vi "Lab Panel V3.4.vi"() -> ()   [LabVIEW 2013]
uses:
  <vilib>/Platform/TimedLoop/XDataNode/timing_clust.ctl
  <vilib>/Platform/TimedLoop/XDataNode/nitl_modes.ctl
  <vilib>/Platform/TimedLoop/XDataNode/wakeup.ctl
  Global 1.vi
  <vilib>/platform/TimedLoop/XDataNode/XDataNode.xnode
  <vilib>/Platform/TimedLoop/XDataNode/XDNodeRunTimeDep.lvlib
panel:
  out "TEMP update":bool
  out "AI update":bool
  in  "stop":bool
  in  "Tab Control 2":T1(tab)
  out "SIG LAB05-2":T2 {"PF" format="%.2f"; "AMPS" format="%.1f"}
  out "SIG LAB05-1":T2 {"PF" format="%.2f"; "AMPS" format="%.1f"}
  out "SIG LAB04-2":T2 {"PF" format="%.2f"; "AMPS" format="%.1f"}
  out "SIG LAB04-1":T2 {"PF" format="%.2f"; "AMPS" format="%.1f"}
  out "SIG LAB03-2":T2 {"PF" format="%.2f"; "AMPS" format="%.1f"}
  out "SIG LAB03-1":T2 {"PF" format="%.2f"; "AMPS" format="%.1f"}
  out "SIG LAB02-2":T2 {"PF" format="%.2f"; "AMPS" format="%.1f"}
  in  "RUN LAB01-1":bool
  in  "O/I  LAB05-1":bool
  in  "O/I  LAB05-2":bool
  in  "O/I  LAB04-1":bool
  in  "O/I  LAB04-2":bool
  in  "O/I  LAB02-1":bool
  in  "O/1  LAB02-2":bool
  in  "O/I  LAB01-2":bool
  in  "O/I  LAB01-1":bool
  in  "O/I  LAB03-1":bool
  in  "RUN LAB05-2":bool
  in  "RUN LAB05-1":bool
  in  "RUN LAB04-2":bool
  in  "RUN LAB04-1":bool
  in  "RUN LAB03-2":bool
  in  "RUN LAB03-1":bool
  in  "RUN LAB02-2":bool
  in  "RUN LAB02-1":bool
  in  "RUN LAB01-2":bool
  in  "SELECT LAB05-2":T3(radio)
  in  "SELECT LAB05-1":T3(radio)
  in  "SELECT LAB04-2":T3(radio)
  in  "SELECT LAB04-1":T3(radio)
  in  "SELECT LAB03-2":T3(radio)
  in  "SELECT LAB03-1":T3(radio)
  in  "SELECT LAB02-2":T3(radio)
  in  "SELECT LAB02-1":T3(radio)
  in  "SELECT LAB01-2":T3(radio)
  in  "SELECT LAB01-1":T3(radio)
  in  "O/I  LAB03-2":bool
  out "SIG LAB01-1":T2 {"PF" format="%.2f"; "AMPS" format="%.1f"}
  out "SIG LAB01-2":T2 {"PF" format="%.2f"; "AMPS" format="%.1f"}
  out "SIG LAB02-1":T2 {"PF" format="%.2f"; "AMPS" format="%.1f"}
  out "DISP LAB05-2":T4 {"MINS" format="%.2g"}
  out "DISP LAB05-1":T4 {"MINS" format="%.2g"}
  out "DISP LAB04-2":T4 {"MINS" format="%.2g"}
  out "DISP LAB04-1":T4 {"MINS" format="%.2g"}
  out "DISP LAB03-2":T4 {"MINS" format="%.2g"}
  out "DISP LAB03-1":T4 {"MINS" format="%.2g"}
  in  "SET LAB05-2":T5={"NAME"="", "DESCRIPTION"="", "CYCLES"=5.0, "T-RISE mins"=0.0, "T-RISE deg C"=0.0} {"CYCLES" min=5.0 step=1.0}
  in  "SET LAB05-1":T5={"NAME"="", "DESCRIPTION"="", "CYCLES"=5.0, "T-RISE mins"=0.0, "T-RISE deg C"=0.0} {"CYCLES" min=5.0 step=1.0}
  in  "SET LAB04-2":T5={"NAME"="", "DESCRIPTION"="", "CYCLES"=5.0, "T-RISE mins"=0.0, "T-RISE deg C"=0.0} {"CYCLES" min=5.0 step=1.0}
  in  "SET LAB04-1":T5={"NAME"="", "DESCRIPTION"="", "CYCLES"=5.0, "T-RISE mins"=0.0, "T-RISE deg C"=0.0} {"CYCLES" min=5.0 step=1.0}
  in  "SET LAB03-2":T5={"NAME"="", "DESCRIPTION"="", "CYCLES"=5.0, "T-RISE mins"=0.0, "T-RISE deg C"=0.0} {"CYCLES" min=5.0 step=1.0}
  in  "SET LAB03-1":T5={"NAME"="", "DESCRIPTION"="", "CYCLES"=5.0, "T-RISE mins"=0.0, "T-RISE deg C"=0.0} {"CYCLES" min=5.0 step=1.0}
  out "DISP LAB02-2":T4 {"MINS" format="%.2g"}
  out "DISP LAB02-1":T4 {"MINS" format="%.2g"}
  in  "SET LAB02-2":T5={"NAME"="", "DESCRIPTION"="", "CYCLES"=5.0, "T-RISE mins"=0.0, "T-RISE deg C"=0.0} {"CYCLES" min=5.0 step=1.0}
  in  "SET LAB02-1":T5={"NAME"="", "DESCRIPTION"="", "CYCLES"=5.0, "T-RISE mins"=0.0, "T-RISE deg C"=0.0} {"CYCLES" min=5.0 step=1.0}
  out "RESULT LAB05-2":bool
  out "RESULT LAB05-1":bool
  out "RESULT LAB04-2":bool
  out "RESULT LAB04-1":bool
  out "RESULT LAB03-2":bool
  out "RESULT LAB03-1":bool
  out "RESULT LAB02-2":bool
  out "RESULT LAB02-1":bool
  out "RESULT LAB01-2":bool
  out "RESULT LAB01-1":bool
  in  "SET LAB01-1":T5={"NAME"="", "DESCRIPTION"="", "CYCLES"=5.0, "T-RISE mins"=0.0, "T-RISE deg C"=0.0} {"CYCLES" min=5.0 step=1.0}
  in  "SET LAB01-2":T5={"NAME"="", "DESCRIPTION"="", "CYCLES"=5.0, "T-RISE mins"=0.0, "T-RISE deg C"=0.0} {"CYCLES" min=5.0 step=1.0}
  out "DISP LAB01-1":T4 {"MINS" format="%.2g"}
  out "DISP LAB01-2":T4 {"MINS" format="%.2f"}
  out "TEMP RISE LAB05-2":cluster{"TL":dbl, "TN":dbl}
  out "TEMP RISE LAB05-1":cluster{"TL":dbl, "TN":dbl}
  out "TEMP RISE LAB04-2":cluster{"TL":dbl, "TN":dbl}
  out "TEMP RISE LAB04-1":cluster{"TL":dbl, "TN":dbl}
  out "TEMP RISE LAB03-2":cluster{"TL":dbl, "TN":dbl}
  out "TEMP RISE LAB03-1":cluster{"TL":dbl, "TN":dbl}
  out "TEMP RISE LAB02-2":cluster{"TL":dbl, "TN":dbl}
  out "TEMP RISE LAB02-1":cluster{"TL":dbl, "TN":dbl}
  out "TEMP RISE LAB01-2":cluster{"TL":dbl, "TN":dbl}
  out "TEMP RISE LAB01-1":cluster{"TL":dbl, "TN":dbl}
  in  "JIG OFF TIME (S)":dbl=2.0 min=2.0 max=10.0 step=0.5 format="%.1g"
  in  "JIG ON TIME (S)":dbl=1.0 min=1.0 max=10.0 step=0.5 format="%.1g"
  out "JIG LAB05-2":bool
  out "JIG LAB05-1":bool
  out "JIG LAB04-2":bool
  out "JIG LAB04-1":bool
  out "JIG LAB03-2":bool
  out "JIG LAB03-1":bool
  out "JIG LAB02-2":bool
  out "JIG LAB02-1":bool
  out "JIG LAB01-2":bool
  out "JIG LAB01-1":bool
  out "TEMP START LAB01-1":cluster{"TL":dbl, "TN":dbl}
  out "TEMP START LAB02-1":cluster{"TL":dbl, "TN":dbl}
  out "TEMP START LAB03-1":cluster{"TL":dbl, "TN":dbl}
  out "TEMP START LAB04-1":cluster{"TL":dbl, "TN":dbl}
  out "TEMP START LAB01-2":cluster{"TL":dbl, "TN":dbl}
  out "TEMP START LAB02-2":cluster{"TL":dbl, "TN":dbl}
  out "TEMP START LAB03-2":cluster{"TL":dbl, "TN":dbl}
  out "TEMP START LAB04-2":cluster{"TL":dbl, "TN":dbl}
  out "TEMP START LAB05-2":cluster{"TL":dbl, "TN":dbl}
  out "TEMP START LAB05-1":cluster{"TL":dbl, "TN":dbl}
  in  "MAIL SETTINGS":T6
  out "MAIL REPORT":string
  in  "TO (string):":string
  in  "Send Mail Now":bool
  in  "Auto Mail Send":bool
  in  "Network Directory":path
  out "CAL LAB01":T7 {"2 (TN) cal" min=0.0 step=0.01 format="%.2f"; "2 (TL) cal" min=0.0 step=0.01 format="%.2f"; "2 (PF) cal" min=0.0 step=0.01 format="%.2f"; "2 (V) cal" min=0.0 step=0.01 format="%.2f"; "2 (A) cal" min=0.0 step=0.01 format="%.2f"; "1 (TN) cal" min=0.0 step=0.01 format="%.2f"; "1 (TL) cal" min=0.0 step=0.01 format="%.2f"; "1 (PF) cal" min=0.0 step=0.01 format="%.2f"; "1 (V) cal" min=0.0 step=0.01 format="%.2f"; "1  (A) cal" min=0.0 step=0.01 format="%.2f"}
  out "CAL LAB03":T7 {"2 (TN) cal" min=0.0 step=0.01 format="%.2f"; "2 (TL) cal" min=0.0 step=0.01 format="%.2f"; "2 (PF) cal" min=0.0 step=0.01 format="%.2f"; "2 (V) cal" min=0.0 step=0.01 format="%.2f"; "2 (A) cal" min=0.0 step=0.01 format="%.2f"; "1 (TN) cal" min=0.0 step=0.01 format="%.2f"; "1 (TL) cal" min=0.0 step=0.01 format="%.2f"; "1 (PF) cal" min=0.0 step=0.01 format="%.2f"; "1 (V) cal" min=0.0 step=0.01 format="%.2f"; "1  (A) cal" min=0.0 step=0.01 format="%.2f"}
  out "CAL LAB02":T8 {"2 (TN) cal" min=0.0 step=0.01 format="%.2f"; "2 (TL) cal" min=0.0 step=0.01 format="%.2f"; "2 (PF) cal" min=0.0 step=0.01 format="%.2f"; "2 (V) cal" min=0.0 step=0.01 format="%.2f"; "2 (A) cal" min=0.0 step=0.01 format="%.2f"; "1 (TN) cal" min=0.0 step=0.01 format="%.2f"; "1 (TL) cal" min=0.0 step=0.01 format="%.2f"; "1 (PF) cal" min=0.0 step=0.01 format="%.2f"; "1 (V) cal" min=0.0 step=0.01 format="%.2f"; "1 (A) cal" min=0.0 step=0.01 format="%.2f"}
  out "CAL LAB05":T7 {"2 (TN) cal" min=0.0 step=0.01 format="%.2f"; "2 (TL) cal" min=0.0 step=0.01 format="%.2f"; "2 (PF) cal" min=0.0 step=0.01 format="%.2f"; "2 (V) cal" min=0.0 step=0.01 format="%.2f"; "2 (A) cal" min=0.0 step=0.01 format="%.2f"; "1 (TN) cal" min=0.0 step=0.01 format="%.2f"; "1 (TL) cal" min=0.0 step=0.01 format="%.2f"; "1 (PF) cal" min=0.0 step=0.01 format="%.2f"; "1 (V) cal" min=0.0 step=0.01 format="%.2f"; "1  (A) cal" min=0.0 step=0.01 format="%.2f"}
  out "CAL LAB04":T7 {"2 (TN) cal" min=0.0 step=0.01 format="%.2f"; "2 (TL) cal" min=0.0 step=0.01 format="%.2f"; "2 (PF) cal" min=0.0 step=0.01 format="%.2f"; "2 (V) cal" min=0.0 step=0.01 format="%.2f"; "2 (A) cal" min=0.0 step=0.01 format="%.2f"; "1 (TN) cal" min=0.0 step=0.01 format="%.2f"; "1 (TL) cal" min=0.0 step=0.01 format="%.2f"; "1 (PF) cal" min=0.0 step=0.01 format="%.2f"; "1 (V) cal" min=0.0 step=0.01 format="%.2f"; "1  (A) cal" min=0.0 step=0.01 format="%.2f"}
  out "calibration file error out":errorcluster
  in  "CALIBRATE":bool
  in  "SHOW ADMIN PAGE":bool
  out "FAIL LAB05-2":cluster{"LO":dbl, "HI":dbl}
  out "FAIL LAB05-1":cluster{"LO":dbl, "HI":dbl}
  out "FAIL LAB04-2":cluster{"LO":dbl, "HI":dbl}
  out "FAIL LAB04-1":cluster{"LO":dbl, "HI":dbl}
  out "FAIL LAB03-2":cluster{"LO":dbl, "HI":dbl}
  out "FAIL LAB03-1":cluster{"LO":dbl, "HI":dbl}
  out "FAIL LAB02-2":cluster{"LO":dbl, "HI":dbl}
  out "FAIL LAB02-1":cluster{"LO":dbl, "HI":dbl}
  out "FAIL LAB01-2":cluster{"LO":dbl, "HI":dbl}
  out "FAIL LAB01-1":cluster{"LO":dbl, "HI":dbl}
  in  "C drive data root dir":path
  out "run lab05-2":bool
  out "run lab05-1":bool
  out "run lab04-2":bool
  out "run lab04-1":bool
  out "run lab03-2":bool
  out "run lab03-1":bool
  out "run lab02-2":bool
  out "run lab02-1":bool
  out "run lab01-2":bool
  out "run lab01-1":bool
  out "stop2":bool
  in  "Tab Control":T9(tab)
  out "LAB01-2 (GRAPH)":dynamicdata(graph)
  out "LAB01-1 (GRAPH)":dynamicdata(graph)
  out "LAB02-2 (GRAPH)":dynamicdata(graph)
  out "LAB02-1 (GRAPH)":dynamicdata(graph)
  out "LAB03-2 (GRAPH)":dynamicdata(graph)
  out "LAB03-1 (GRAPH)":dynamicdata(graph)
  out "LAB04-2 (GRAPH)":dynamicdata(graph)
  out "LAB04-1 (GRAPH)":dynamicdata(graph)
  out "LAB05-2 (GRAPH)":dynamicdata(graph)
  out "LAB05-1 (GRAPH)":dynamicdata(graph)
  out "LAB05 TEMP":T10
  out "LAB04 TEMP":T10
  out "LAB02 TEMP":T10
  out "LAB01 TEMP":T10
  out "LAB03 TEMP":T10
  out "Analog Error Array":errorcluster[](array[cluster])
  out "AI loop time":dbl format="%.6g"
  out "loops":dbl
  in  "loop  delay(mS)":dbl
  out "on loops":dbl
  out "off loops":dbl
  out "jig cycle":dbl
  out "TDMS LAB01-1":refnum<k34>
  out "data file error":errorcluster
  out "TDMS LAB02-1":refnum<k34>
  out "TDMS LAB01-2":refnum<k34>
  out "TDMS LAB02-2":refnum<k34>
  out "TDMS LAB03-1":refnum<k34>
  out "TDMS LAB03-2":refnum<k34>
  out "TDMS LAB04-1":refnum<k34>
  out "TDMS LAB04-2":refnum<k34>
  out "TDMS LAB05-1":refnum<k34>
  out "TDMS LAB05-2":refnum<k34>
  out "mail control":string
  # "LAB01"
  # "LAB02"
  # "LAB05"
  # "LAB03"
  # "LAB04"
  # "LAB01"
  # "LAB02"
  # "LAB03"
  # "LAB04"
  # "LAB05"
  # "JIG SET"
  # "(Enter recipients address seperated by comma)"
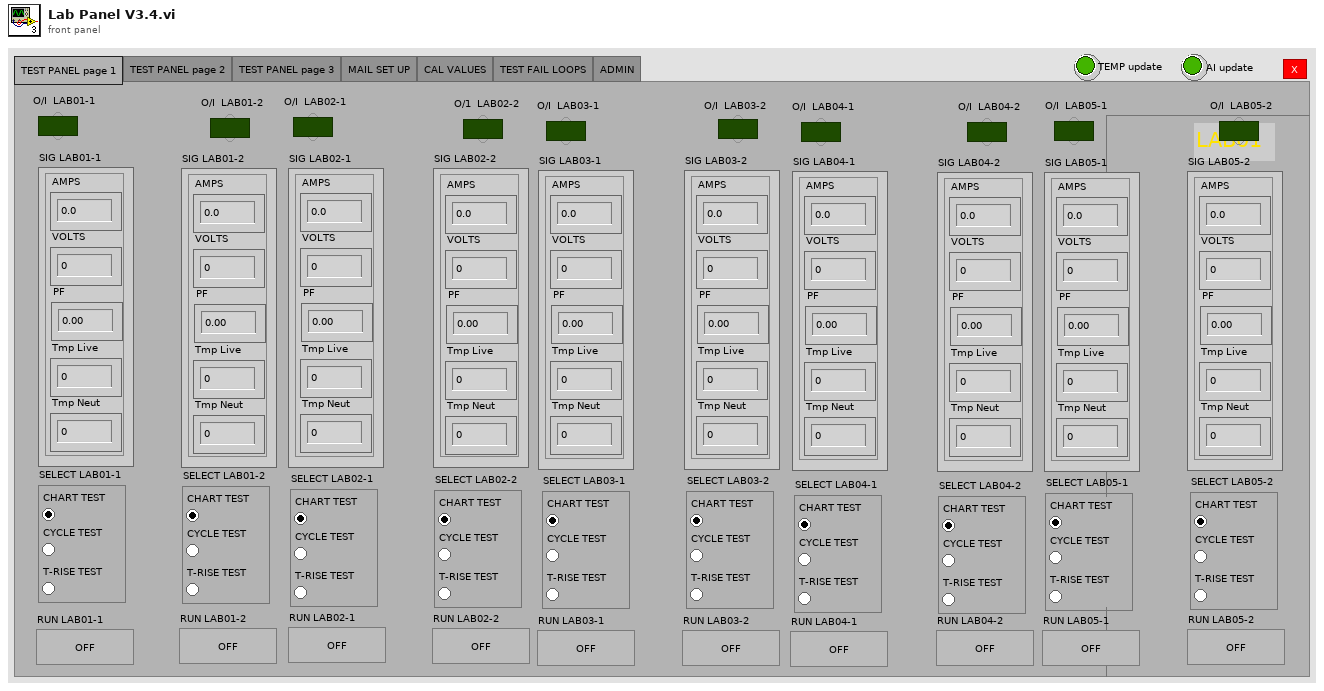
[diagram p1: front panel]
types:
  T1 = enum32{"TEST PANEL page 1", "TEST PANEL page 2", "TEST PANEL page 3", "MAIL SET UP", "CAL VALUES", "TEST FAIL LOOPS", "ADMIN"}
  T2 = cluster{"AMPS":dbl, "VOLTS":dbl, "PF":dbl, "Tmp Live":dbl, "Tmp Neut":dbl}
  T3 = enum32{"CHART TEST", "CYCLE TEST", "T-RISE TEST"}
  T4 = cluster{"CYCLE":dbl, "MINS":dbl, "STATUS":string}
  T5 = cluster{"NAME":string, "DESCRIPTION":string, "CYCLES":dbl, "T-RISE mins":dbl, "T-RISE deg C":dbl}
  T6 = cluster{"OUT SERVER ADDRESS":string, "FROM ACCOUNT":string, "USER NAME":string, "PASSWORD":string, "TEST MAIL":bool, "TEST MAIL STATUS":string, "mail error":errorcluster}
  T7 = cluster{"1  (A) cal":dbl, "1 (V) cal":dbl, "1 (PF) cal":dbl, "1 (TL) cal":dbl, "1 (TN) cal":dbl, "2 (A) cal":dbl, "2 (V) cal":dbl, "2 (PF) cal":dbl, "2 (TL) cal":dbl, "2 (TN) cal":dbl}
  T8 = cluster{"1 (A) cal":dbl, "1 (V) cal":dbl, "1 (PF) cal":dbl, "1 (TL) cal":dbl, "1 (TN) cal":dbl, "2 (A) cal":dbl, "2 (V) cal":dbl, "2 (PF) cal":dbl, "2 (TL) cal":dbl, "2 (TN) cal":dbl}
  T9 = enum32{"LAB01", "LAB02", "LAB03", "LAB04", "LAB05", "TEMPERATURE", "ERROR"}
  T10 = cluster{"T1 Live":dbl, "T1 Neut":dbl, "T2 Live":dbl, "T2 Neut":dbl, "ID":dbl, "ER":dbl}
  T11 = enum8{"Enabled", "Disabled", "Disabled and Grayed Out"}
  T12 = typedef "XDNodeRunTimeDep.lvlib/timing_clust.ctl" = cluster{"Expected End [f-1]":u64, "Actual End [f-1]":u64, "Finished Late? [f-1]":bool, "Expected End [i-1]":u64, "Actual End [i-1]":u64, "Finished Late? [i-1]":bool, "Expected Start [i]":u64, "Actual Start [i]":u64, "Expected Start [f]":u64, "Actual Start [f]":u64, "Source Name":string, "Structure Name":string, "Period":i64, "Deadline":i64, "Offset":i64, "Start":i64, "Priority":i32, "Timeout":i32, "Mode":T13, "Wakeup Reason":T14, "Error":errorcluster, "Source Type":string, "Secondary Source Type":string, "Global End Time":u64, "Global Start Time":u64, "Frame Duration":u64, "Iteration Duration":u64, "Assigned CPU":i32, "I/O Scan Engine Mode":u32}
  T13 = typedef "XDNodeRunTimeDep.lvlib/nitl_modes.ctl" = enum32{"No Change", "Process missed periods, maintain original phase", "Discard missed periods, maintain original phase", "Process missed periods, ignore original phase", "Discard missed periods, ignore original phase"}
  T14 = typedef "XDNodeRunTimeDep.lvlib/wakeup.ctl" = enum32{"Normal", "Aborted", "Asynchronous wakeup", "Timing source error", "Timed loop error", "Timeout"}
  T15 = enum16{"open", "open or create", "create or replace", "create", "open (read-only)"}
  T16 = enum16{"open", "replace", "create", "open or create", "replace or create", "replace or create with confirmation"}
  T17 = cluster{"SET LAB01-1":cluster{"NAME":string, "DESCRIPTION":string, "CYCLES":dbl, "T-RISE mins":dbl, "T-RISE deg C":dbl}, "SET LAB01-2":cluster{"NAME":string, "DESCRIPTION":string, "CYCLES":dbl, "T-RISE mins":dbl, "T-RISE deg C":dbl}, "SET LAB02-1":cluster{"NAME":string, "DESCRIPTION":string, "CYCLES":dbl, "T-RISE mins":dbl, "T-RISE deg C":dbl}, "SET LAB02-2":cluster{"NAME":string, "DESCRIPTION":string, "CYCLES":dbl, "T-RISE mins":dbl, "T-RISE deg C":dbl}, "SET LAB03-1":cluster{"NAME":string, "DESCRIPTION":string, "CYCLES":dbl, "T-RISE mins":dbl, "T-RISE deg C":dbl}, "SET LAB03-2":cluster{"NAME":string, "DESCRIPTION":string, "CYCLES":dbl, "T-RISE mins":dbl, "T-RISE deg C":dbl}, "SET LAB04-1":cluster{"NAME":string, "DESCRIPTION":string, "CYCLES":dbl, "T-RISE mins":dbl, "T-RISE deg C":dbl}, "SET LAB04-2":cluster{"NAME":string, "DESCRIPTION":string, "CYCLES":dbl, "T-RISE mins":dbl, "T-RISE deg C":dbl}, "SET LAB05-1":cluster{"NAME":string, "DESCRIPTION":string, "CYCLES":dbl, "T-RISE mins":dbl, "T-RISE deg C":dbl}, "SET LAB05-2":cluster{"NAME":string, "DESCRIPTION":string, "CYCLES":dbl, "T-RISE mins":dbl, "T-RISE deg C":dbl}, "Network Directory":path, "C drive data root dir":path}
  T18 = cluster{"MAIL SETTINGS":cluster{"OUT SERVER ADDRESS":string, "FROM ACCOUNT":string, "USER NAME":string, "PASSWORD":string, "TEST MAIL":bool, "TEST MAIL STATUS":string, "mail error":errorcluster}, "Auto Mail Send":bool, string}
  T19 = cluster{"T1":dbl, "T2":dbl, "T3":dbl, "T4":dbl, "ID":dbl, "ER":dbl}
  T20 = cluster{"LAB01-1 (A)":dbl, "LAB01-1 (V)":dbl, "LAB01-1 (PF)":dbl, "LAB01-2 (A)":dbl, "LAB01-2 (V)":dbl, "LAB01-2 (PF)":dbl}
  T21 = cluster{"LAB02-1 (A)":dbl, "LAB02-1 (V)":dbl, "LAB02-1 (PF)":dbl, "LAB02-2 (A)":dbl, "LAB02-2 (V)":dbl, "LAB02-2 (PF)":dbl}
  T22 = cluster{"LAB03-1 (A)":dbl, "LAB03-1 (V)":dbl, "LAB03-1 (PF)":dbl, "LAB03-2 (A)":dbl, "LAB03-2 (V)":dbl, "LAB03-2 (PF)":dbl}
  T23 = cluster{"LAB04-1 (A)":dbl, "LAB04-1 (V)":dbl, "LAB04-1 (PF)":dbl, "LAB04-2 (A)":dbl, "LAB04-2 (V)":dbl, "LAB04-2 (PF)":dbl}
  T24 = cluster{"LAB05-1 (A)":dbl, "LAB05-1 (V)":dbl, "LAB05-1 (PF)":dbl, "LAB05-2 (A)":dbl, "LAB05-2 (V)":dbl, "LAB05-2 (PF)":dbl}
  T25 = cluster{"FAIL LAB01-1":cluster{"LO":dbl, "HI":dbl}, "SIG LAB01-1":cluster{"AMPS":dbl, "VOLTS":dbl, "PF":dbl, "Tmp Live":dbl, "Tmp Neut":dbl}, "TEMP START LAB01-1":cluster{"TL":dbl, "TN":dbl}, "DISP LAB01-1":cluster{"CYCLE":dbl, "MINS":dbl, "STATUS":string}, "SET LAB01-1":cluster{"NAME":string, "DESCRIPTION":string, "CYCLES":dbl, "T-RISE mins":dbl, "T-RISE deg C":dbl}, "TDMS LAB01-1":refnum<k34>}
  T26 = cluster{"FAIL LAB01-2":cluster{"LO":dbl, "HI":dbl}, "SIG LAB01-2":cluster{"AMPS":dbl, "VOLTS":dbl, "PF":dbl, "Tmp Live":dbl, "Tmp Neut":dbl}, "TEMP START LAB01-2":cluster{"TL":dbl, "TN":dbl}, "DISP LAB01-2":cluster{"CYCLE":dbl, "MINS":dbl, "STATUS":string}, "SET LAB01-2":cluster{"NAME":string, "DESCRIPTION":string, "CYCLES":dbl, "T-RISE mins":dbl, "T-RISE deg C":dbl}, "TDMS LAB01-2":refnum<k34>}
  T27 = cluster{"FAIL LAB02-1":cluster{"LO":dbl, "HI":dbl}, "SIG LAB02-1":cluster{"AMPS":dbl, "VOLTS":dbl, "PF":dbl, "Tmp Live":dbl, "Tmp Neut":dbl}, "TEMP START LAB02-1":cluster{"TL":dbl, "TN":dbl}, "DISP LAB02-1":cluster{"CYCLE":dbl, "MINS":dbl, "STATUS":string}, "SET LAB02-1":cluster{"NAME":string, "DESCRIPTION":string, "CYCLES":dbl, "T-RISE mins":dbl, "T-RISE deg C":dbl}, "TDMS LAB02-1":refnum<k34>}
  T28 = cluster{"FAIL LAB02-2":cluster{"LO":dbl, "HI":dbl}, "SIG LAB02-2":cluster{"AMPS":dbl, "VOLTS":dbl, "PF":dbl, "Tmp Live":dbl, "Tmp Neut":dbl}, "TEMP START LAB02-2":cluster{"TL":dbl, "TN":dbl}, "DISP LAB02-2":cluster{"CYCLE":dbl, "MINS":dbl, "STATUS":string}, "SET LAB02-2":cluster{"NAME":string, "DESCRIPTION":string, "CYCLES":dbl, "T-RISE mins":dbl, "T-RISE deg C":dbl}, "TDMS LAB02-2":refnum<k34>}
  T29 = cluster{"FAIL LAB03-1":cluster{"LO":dbl, "HI":dbl}, "SIG LAB03-1":cluster{"AMPS":dbl, "VOLTS":dbl, "PF":dbl, "Tmp Live":dbl, "Tmp Neut":dbl}, "TEMP START LAB03-1":cluster{"TL":dbl, "TN":dbl}, "DISP LAB03-1":cluster{"CYCLE":dbl, "MINS":dbl, "STATUS":string}, "SET LAB03-1":cluster{"NAME":string, "DESCRIPTION":string, "CYCLES":dbl, "T-RISE mins":dbl, "T-RISE deg C":dbl}, "TDMS LAB03-1":refnum<k34>}
  T30 = cluster{"FAIL LAB03-2":cluster{"LO":dbl, "HI":dbl}, "SIG LAB03-2":cluster{"AMPS":dbl, "VOLTS":dbl, "PF":dbl, "Tmp Live":dbl, "Tmp Neut":dbl}, "TEMP START LAB03-2":cluster{"TL":dbl, "TN":dbl}, "DISP LAB03-2":cluster{"CYCLE":dbl, "MINS":dbl, "STATUS":string}, "SET LAB03-2":cluster{"NAME":string, "DESCRIPTION":string, "CYCLES":dbl, "T-RISE mins":dbl, "T-RISE deg C":dbl}, "TDMS LAB03-2":refnum<k34>}
  T31 = cluster{"FAIL LAB04-1":cluster{"LO":dbl, "HI":dbl}, "SIG LAB04-1":cluster{"AMPS":dbl, "VOLTS":dbl, "PF":dbl, "Tmp Live":dbl, "Tmp Neut":dbl}, "TEMP START LAB04-1":cluster{"TL":dbl, "TN":dbl}, "DISP LAB04-1":cluster{"CYCLE":dbl, "MINS":dbl, "STATUS":string}, "SET LAB04-1":cluster{"NAME":string, "DESCRIPTION":string, "CYCLES":dbl, "T-RISE mins":dbl, "T-RISE deg C":dbl}, "TDMS LAB04-1":refnum<k34>}
  T32 = cluster{"FAIL LAB04-2":cluster{"LO":dbl, "HI":dbl}, "SIG LAB04-2":cluster{"AMPS":dbl, "VOLTS":dbl, "PF":dbl, "Tmp Live":dbl, "Tmp Neut":dbl}, "TEMP START LAB04-2":cluster{"TL":dbl, "TN":dbl}, "DISP LAB04-2":cluster{"CYCLE":dbl, "MINS":dbl, "STATUS":string}, "SET LAB04-2":cluster{"NAME":string, "DESCRIPTION":string, "CYCLES":dbl, "T-RISE mins":dbl, "T-RISE deg C":dbl}, "TDMS LAB04-2":refnum<k34>}
  T33 = cluster{"FAIL LAB05-1":cluster{"LO":dbl, "HI":dbl}, "SIG LAB05-1":cluster{"AMPS":dbl, "VOLTS":dbl, "PF":dbl, "Tmp Live":dbl, "Tmp Neut":dbl}, "TEMP START LAB05-1":cluster{"TL":dbl, "TN":dbl}, "DISP LAB05-1":cluster{"CYCLE":dbl, "MINS":dbl, "STATUS":string}, "SET LAB05-1":cluster{"NAME":string, "DESCRIPTION":string, "CYCLES":dbl, "T-RISE mins":dbl, "T-RISE deg C":dbl}, "TDMS LAB05-1":refnum<k34>}
  T34 = cluster{"FAIL LAB05-2":cluster{"LO":dbl, "HI":dbl}, "SIG LAB05-2":cluster{"AMPS":dbl, "VOLTS":dbl, "PF":dbl, "Tmp Live":dbl, "Tmp Neut":dbl}, "TEMP START LAB05-2":cluster{"TL":dbl, "TN":dbl}, "DISP LAB05-2":cluster{"CYCLE":dbl, "MINS":dbl, "STATUS":string}, "SET LAB05-2":cluster{"NAME":string, "DESCRIPTION":string, "CYCLES":dbl, "T-RISE mins":dbl, "T-RISE deg C":dbl}, "TDMS LAB05-2":refnum<k34>}
  T35 = cluster{"MAIL SETTINGS":cluster{"OUT SERVER ADDRESS":string, "FROM ACCOUNT":string, "USER NAME":string, "PASSWORD":string, "TEST MAIL":bool, "TEST MAIL STATUS":string, "mail error":errorcluster}, "Auto Mail Send":bool, "TO (string):":string}
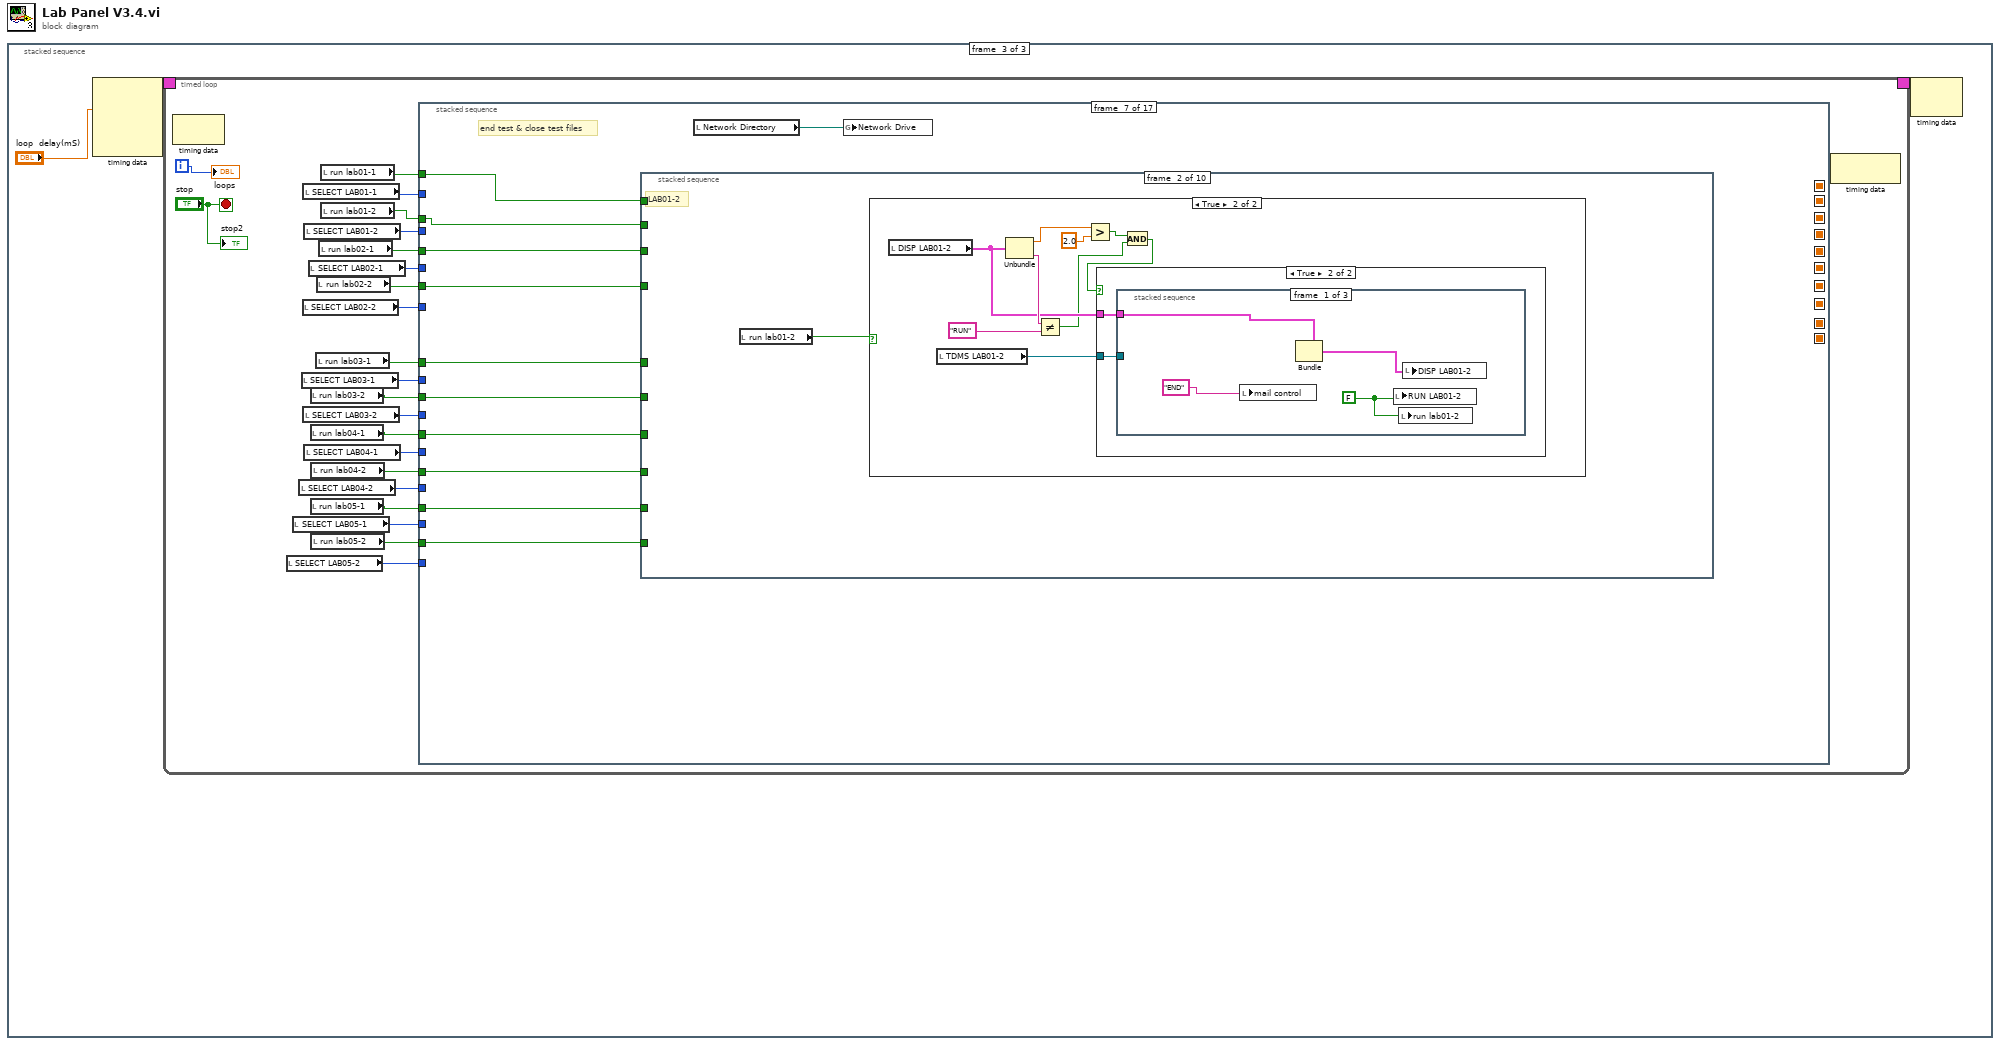
[diagram p0: block diagram]
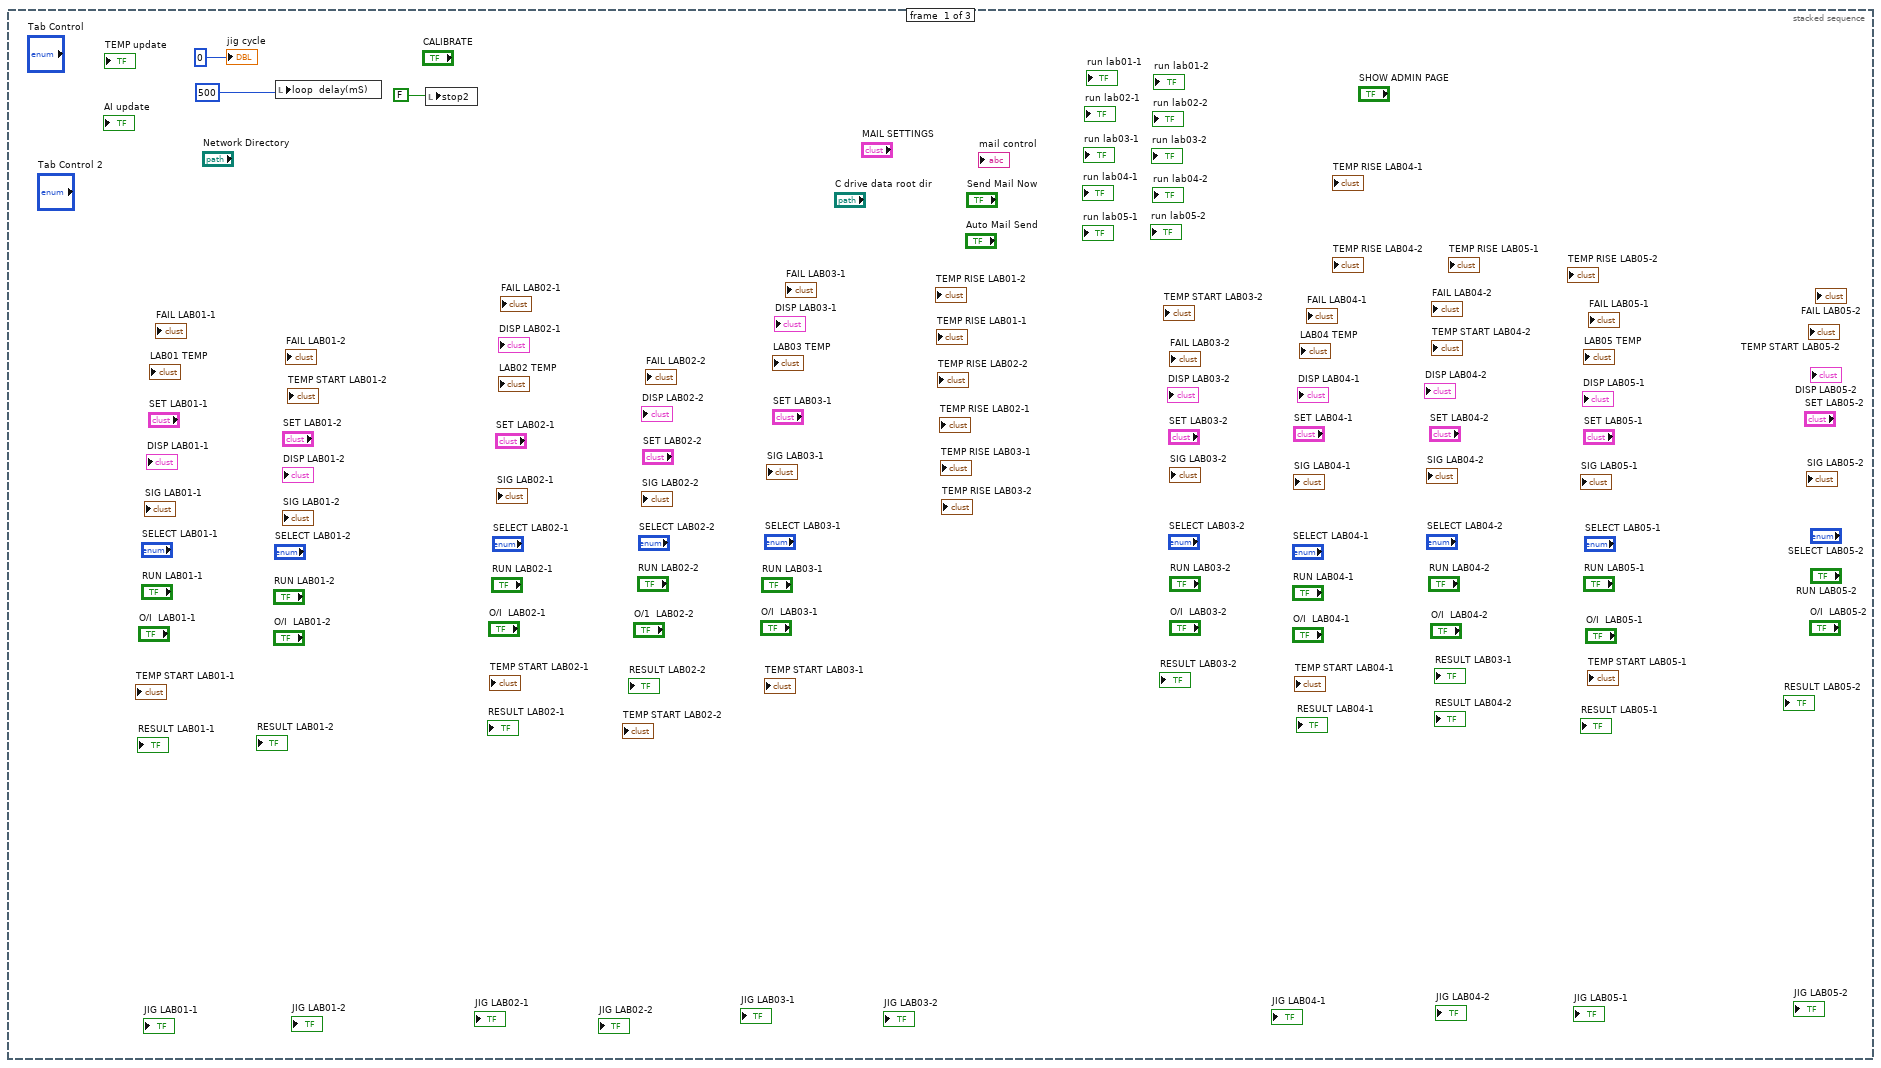
[diagram p2: hidden frame]
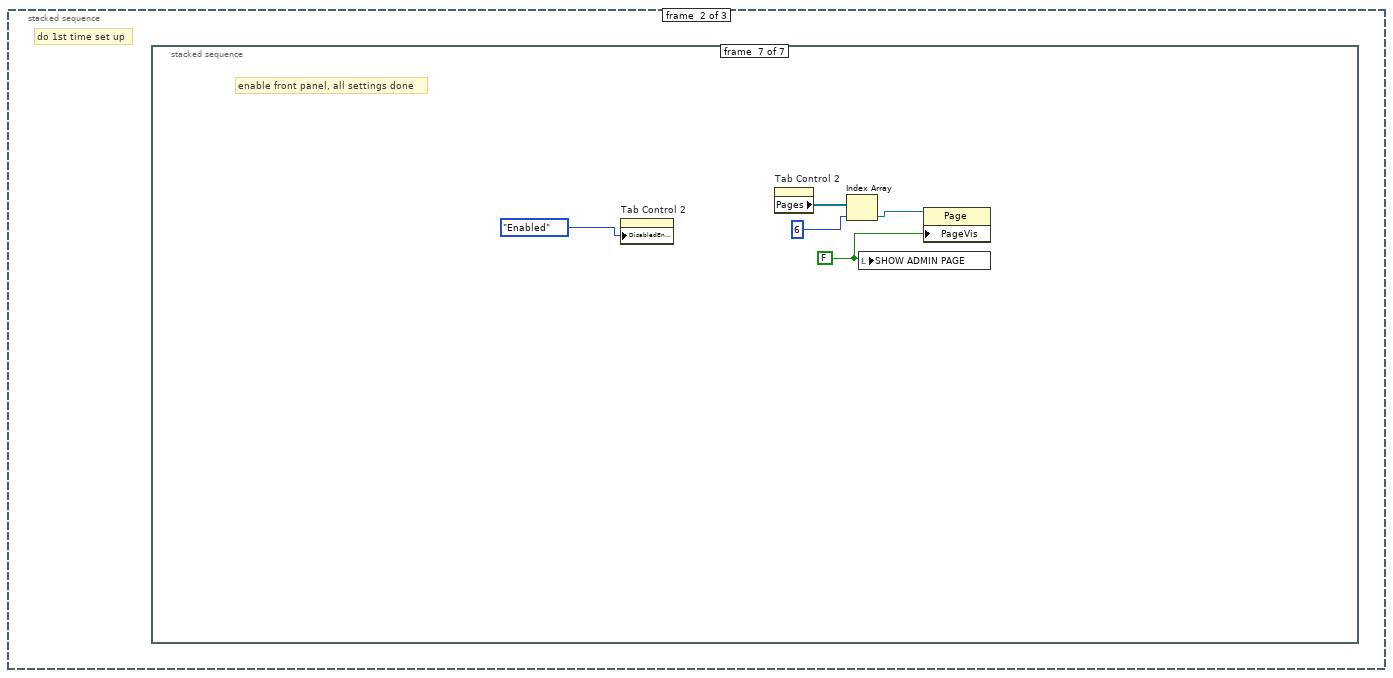
[diagram p3: hidden frame]
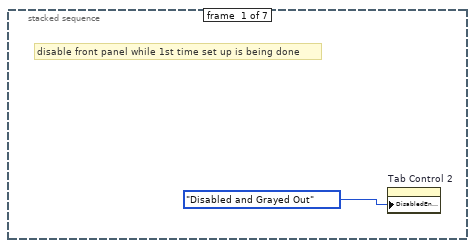
[diagram p4: hidden frame]
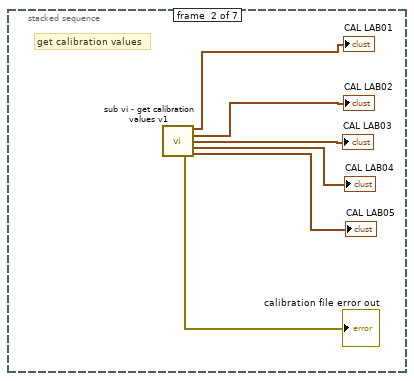
[diagram p5: hidden frame]
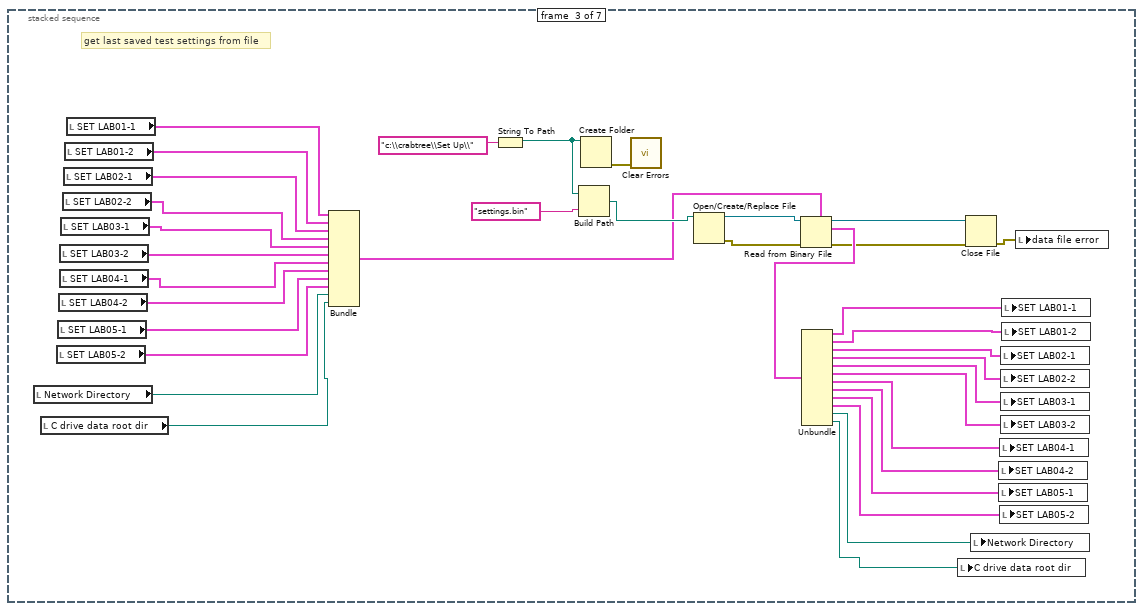
[diagram p6: hidden frame]
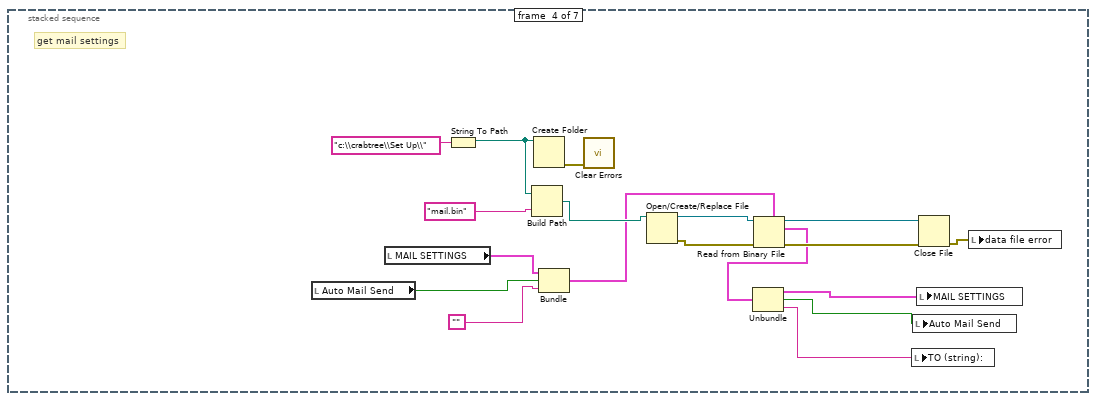
[diagram p7: hidden frame]
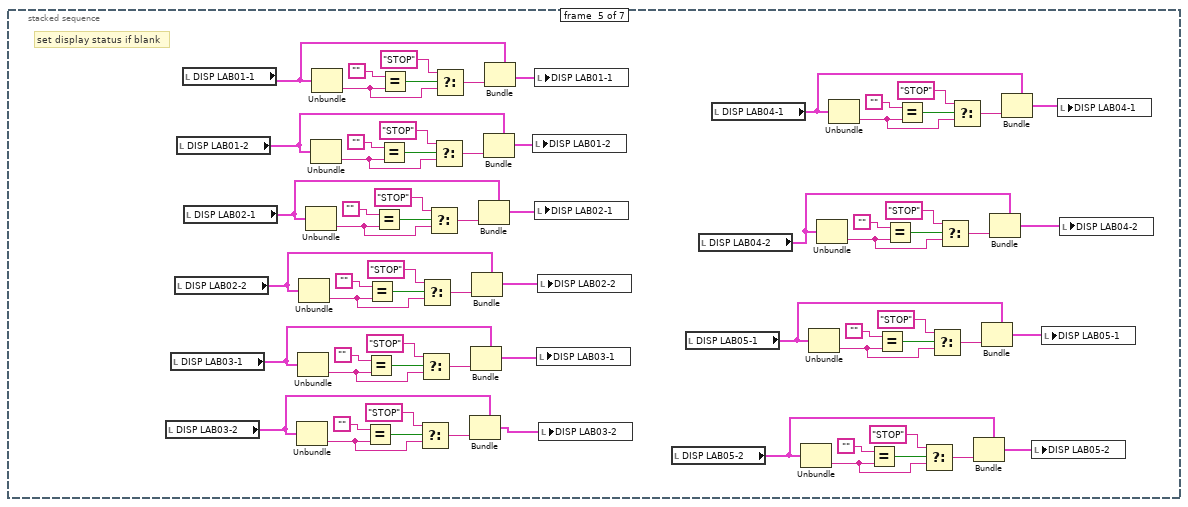
[diagram p8: hidden frame]
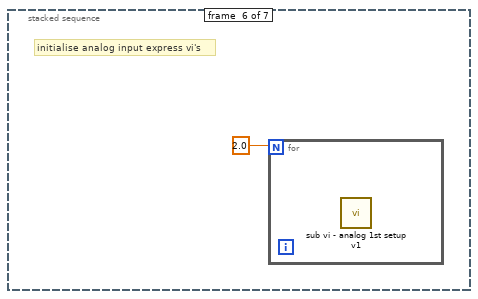
[diagram p9: hidden frame]
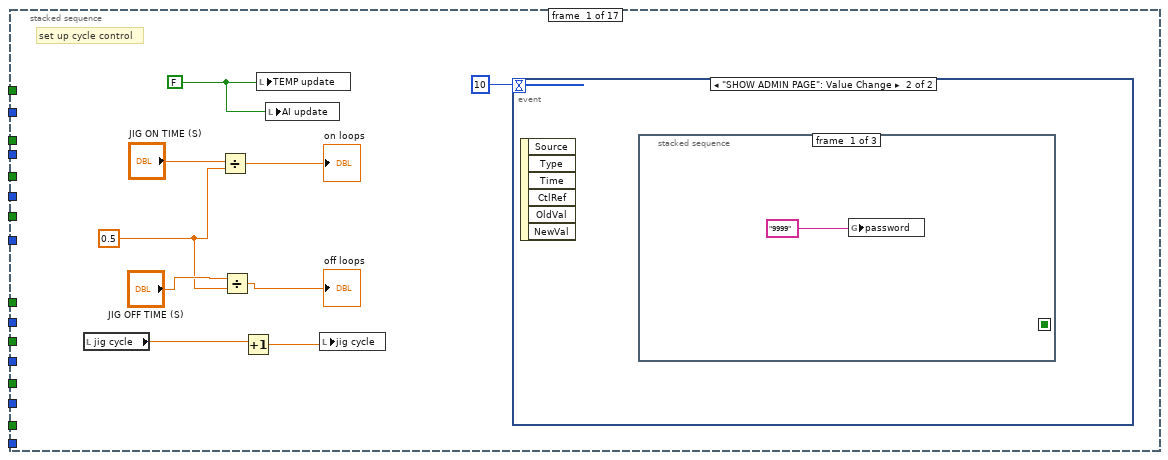
[diagram p10: hidden frame]
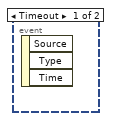
[diagram p11: hidden frame]
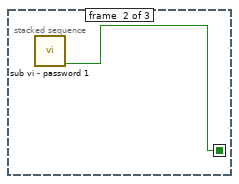
[diagram p12: hidden frame]
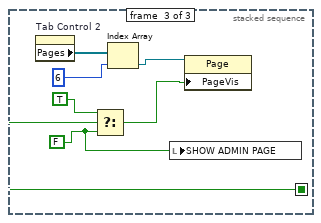
[diagram p13: hidden frame]
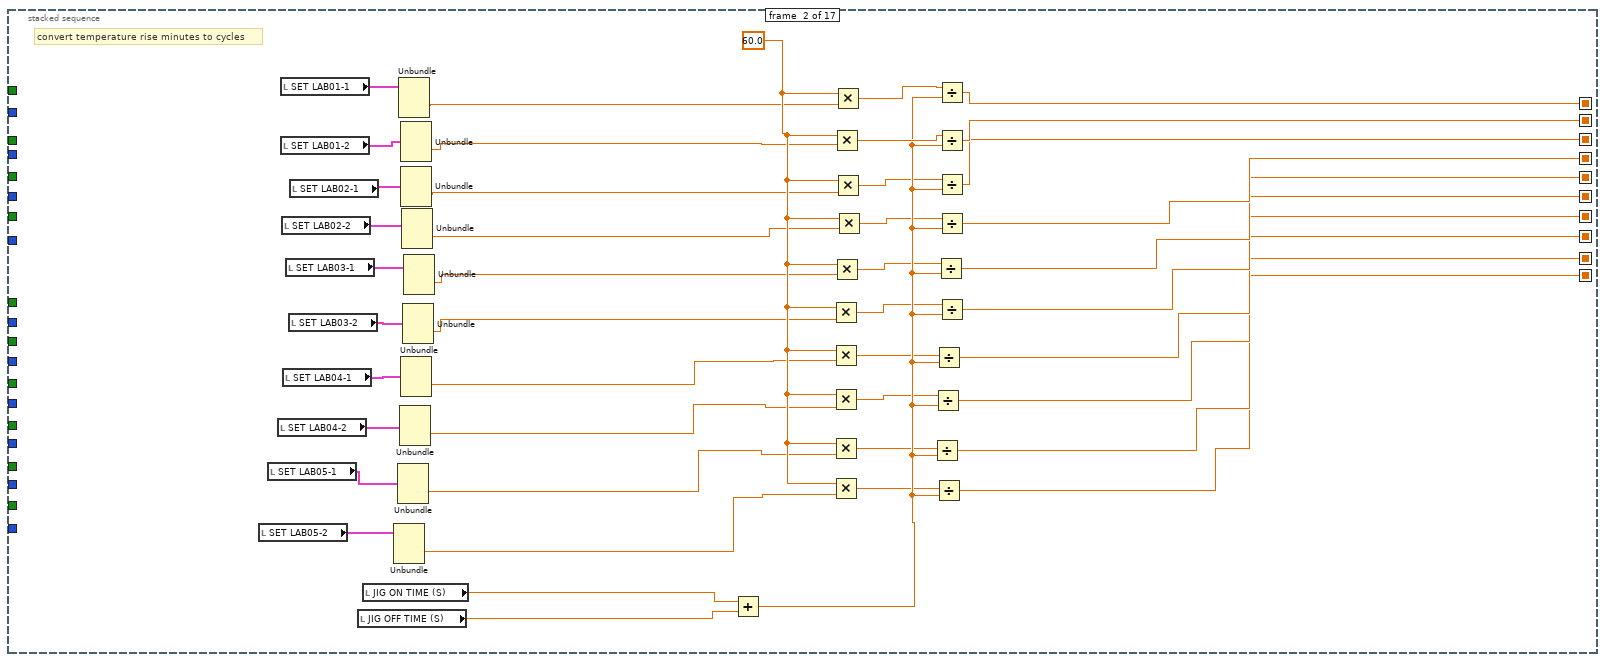
[diagram p14: hidden frame]
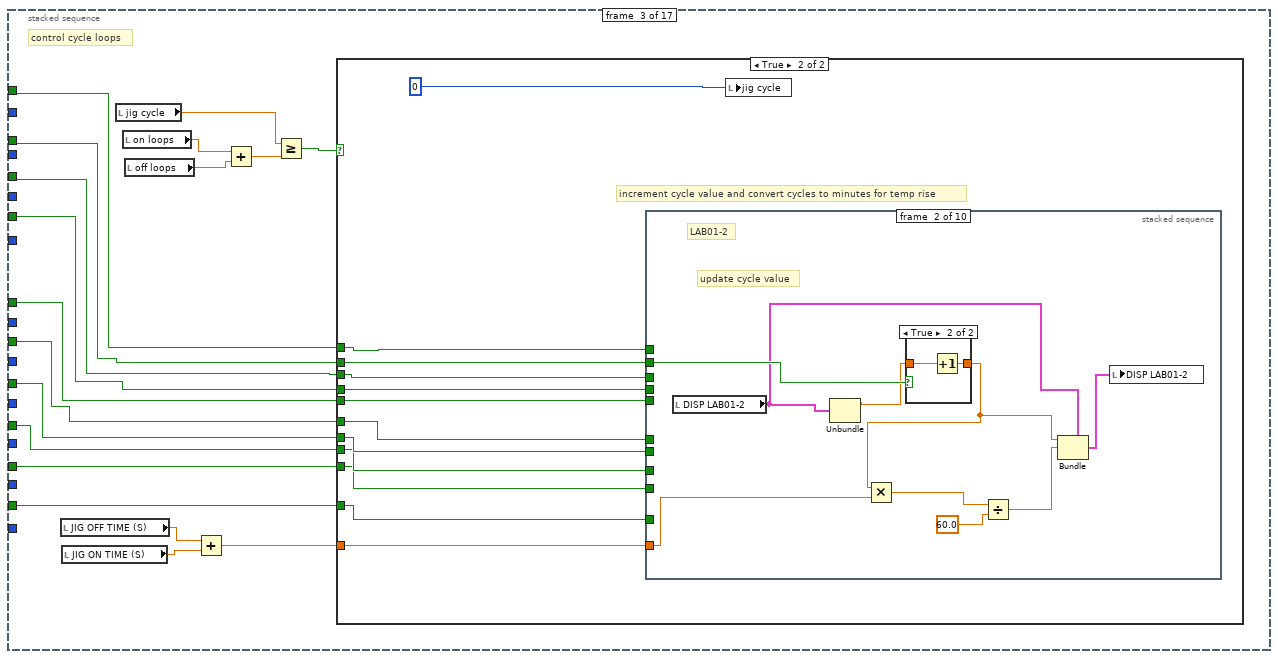
[diagram p15: hidden frame]
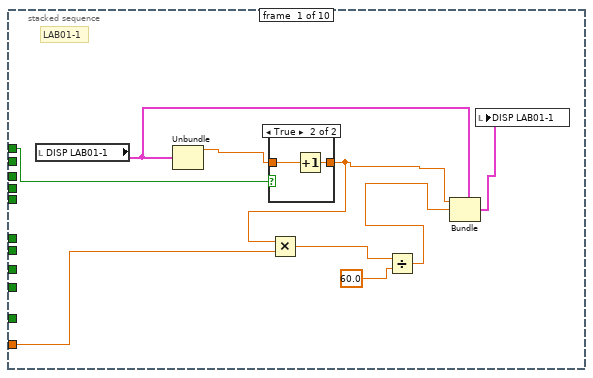
[diagram p17: hidden frame]
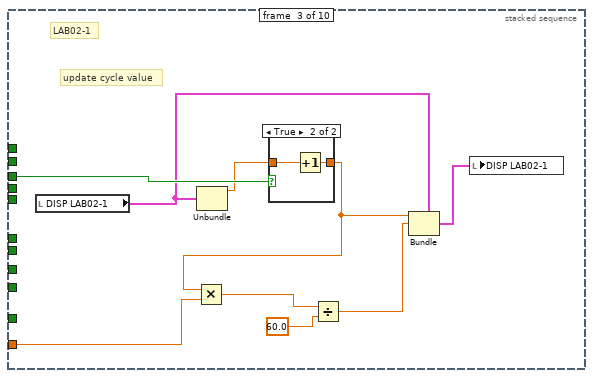
[diagram p20: hidden frame]
diagram:
  n1 = stacked-sequence {
    frame #0 {
      n2 = local write "loop  delay(mS)"(500) -> ()
      n3 = local write "stop2"(FALSE) -> ()
      "jig cycle" <- 0
    }
    frame #1 {
      # "do 1st time set up"
      n4 = stacked-sequence {
        frame #0 {
          # "disable front panel while 1st time set up is being done"
          n5 = property on="Tab Control 2" class="TabCtl (strict)"("DisabledEnum"=T11."Disabled and Grayed Out" ("Disabled")) -> ()  [unwired: 2 in, 2 out]
        }
        frame #1 {
          # "get calibration values"
          n6 = call "sub vi - get calibration values v1.vi"() -> ("LAB01 (CAL)"=→"CAL LAB01":T7, "LAB02 (CAL)"=→"CAL LAB02":T8, "LAB03 (CAL)"=→"CAL LAB03":T7, "LAB04 (CAL)"=→"CAL LAB04":T7, "calibration file error out"=→"calibration file error out":errorcluster, "LAB05 (CAL)"=→"CAL LAB05":T7)  [unwired: 10 in]
        }
        frame #2 {
          # "get last saved test settings from file"
          n7 = local read "Network Directory"() -> (w13:path)
          n8 = local read "C drive data root dir"() -> (w11:path)
          n9 = local read "SET LAB05-2"() -> (w43:T5)
          n10 = local read "SET LAB05-1"() -> (w44:T5)
          n11 = local read "SET LAB04-2"() -> (w45:T5)
          n12 = local read "SET LAB03-2"() -> (w42:T5)
          n13 = local read "SET LAB04-1"() -> (w46:T5)
          n14 = local read "SET LAB03-1"() -> (w41:T5)
          n15 = local read "SET LAB02-2"() -> (w40:T5)
          n16 = local read "SET LAB02-1"() -> (w39:T5)
          n17 = local read "SET LAB01-2"() -> (w38:T5)
          n18 = local read "SET LAB01-1"() -> (w37:T5)
          n19 = Bundle("SET LAB01-1"=w37, "SET LAB01-2"=w38, "SET LAB02-1"=w39, "SET LAB02-2"=w40, "SET LAB03-1"=w41, "SET LAB03-2"=w42, "SET LAB04-1"=w46, "SET LAB04-2"=w45, "SET LAB05-1"=w44, "SET LAB05-2"=w43, "Network Directory"=w13, "C drive data root dir"=w11) -> (w30:T17)  [unwired: 1 in]
          n20 = String To Path(string="c:\\crabtree\\Set Up\\") -> (path=w34:path)
          n21 = Build Path(base path=w34, name or relative path="settings.bin") -> (appended path=w32:path)
          n22 = Create Folder(path (use dialog)=w34) -> (error out=w36:errorcluster)  [unwired: 2 in, 2 out]
          n23 = call <vilib>:"Clear Errors.vi"("error in (no error)"=w36) -> ()  [unwired: 6 in, 1 out]
          n24 = Open/Create/Replace File(file path (use dialog)=w32) -> (refnum out=w29:refnum<file>, error out=w31:errorcluster)  [unwired: 5 in, 1 out]
          n25 = Read from Binary File(5:w30, 8:w31, 11:w29) -> (0:w26:errorcluster, 2:w28:T17, 3:w27:refnum<file>)  [unwired: 3 in, 1 out]
          n26 = Unbundle(w28) -> ("SET LAB01-1"=w24:T5, "SET LAB01-2"=w23:T5, "SET LAB02-1"=w22:T5, "SET LAB02-2"=w21:T5, "SET LAB03-1"=w20:T5, "SET LAB03-2"=w19:T5, "SET LAB04-1"=w18:T5, "SET LAB04-2"=w17:T5, "SET LAB05-1"=w16:T5, "SET LAB05-2"=w15:T5, "Network Directory"=w14:path, "C drive data root dir"=w12:path)
          n27 = local write "C drive data root dir"(w12) -> ()
          n28 = Close File(refnum=w27, error in=w26) -> (error out=w25:errorcluster)  [unwired: 1 out]
          n29 = local write "Network Directory"(w14) -> ()
          n30 = local write "SET LAB04-2"(w17) -> ()
          n31 = local write "SET LAB05-1"(w16) -> ()
          n32 = local write "SET LAB04-1"(w18) -> ()
          n33 = local write "SET LAB05-2"(w15) -> ()
          n34 = local write "SET LAB02-1"(w22) -> ()
          n35 = local write "SET LAB02-2"(w21) -> ()
          n36 = local write "SET LAB03-1"(w20) -> ()
          n37 = local write "SET LAB03-2"(w19) -> ()
          n38 = local write "SET LAB01-1"(w24) -> ()
          n39 = local write "SET LAB01-2"(w23) -> ()
          n40 = local write "data file error"(w25) -> ()
        }
        frame #3 {
          # "get mail settings"
          n41 = local read "Auto Mail Send"() -> (w50:bool)
          n42 = local read "MAIL SETTINGS"() -> (w54:T6)
          n43 = String To Path(string="c:\\crabtree\\Set Up\\") -> (path=w62:path)
          n44 = Build Path(base path=w62, name or relative path="mail.bin") -> (appended path=w60:path)
          n45 = Create Folder(path (use dialog)=w62) -> (error out=w64:errorcluster)  [unwired: 2 in, 2 out]
          n46 = Bundle("MAIL SETTINGS"=w54, "Auto Mail Send"=w50, "") -> (w53:T18)  [unwired: 1 in]
          n47 = call <vilib>:"Clear Errors.vi"("error in (no error)"=w64) -> ()  [unwired: 6 in, 1 out]
          n48 = Open/Create/Replace File(file path (use dialog)=w60) -> (refnum out=w58:refnum<file>, error out=w59:errorcluster)  [unwired: 5 in, 1 out]
          n49 = Read from Binary File(5:w53, 8:w59, 11:w58) -> (0:w56:errorcluster, 2:w52:T18, 3:w57:refnum<file>)  [unwired: 3 in, 1 out]
          n50 = Unbundle(w52) -> ("MAIL SETTINGS"=w51:T6, "Auto Mail Send"=w49:bool, w48:string)
          n51 = local write "TO (string):"(w48) -> ()
          n52 = local write "Auto Mail Send"(w49) -> ()
          n53 = local write "MAIL SETTINGS"(w51) -> ()
          n54 = Close File(refnum=w57, error in=w56) -> (error out=w55:errorcluster)  [unwired: 1 out]
          n55 = local write "data file error"(w55) -> ()
        }
        frame #4 {
          # "set display status if blank"
          n56 = local read "DISP LAB03-2"() -> (w94:T4)
          n57 = local read "DISP LAB03-1"() -> (w101:T4)
          n58 = local read "DISP LAB02-2"() -> (w108:T4)
          n59 = local read "DISP LAB01-2"() -> (w121:T4)
          n60 = local read "DISP LAB01-1"() -> (w130:T4)
          n61 = local read "DISP LAB02-1"() -> (w115:T4)
          n62 = Unbundle(w94) -> ("STATUS"=w96:string)  [unwired: 2 out]
          n63 = Unbundle(w101) -> ("STATUS"=w103:string)  [unwired: 2 out]
          n64 = Unbundle(w108) -> ("STATUS"=w110:string)  [unwired: 2 out]
          n65 = Unbundle(w115) -> ("STATUS"=w117:string)  [unwired: 2 out]
          n66 = Unbundle(w121) -> ("STATUS"=w124:string)  [unwired: 2 out]
          n67 = Unbundle(w130) -> ("STATUS"=w131:string)  [unwired: 2 out]
          n68 = Equal?(x="", y=w96) -> (x = y?=w98:bool)
          n69 = Equal?(x="", y=w103) -> (x = y?=w105:bool)
          n70 = Equal?(x="", y=w110) -> (x = y?=w112:bool)
          n71 = Equal?(x="", y=w117) -> (x = y?=w119:bool)
          n72 = Equal?(x="", y=w124) -> (x = y?=w126:bool)
          n73 = Equal?(x="", y=w131) -> (x = y?=w133:bool)
          n74 = Select(t="STOP", s=w98, f=w96) -> (s? t:f=w95:string)
          n75 = Select(t="STOP", s=w105, f=w103) -> (s? t:f=w102:string)
          n76 = Select(t="STOP", s=w112, f=w110) -> (s? t:f=w109:string)
          n77 = Select(t="STOP", s=w119, f=w117) -> (s? t:f=w116:string)
          n78 = Select(t="STOP", s=w126, f=w124) -> (s? t:f=w123:string)
          n79 = Select(t="STOP", s=w133, f=w131) -> (s? t:f=w129:string)
          n80 = Bundle(cluster=w94, "STATUS"=w95) -> (w93:T4)  [unwired: 2 in]
          n81 = Bundle(cluster=w101, "STATUS"=w102) -> (w100:T4)  [unwired: 2 in]
          n82 = Bundle(cluster=w108, "STATUS"=w109) -> (w107:T4)  [unwired: 2 in]
          n83 = Bundle(cluster=w115, "STATUS"=w116) -> (w114:T4)  [unwired: 2 in]
          n84 = Bundle(cluster=w121, "STATUS"=w123) -> (w122:T4)  [unwired: 2 in]
          n85 = Bundle(cluster=w130, "STATUS"=w129) -> (w128:T4)  [unwired: 2 in]
          n86 = local write "DISP LAB01-2"(w122) -> ()
          n87 = local write "DISP LAB01-1"(w128) -> ()
          n88 = local write "DISP LAB02-1"(w114) -> ()
          n89 = local write "DISP LAB03-1"(w100) -> ()
          n90 = local write "DISP LAB02-2"(w107) -> ()
          n91 = local write "DISP LAB03-2"(w93) -> ()
          n92 = local read "DISP LAB05-2"() -> (w66:T4)
          n93 = local read "DISP LAB05-1"() -> (w73:T4)
          n94 = local read "DISP LAB04-2"() -> (w75:T4)
          n95 = local read "DISP LAB04-1"() -> (w77:T4)
          n96 = Unbundle(w66) -> ("STATUS"=w68:string)  [unwired: 2 out]
          n97 = Unbundle(w73) -> ("STATUS"=w79:string)  [unwired: 2 out]
          n98 = Unbundle(w75) -> ("STATUS"=w84:string)  [unwired: 2 out]
          n99 = Unbundle(w77) -> ("STATUS"=w89:string)  [unwired: 2 out]
          n100 = Equal?(x="", y=w68) -> (x = y?=w70:bool)
          n101 = Equal?(x="", y=w79) -> (x = y?=w81:bool)
          n102 = Equal?(x="", y=w84) -> (x = y?=w86:bool)
          n103 = Equal?(x="", y=w89) -> (x = y?=w91:bool)
          n104 = Select(t="STOP", s=w70, f=w68) -> (s? t:f=w67:string)
          n105 = Select(t="STOP", s=w81, f=w79) -> (s? t:f=w78:string)
          n106 = Select(t="STOP", s=w86, f=w84) -> (s? t:f=w83:string)
          n107 = Select(t="STOP", s=w91, f=w89) -> (s? t:f=w88:string)
          n108 = Bundle(cluster=w66, "STATUS"=w67) -> (w65:T4)  [unwired: 2 in]
          n109 = Bundle(cluster=w73, "STATUS"=w78) -> (w72:T4)  [unwired: 2 in]
          n110 = Bundle(cluster=w75, "STATUS"=w83) -> (w74:T4)  [unwired: 2 in]
          n111 = Bundle(cluster=w77, "STATUS"=w88) -> (w76:T4)  [unwired: 2 in]
          n112 = local write "DISP LAB05-2"(w65) -> ()
          n113 = local write "DISP LAB05-1"(w72) -> ()
          n114 = local write "DISP LAB04-1"(w76) -> ()
          n115 = local write "DISP LAB04-2"(w74) -> ()
        }
        frame #5 {
          # "initialise analog input express vi's"
          n116 = for {
            N: 2.0 -> [_]
            n117 = call "sub vi - analog 1st setup v1.vi"() -> ()  [unwired: 11 in, 5 out]
          }
        }
        frame #6 {
          w136 = FALSE
          # "enable front panel, all settings done"
          n118 = property on="Tab Control 2" class="TabCtl (strict)"("DisabledEnum"=T11."Enabled" ("Disabled")) -> ()  [unwired: 2 in, 2 out]
          n119 = property on="Tab Control 2" class="TabCtl (strict)"() -> ("Pages"=w137:refnum<vi>[])  [unwired: 2 in, 2 out]
          n120 = Index Array(array=w137, index=6) -> (element=w139:refnum<vi>)
          n121 = local write "SHOW ADMIN PAGE"(w136) -> ()
          n122 = property class="Page"(reference=w139, "PageVis"=w136) -> ()  [unwired: 1 in, 2 out]
        }
      }
    }
    frame #2 {
      n123 = node-c288("loop  delay(mS)") -> (w143:T12)  [unwired: 3 in]
      n124 = timed-loop {
        timing: w143 -> [_]
        timing-out: [_] -> w142
        i -> [w165]
        stop <- "stop" stop-if-true
        n125 = node-c288() -> ()  [unwired: 1 in, 1 out]
        n126 = local read "SELECT LAB05-2"() -> (w145:T3)
        n127 = local read "SELECT LAB05-1"() -> (w146:T3)
        n128 = local read "SELECT LAB04-2"() -> (w147:T3)
        n129 = local read "SELECT LAB03-1"() -> (w150:T3)
        n130 = local read "SELECT LAB02-2"() -> (w151:T3)
        n131 = local read "SELECT LAB01-1"() -> (w154:T3)
        n132 = local read "SELECT LAB03-2"() -> (w149:T3)
        n133 = local read "SELECT LAB01-2"() -> (w153:T3)
        n134 = local read "SELECT LAB04-1"() -> (w148:T3)
        n135 = local read "SELECT LAB02-1"() -> (w152:T3)
        n136 = local read "run lab03-2"() -> (w159:bool)
        n137 = local read "run lab04-1"() -> (w158:bool)
        n138 = local read "run lab05-1"() -> (w156:bool)
        n139 = local read "run lab04-2"() -> (w157:bool)
        n140 = local read "run lab05-2"() -> (w155:bool)
        n141 = local read "run lab03-1"() -> (w160:bool)
        n142 = local read "run lab02-2"() -> (w161:bool)
        n143 = local read "run lab02-1"() -> (w162:bool)
        n144 = local read "run lab01-1"() -> (w164:bool)
        n145 = local read "run lab01-2"() -> (w163:bool)
        n146 = stacked-sequence {
          seq-local: [_ w227 _ _ _ _ _ _ _ _ _ _ _ _ _ _ _] -> [_ _ _ _ _ w1722 _ _ _ _ _ _ _ _ _ _ _]
          seq-local: [_ w226 _ _ _ _ _ _ _ _ _ _ _ _ _ _ _] -> [_ _ _ _ _ w1721 _ _ _ _ _ _ _ _ _ _ _]
          seq-local: [_ w213 _ _ _ _ _ _ _ _ _ _ _ _ _ _ _] -> [_ _ _ _ _ w1720 _ _ _ _ _ _ _ _ _ _ _]
          seq-local: [_ w212 _ _ _ _ _ _ _ _ _ _ _ _ _ _ _] -> [_ _ _ _ _ w1719 _ _ _ _ _ _ _ _ _ _ _]
          seq-local: [_ w211 _ _ _ _ _ _ _ _ _ _ _ _ _ _ _] -> [_ _ _ _ _ w1718 _ _ _ _ _ _ _ _ _ _ _]
          seq-local: [_ w210 _ _ _ _ _ _ _ _ _ _ _ _ _ _ _] -> [_ _ _ _ _ w1717 _ _ _ _ _ _ _ _ _ _ _]
          seq-local: [_ w209 _ _ _ _ _ _ _ _ _ _ _ _ _ _ _] -> [_ _ _ _ _ w1716 _ _ _ _ _ _ _ _ _ _ _]
          seq-local: [_ w208 _ _ _ _ _ _ _ _ _ _ _ _ _ _ _] -> [_ _ _ _ _ w1715 _ _ _ _ _ _ _ _ _ _ _]
          seq-local: [_ w207 _ _ _ _ _ _ _ _ _ _ _ _ _ _ _] -> [_ _ _ _ _ w1714 _ _ _ _ _ _ _ _ _ _ _]
          seq-local: [_ w206 _ _ _ _ _ _ _ _ _ _ _ _ _ _ _] -> [_ _ _ _ _ w1713 _ _ _ _ _ _ _ _ _ _ _]
          tunnel: w164 -> [_ _ w243 w408 w1322 w1742 w2052 w2267 _ _ _ _ w2712 w3200 _ _ w3475]
          tunnel: w163 -> [_ _ w242 w406 w1321 w1741 w2053 w2266 _ _ _ _ w2711 w3198 _ _ w3474]
          tunnel: w162 -> [_ _ w241 w404 w1320 w1740 w2051 w2265 _ _ _ _ w2710 w3196 _ _ w3473]
          tunnel: w161 -> [_ _ w240 w402 w1319 w1739 w2050 w2264 _ _ _ _ w2709 w3194 _ _ w3472]
          tunnel: w160 -> [_ _ w239 w400 w1318 w1738 w2049 w2263 _ _ _ _ w2708 w3192 _ _ w3471]
          tunnel: w159 -> [_ _ w238 w398 w1317 w1737 w2048 w2262 _ _ _ _ w2707 w3190 _ _ w3470]
          tunnel: w158 -> [_ _ w237 w396 w1316 w1736 w2047 w2261 _ _ _ _ w2706 w3188 _ _ w3469]
          tunnel: w157 -> [_ _ w236 w394 w1315 w1735 w2046 w2260 _ _ _ _ w2705 w3186 _ _ w3468]
          tunnel: w156 -> [_ _ w235 w392 w1314 w1734 w2045 w2259 _ _ _ _ w2704 w3184 _ _ w3467]
          tunnel: w155 -> [_ _ w234 w390 w1313 w1733 w2044 w2258 _ _ _ _ w2703 w3182 _ _ w3466]
          tunnel: w154 -> [_ _ _ w407 w1312 w1732 _ _ _ _ _ _ _ w3202 _ _ _]
          tunnel: w153 -> [_ _ _ w405 w1311 w1731 _ _ _ _ _ _ _ w3197 _ _ _]
          tunnel: w152 -> [_ _ _ w403 w1310 w1730 _ _ _ _ _ _ _ w3195 _ _ _]
          tunnel: w151 -> [_ _ _ w401 w1309 w1729 _ _ _ _ _ _ _ w3193 _ _ _]
          tunnel: w150 -> [_ _ _ w399 w1308 w1728 _ _ _ _ _ _ _ w3191 _ _ _]
          tunnel: w149 -> [_ _ _ w397 w1307 w1727 _ _ _ _ _ _ _ w3189 _ _ _]
          tunnel: w148 -> [_ _ _ w395 w1306 w1726 _ _ _ _ _ _ _ w3187 _ _ _]
          tunnel: w147 -> [_ _ _ w393 w1305 w1725 _ _ _ _ _ _ _ w3185 _ _ _]
          tunnel: w146 -> [_ _ _ w391 w1304 w1724 _ _ _ _ _ _ _ w3183 _ _ _]
          tunnel: w145 -> [_ _ _ w389 w1303 w1723 _ _ _ _ _ _ _ w3181 _ _ _]
          frame #0 {
            w169 = FALSE
            w174 = 0.5
            # "set up cycle control"
            n147 = local read "jig cycle"() -> (w173:dbl)
            n148 = Divide(x="JIG ON TIME (S)", y=w174) -> (x/y=→"on loops":dbl)
            n149 = Divide(x="JIG OFF TIME (S)", y=w174) -> (x/y=→"off loops":dbl)
            n150 = Increment(x=w173) -> (x+1=w172:dbl)
            n151 = local write "TEMP update"(w169) -> ()
            n152 = local write "AI update"(w169) -> ()
            n153 = local write "jig cycle"(w172) -> ()
            n154 = event shown="[1] \"SHOW ADMIN PAGE\": Value Change" {
              selector: _ -> [_ _]
              dyn-events: _ -> [_ _]
              timeout: 10 -> [_ _]
              event Timeout {
                n155 = event-data() -> ()  [unwired: 1 in, 3 out]
              }
              event "SHOW ADMIN PAGE": Value Change {
                n156 = event-data() -> ()  [unwired: 1 in, 6 out]
                n157 = stacked-sequence {
                  seq-local: [_ w178 _] -> [_ _ w179]
                  frame #0 {
                    n158 = global write "Global 1.vi" "password"("9999") -> ()
                  }
                  frame #1 {
                    n159 = call "sub vi - password 1.vi"() -> ("RESULT"=w178:bool)  [unwired: 11 in]
                  }
                  frame #2 {
                    w181 = FALSE
                    n160 = property on="Tab Control 2" class="TabCtl (strict)"() -> ("Pages"=w185:refnum<vi>[])  [unwired: 2 in, 2 out]
                    n161 = Select(t=TRUE, s=w179, f=w181) -> (s? t:f=w180:bool)
                    n162 = Index Array(array=w185, index=6) -> (element=w183:refnum<vi>)
                    n163 = local write "SHOW ADMIN PAGE"(w181) -> ()
                    n164 = property class="Page"(reference=w183, "PageVis"=w180) -> ()  [unwired: 1 in, 2 out]
                  }
                }
              }
            }
          }
          frame #1 {
            w223 = 60.0
            # "convert temperature rise minutes to cycles"
            n165 = local read "SET LAB05-2"() -> (w187:T5)
            n166 = local read "SET LAB05-1"() -> (w189:T5)
            n167 = local read "SET LAB04-2"() -> (w191:T5)
            n168 = local read "SET LAB01-1"() -> (w205:T5)
            n169 = local read "SET LAB01-2"() -> (w203:T5)
            n170 = local read "SET LAB02-2"() -> (w199:T5)
            n171 = local read "SET LAB04-1"() -> (w193:T5)
            n172 = local read "SET LAB03-1"() -> (w197:T5)
            n173 = local read "SET LAB03-2"() -> (w195:T5)
            n174 = local read "SET LAB02-1"() -> (w201:T5)
            n175 = local read "JIG OFF TIME (S)"() -> (w228:dbl)
            n176 = local read "JIG ON TIME (S)"() -> (w229:dbl)
            n177 = Unbundle(w187) -> ("T-RISE mins"=w186:dbl)  [unwired: 4 out]
            n178 = Unbundle(w189) -> ("T-RISE mins"=w188:dbl)  [unwired: 4 out]
            n179 = Unbundle(w205) -> ("T-RISE mins"=w204:dbl)  [unwired: 4 out]
            n180 = Unbundle(w191) -> ("T-RISE mins"=w190:dbl)  [unwired: 4 out]
            n181 = Unbundle(w203) -> ("T-RISE mins"=w202:dbl)  [unwired: 4 out]
            n182 = Unbundle(w201) -> ("T-RISE mins"=w200:dbl)  [unwired: 4 out]
            n183 = Unbundle(w193) -> ("T-RISE mins"=w192:dbl)  [unwired: 4 out]
            n184 = Unbundle(w199) -> ("T-RISE mins"=w198:dbl)  [unwired: 4 out]
            n185 = Unbundle(w195) -> ("T-RISE mins"=w194:dbl)  [unwired: 4 out]
            n186 = Unbundle(w197) -> ("T-RISE mins"=w196:dbl)  [unwired: 4 out]
            n187 = Add(x=w229, y=w228) -> (x+y=w222:dbl)
            n188 = Multiply(x=w223, y=w194) -> (x*y=w218:dbl)
            n189 = Multiply(x=w223, y=w192) -> (x*y=w217:dbl)
            n190 = Multiply(x=w223, y=w190) -> (x*y=w216:dbl)
            n191 = Multiply(x=w223, y=w188) -> (x*y=w215:dbl)
            n192 = Multiply(x=w223, y=w186) -> (x*y=w214:dbl)
            n193 = Multiply(x=w223, y=w202) -> (x*y=w224:dbl)
            n194 = Multiply(x=w223, y=w196) -> (x*y=w219:dbl)
            n195 = Multiply(x=w223, y=w204) -> (x*y=w225:dbl)
            n196 = Multiply(x=w223, y=w200) -> (x*y=w221:dbl)
            n197 = Multiply(x=w223, y=w198) -> (x*y=w220:dbl)
            n198 = Divide(x=w215, y=w222) -> (x/y=w207:dbl)
            n199 = Divide(x=w216, y=w222) -> (x/y=w208:dbl)
            n200 = Divide(x=w217, y=w222) -> (x/y=w209:dbl)
            n201 = Divide(x=w214, y=w222) -> (x/y=w206:dbl)
            n202 = Divide(x=w219, y=w222) -> (x/y=w211:dbl)
            n203 = Divide(x=w225, y=w222) -> (x/y=w227:dbl)
            n204 = Divide(x=w224, y=w222) -> (x/y=w226:dbl)
            n205 = Divide(x=w221, y=w222) -> (x/y=w213:dbl)
            n206 = Divide(x=w220, y=w222) -> (x/y=w212:dbl)
            n207 = Divide(x=w218, y=w222) -> (x/y=w210:dbl)
          }
          frame #2 {
            # "control cycle loops"
            n208 = local read "JIG OFF TIME (S)"() -> (w232:dbl)
            n209 = local read "JIG ON TIME (S)"() -> (w231:dbl)
            n210 = local read "jig cycle"() -> (w245:dbl)
            n211 = local read "on loops"() -> (w247:dbl)
            n212 = local read "off loops"() -> (w246:dbl)
            n213 = Add(x=w232, y=w231) -> (x+y=w230:dbl)
            n214 = Add(x=w247, y=w246) -> (x+y=w233:dbl)
            n215 = Greater Or Equal?(x=w245, y=w233) -> (x >= y?=w244:bool)
            n216 = case shown="True" w244 {
              tunnel: w243 -> [_ w258]
              tunnel: w242 -> [_ w257]
              tunnel: w241 -> [_ w256]
              tunnel: w240 -> [_ w255]
              tunnel: w239 -> [_ w254]
              tunnel: w238 -> [_ w253]
              tunnel: w237 -> [_ w252]
              tunnel: w236 -> [_ w251]
              tunnel: w235 -> [_ w250]
              tunnel: w234 -> [_ w249]
              tunnel: w230 -> [_ w248]
              frame False {
              }
              frame True {
                # "increment cycle value and convert cycles to minutes for temp rise"
                n217 = stacked-sequence {
                  tunnel: w258 -> [w268 _ _ _ _ _ _ _ _ _]
                  tunnel: w257 -> [_ w280 _ _ _ _ _ _ _ _]
                  tunnel: w256 -> [_ _ w292 _ _ _ _ _ _ _]
                  tunnel: w255 -> [_ _ _ w304 _ _ _ _ _ _]
                  tunnel: w254 -> [_ _ _ _ w316 _ _ _ _ _]
                  tunnel: w253 -> [_ _ _ _ _ w328 _ _ _ _]
                  tunnel: w252 -> [_ _ _ _ _ _ w340 _ _ _]
                  tunnel: w251 -> [_ _ _ _ _ _ _ w352 _ _]
                  tunnel: w250 -> [_ _ _ _ _ _ _ _ w364 _]
                  tunnel: w249 -> [_ _ _ _ _ _ _ _ _ w376]
                  tunnel: w248 -> [w265 w277 w289 w301 w313 w325 w337 w349 w361 w373]
                  frame #0 {
                    # "LAB01-1"
                    n218 = local read "DISP LAB01-1"() -> (w263:T4)
                    n219 = Unbundle(w263) -> ("CYCLE"=w264:dbl)  [unwired: 2 out]
                    n220 = case shown="True" w268 {
                      tunnel: w264 -> [w269 w271]
                      tunnel: [w269 w270] -> w262
                      frame False {
                      }
                      frame True {
                        n221 = Increment(x=w271) -> (x+1=w270:dbl)
                      }
                    }
                    n222 = Multiply(x=w262, y=w265) -> (x*y=w266:dbl)
                    n223 = Divide(x=w266, y=60.0) -> (x/y=w261:dbl)
                    n224 = Bundle(cluster=w263, "CYCLE"=w262, "MINS"=w261) -> (w260:T4)  [unwired: 1 in]
                    n225 = local write "DISP LAB01-1"(w260) -> ()
                  }
                  frame #1 {
                    # "update cycle value"
                    # "LAB01-2"
                    n226 = local read "DISP LAB01-2"() -> (w275:T4)
                    n227 = Unbundle(w275) -> ("CYCLE"=w276:dbl)  [unwired: 2 out]
                    n228 = case shown="True" w280 {
                      tunnel: w276 -> [w281 w283]
                      tunnel: [w281 w282] -> w273
                      frame False {
                      }
                      frame True {
                        n229 = Increment(x=w283) -> (x+1=w282:dbl)
                      }
                    }
                    n230 = Multiply(x=w273, y=w277) -> (x*y=w278:dbl)
                    n231 = Divide(x=w278, y=60.0) -> (x/y=w272:dbl)
                    n232 = Bundle(cluster=w275, "CYCLE"=w273, "MINS"=w272) -> (w274:T4)  [unwired: 1 in]
                    n233 = local write "DISP LAB01-2"(w274) -> ()
                  }
                  frame #2 {
                    # "update cycle value"
                    # "LAB02-1"
                    n234 = local read "DISP LAB02-1"() -> (w287:T4)
                    n235 = Unbundle(w287) -> ("CYCLE"=w288:dbl)  [unwired: 2 out]
                    n236 = case shown="True" w292 {
                      tunnel: [w293 w295] -> w285
                      tunnel: w288 -> [w293 w294]
                      frame False {
                      }
                      frame True {
                        n237 = Increment(x=w294) -> (x+1=w295:dbl)
                      }
                    }
                    n238 = Multiply(x=w285, y=w289) -> (x*y=w290:dbl)
                    n239 = Divide(x=w290, y=60.0) -> (x/y=w284:dbl)
                    n240 = Bundle(cluster=w287, "CYCLE"=w285, "MINS"=w284) -> (w286:T4)  [unwired: 1 in]
                    n241 = local write "DISP LAB02-1"(w286) -> ()
                  }
                  frame #3 {
                    # "update cycle value"
                    # "LAB02-2"
                    n242 = local read "DISP LAB02-2"() -> (w299:T4)
                    n243 = Unbundle(w299) -> ("CYCLE"=w300:dbl)  [unwired: 2 out]
                    n244 = case shown="True" w304 {
                      tunnel: [w305 w307] -> w298
                      tunnel: w300 -> [w305 w306]
                      frame False {
                      }
                      frame True {
                        n245 = Increment(x=w306) -> (x+1=w307:dbl)
                      }
                    }
                    n246 = Multiply(x=w298, y=w301) -> (x*y=w302:dbl)
                    n247 = Divide(x=w302, y=60.0) -> (x/y=w297:dbl)
                    n248 = Bundle(cluster=w299, "CYCLE"=w298, "MINS"=w297) -> (w296:T4)  [unwired: 1 in]
                    n249 = local write "DISP LAB02-2"(w296) -> ()
                  }
                  frame #4 {
                    # "update cycle value"
                    # "LAB03-1"
                    n250 = local read "DISP LAB03-1"() -> (w311:T4)
                    n251 = Unbundle(w311) -> ("CYCLE"=w312:dbl)  [unwired: 2 out]
                    n252 = case shown="True" w316 {
                      tunnel: [w317 w319] -> w308
                      tunnel: w312 -> [w317 w318]
                      frame False {
                      }
                      frame True {
                        n253 = Increment(x=w318) -> (x+1=w319:dbl)
                      }
                    }
                    n254 = Multiply(x=w308, y=w313) -> (x*y=w314:dbl)
                    n255 = Divide(x=w314, y=60.0) -> (x/y=w309:dbl)
                    n256 = Bundle(cluster=w311, "CYCLE"=w308, "MINS"=w309) -> (w310:T4)  [unwired: 1 in]
                    n257 = local write "DISP LAB03-1"(w310) -> ()
                  }
                  frame #5 {
                    # "update cycle value"
                    # "LAB03-2"
                    n258 = local read "DISP LAB03-2"() -> (w323:T4)
                    n259 = Unbundle(w323) -> ("CYCLE"=w324:dbl)  [unwired: 2 out]
                    n260 = case shown="False" w328 {
                      tunnel: [w329 w331] -> w322
                      tunnel: w324 -> [w329 w330]
                      frame False {
                      }
                      frame True {
                        n261 = Increment(x=w330) -> (x+1=w331:dbl)
                      }
                    }
                    n262 = Multiply(x=w322, y=w325) -> (x*y=w326:dbl)
                    n263 = Divide(x=w326, y=60.0) -> (x/y=w321:dbl)
                    n264 = Bundle(cluster=w323, "CYCLE"=w322, "MINS"=w321) -> (w320:T4)  [unwired: 1 in]
                    n265 = local write "DISP LAB03-2"(w320) -> ()
                  }
                  frame #6 {
                    # "update cycle value"
                    # "LAB04-1"
                    n266 = local read "DISP LAB04-1"() -> (w335:T4)
                    n267 = Unbundle(w335) -> ("CYCLE"=w336:dbl)  [unwired: 2 out]
                    n268 = case shown="True" w340 {
                      tunnel: [w341 w343] -> w333
                      tunnel: w336 -> [w341 w342]
                      frame False {
                      }
                      frame True {
                        n269 = Increment(x=w342) -> (x+1=w343:dbl)
                      }
                    }
                    n270 = Multiply(x=w333, y=w337) -> (x*y=w338:dbl)
                    n271 = Divide(x=w338, y=60.0) -> (x/y=w332:dbl)
                    n272 = Bundle(cluster=w335, "CYCLE"=w333, "MINS"=w332) -> (w334:T4)  [unwired: 1 in]
                    n273 = local write "DISP LAB04-1"(w334) -> ()
                  }
                  frame #7 {
                    # "update cycle value"
                    # "LAB04-2"
                    n274 = local read "DISP LAB04-2"() -> (w347:T4)
                    n275 = Unbundle(w347) -> ("CYCLE"=w348:dbl)  [unwired: 2 out]
                    n276 = case shown="True" w352 {
                      tunnel: [w353 w355] -> w345
                      tunnel: w348 -> [w353 w354]
                      frame False {
                      }
                      frame True {
                        n277 = Increment(x=w354) -> (x+1=w355:dbl)
                      }
                    }
                    n278 = Multiply(x=w345, y=w349) -> (x*y=w351:dbl)
                    n279 = Divide(x=w351, y=60.0) -> (x/y=w344:dbl)
                    n280 = Bundle(cluster=w347, "CYCLE"=w345, "MINS"=w344) -> (w346:T4)  [unwired: 1 in]
                    n281 = local write "DISP LAB04-2"(w346) -> ()
                  }
                  frame #8 {
                    # "update cycle value"
                    # "LAB05-1"
                    n282 = local read "DISP LAB05-1"() -> (w359:T4)
                    n283 = Unbundle(w359) -> ("CYCLE"=w360:dbl)  [unwired: 2 out]
                    n284 = case shown="True" w364 {
                      tunnel: [w365 w367] -> w357
                      tunnel: w360 -> [w365 w366]
                      frame False {
                      }
                      frame True {
                        n285 = Increment(x=w366) -> (x+1=w367:dbl)
                      }
                    }
                    n286 = Multiply(x=w357, y=w361) -> (x*y=w362:dbl)
                    n287 = Divide(x=w362, y=60.0) -> (x/y=w356:dbl)
                    n288 = Bundle(cluster=w359, "CYCLE"=w357, "MINS"=w356) -> (w358:T4)  [unwired: 1 in]
                    n289 = local write "DISP LAB05-1"(w358) -> ()
                  }
                  frame #9 {
                    # "update cycle value"
                    # "LAB05-2"
                    n290 = local read "DISP LAB05-2"() -> (w372:T4)
                    n291 = Unbundle(w372) -> ("CYCLE"=w371:dbl)  [unwired: 2 out]
                    n292 = case shown="True" w376 {
                      tunnel: [w377 w379] -> w370
                      tunnel: w371 -> [w377 w378]
                      frame False {
                      }
                      frame True {
                        n293 = Increment(x=w378) -> (x+1=w379:dbl)
                      }
                    }
                    n294 = Multiply(x=w370, y=w373) -> (x*y=w374:dbl)
                    n295 = Divide(x=w374, y=60.0) -> (x/y=w369:dbl)
                    n296 = Bundle(cluster=w372, "CYCLE"=w370, "MINS"=w369) -> (w368:T4)  [unwired: 1 in]
                    n297 = local write "DISP LAB05-2"(w368) -> ()
                  }
                }
                n298 = local write "jig cycle"(0) -> ()
              }
            }
          }
          frame #3 {
            (unwired) "c:\\BAT\\labdatav2\\"
            # "START & STOP test RUN switch change, start test if true and stop test if false"
            n299 = Get Date/Time In Seconds() -> (seconds since 1Jan1904=w387:timestamp)
            n300 = local read "C drive data root dir"() -> (w380:path)
            n301 = Format Date/Time String(time format string (%c)="%b%d", seconds (now)=w387) -> (date/time string=w411:string)  [unwired: 1 in]
            n302 = Format Date/Time String(time format string (%c)="%H%M", seconds (now)=w387) -> (date/time string=w409:string)  [unwired: 1 in]
            n303 = Format Date/Time String(time format string (%c)="%Y", seconds (now)=w387) -> (date/time string=w386:string)  [unwired: 1 in]
            n304 = Path To String(path=w380) -> (string=w383:string)
            n305 = global write "Global 1.vi" "C drive root path"(w380) -> ()
            n306 = Concatenate Strings(w383, "\\") -> (w381:string)
            n307 = event shown="[1] \"RUN LAB01-1\": Value Change" {
              selector: _ -> [_ _ _ _ _ _ _ _ _ _ _]
              dyn-events: _ -> [_ _ _ _ _ _ _ _ _ _ _]
              timeout: 10 -> [_ _ _ _ _ _ _ _ _ _ _]
              tunnel: w381 -> [_ w419 w508 w597 w686 w775 w864 w953 w1042 w1131 w1220]
              tunnel: w411 -> [_ w418 w507 w596 w685 w774 w863 w952 w1041 w1130 w1219]
              tunnel: w409 -> [_ w416 w506 w595 w684 w773 w862 w951 w1040 w1129 w1218]
              tunnel: w407 -> [_ w417 _ _ _ _ _ _ _ _ _]
              tunnel: w408 -> [_ _ _ _ _ _ _ _ _ _ _]
              tunnel: w406 -> [_ _ _ _ _ _ _ _ _ _ _]
              tunnel: w405 -> [_ _ w505 _ _ _ _ _ _ _ _]
              tunnel: w404 -> [_ _ _ _ _ _ _ _ _ _ _]
              tunnel: w403 -> [_ _ _ w594 _ _ _ _ _ _ _]
              tunnel: w402 -> [_ _ _ _ _ _ _ _ _ _ _]
              tunnel: w401 -> [_ _ _ _ w683 _ _ _ _ _ _]
              tunnel: w400 -> [_ _ _ _ _ _ _ _ _ _ _]
              tunnel: w399 -> [_ _ _ _ _ w772 _ _ _ _ _]
              tunnel: w398 -> [_ _ _ _ _ _ _ _ _ _ _]
              tunnel: w397 -> [_ _ _ _ _ _ w861 _ _ _ _]
              tunnel: w396 -> [_ _ _ _ _ _ _ _ _ _ _]
              tunnel: w395 -> [_ _ _ _ _ _ _ w950 _ _ _]
              tunnel: w394 -> [_ _ _ _ _ _ _ _ _ _ _]
              tunnel: w393 -> [_ _ _ _ _ _ _ _ w1039 _ _]
              tunnel: w392 -> [_ _ _ _ _ _ _ _ _ _ _]
              tunnel: w391 -> [_ _ _ _ _ _ _ _ _ w1128 _]
              tunnel: w390 -> [_ _ _ _ _ _ _ _ _ _ _]
              tunnel: w389 -> [_ _ _ _ _ _ _ _ _ _ w1217]
              tunnel: w386 -> [_ w415 w504 w593 w682 w771 w860 w949 w1038 w1127 w1216]
              tunnel: [_ w414 w503 w592 w681 w770 w859 w948 w1037 w1126 w1215] -> w384
              event Timeout {
                n308 = event-data() -> ()  [unwired: 1 in, 3 out]
              }
              event "RUN LAB01-1": Value Change {
                n309 = event-data() -> ("NewVal"=w413:bool)  [unwired: 1 in, 5 out]
                n310 = local write "run lab01-1"(w413) -> ()
                n311 = case shown="True" w413 {
                  tunnel: w419 -> [_ w449]
                  tunnel: w418 -> [_ w448]
                  tunnel: w417 -> [w421 w447]
                  tunnel: w416 -> [_ w446]
                  tunnel: w415 -> [_ w445]
                  tunnel: [w420 w444] -> w414
                  frame False {
                    # "stop test"
                    n312 = stacked-sequence {
                      tunnel: w421 -> [_ w433 _ _]
                      tunnel: [_ w425 _ _] -> w420
                      frame #0 {
                        n313 = local read "DISP LAB01-1"() -> (w424:T4)
                        n314 = Bundle(cluster=w424, "STATUS"="STOP") -> (w422:T4)  [unwired: 2 in]
                        n315 = local write "DISP LAB01-1"(w422) -> ()
                      }
                      frame #1 {
                        n316 = local read "DISP LAB01-1"() -> (w432:T4)
                        n317 = Unbundle(w432) -> ("CYCLE"=w430:dbl, "MINS"=w431:dbl)  [unwired: 1 out]
                        n318 = case shown="\"CYCLE TEST\"" w433 {
                          tunnel: w431 -> [_ _ w440]
                          tunnel: w430 -> [w438 w439 _]
                          tunnel: [w438 w439 w440] -> w429
                          frame "CHART TEST", Default {
                          }
                          frame "CYCLE TEST" {
                          }
                          frame "T-RISE TEST" {
                          }
                        }
                        n319 = local read "TDMS LAB01-1"() -> (w437:refnum<k34>)
                        n320 = Build Array("STOPPED") -> (w434:string[])
                        n321 = Build Array(w429) -> (w428:dbl[])
                        n322 = TDMS Write(0:w437, 5:"TEST RESULT", 7:w434, 9:w428) -> (4:w426:refnum<k34>, 15:w427:errorcluster)  [unwired: 2 in, 2 out]
                        n323 = TDMS Close(8:w427, 11:w426) -> (0:w425:errorcluster)  [unwired: 1 out]
                      }
                      frame #2 {
                        n324 = call "Save data file to network drive v1.vi"("panel id"="LAB01-1") -> ("network file save error"=w441:errorcluster)  [unwired: 9 in, 1 out]
                        n325 = local write "RESULT LAB01-1"(FALSE) -> ()
                        n326 = local write "data file error"(w441) -> ()
                      }
                      frame #3 {
                      }
                    }
                  }
                  frame True {
                    # "start new test and create test file"
                    n327 = stacked-sequence {
                      seq-local: [w450 _ _ _ _] -> [_ w471 _ _ _]
                      tunnel: w449 -> [w455 _ _ _ _]
                      tunnel: w448 -> [w451 _ _ _ _]
                      tunnel: w447 -> [w465 _ _ _ _]
                      tunnel: w446 -> [w458 _ _ _ _]
                      tunnel: w445 -> [w453 _ _ _ _]
                      tunnel: [_ w472 _ _ _] -> w444
                      frame #0 {
                        w452 = "\\"
                        n328 = local read "SET LAB01-1"() -> (w460:T5)
                        n329 = case shown="\"CHART TEST\", Default" w465 {
                          tunnel: ["CHART TEST-" "CYCLE TEST-" "T-RISE TEST-"] -> w461
                          frame "CHART TEST", Default {
                          }
                          frame "CYCLE TEST" {
                          }
                          frame "T-RISE TEST" {
                          }
                        }
                        n330 = Unbundle(w460) -> ("DESCRIPTION"=w459:string)  [unwired: 4 out]
                        n331 = Concatenate Strings(w455, "LAB01-1\\", w453, w452, w451, w452) -> (w462:string)
                        n332 = String To Path(string=w462) -> (path=w464:path)
                        n333 = Concatenate Strings(w462, w461, w459, "-", w458, ".tdms") -> (w450:string)
                        n334 = Create Folder(path (use dialog)=w464) -> (error out=w463:errorcluster)  [unwired: 2 in, 2 out]
                        n335 = call <vilib>:"Clear Errors.vi"("error in (no error)"=w463) -> ()  [unwired: 6 in, 1 out]
                        n336 = global write "Global 1.vi" "LAB01-1 FILE"(w450) -> ()
                      }
                      frame #1 {
                        n337 = String To Path(string=w471) -> (path=w469:path)
                        n338 = TDMS Open(5:FALSE, 6:FALSE, 10:T15."create or replace" ("operation (0:open)"), 11:w469) -> (0:w472:errorcluster, 3:→"TDMS LAB01-1":refnum<k34>)  [unwired: 3 in]
                      }
                      frame #2 {
                        n339 = local read "SET LAB01-1"() -> (w481:T5)
                        n340 = local read "TDMS LAB01-1"() -> (w492:refnum<k34>)
                        n341 = Build Array("Testers Name", "Description", "Set Test Cycles", "T-Rise minutes", "T-Rise Deg C") -> (w482:string[])
                        n342 = Unbundle(w481) -> ("NAME"=w480:string, "DESCRIPTION"=w479:string, "CYCLES"=w478:dbl, "T-RISE mins"=w477:dbl, "T-RISE deg C"=w476:dbl)
                        n343 = Number To Decimal String(number=w478) -> (decimal integer string=w491:string)  [unwired: 1 in]
                        n344 = Number To Decimal String(number=w477) -> (decimal integer string=w490:string)  [unwired: 1 in]
                        n345 = Number To Decimal String(number=w476) -> (decimal integer string=w489:string)  [unwired: 1 in]
                        n346 = Build Array(w480, w479, w491, w490, w489) -> (w488:string[])
                        n347 = TDMS Set Properties(5:w488, 7:w482, 11:w492) -> ()  [unwired: 3 in, 4 out]
                      }
                      frame #3 {
                        w493 = 0.0
                        n348 = local read "DISP LAB01-1"() -> (w496:T4)
                        n349 = Bundle(cluster=w496, "CYCLE"=w493, "MINS"=w493, "STATUS"="RUN") -> (w495:T4)
                        n350 = local write "DISP LAB01-1"(w495) -> ()
                      }
                      frame #4 {
                        n351 = local read "SIG LAB01-1"() -> (w499:T2)
                        n352 = local read "TEMP START LAB01-1"() -> (w501:cluster{"TL":dbl, "TN":dbl})
                        n353 = Unbundle(w499) -> ("Tmp Live"=w498:dbl, "Tmp Neut"=w497:dbl)  [unwired: 3 out]
                        n354 = Bundle(cluster=w501, "TL"=w498, "TN"=w497) -> (w500:cluster{"TL":dbl, "TN":dbl})
                        n355 = local write "TEMP START LAB01-1"(w500) -> ()
                      }
                    }
                  }
                }
              }
              event "RUN LAB01-2": Value Change {
                n356 = event-data() -> ("NewVal"=w502:bool)  [unwired: 1 in, 5 out]
                n357 = local write "run lab01-2"(w502) -> ()
                n358 = case shown="False" w502 {
                  tunnel: w508 -> [_ w538]
                  tunnel: w507 -> [_ w537]
                  tunnel: w505 -> [w510 w536]
                  tunnel: w506 -> [_ w535]
                  tunnel: w504 -> [_ w534]
                  tunnel: [w509 w533] -> w503
                  frame False {
                    # "stop test"
                    n359 = stacked-sequence {
                      tunnel: w510 -> [w519 _]
                      tunnel: [w511 _] -> w509
                      frame #0 {
                        n360 = local read "DISP LAB01-2"() -> (w518:T4)
                        n361 = Unbundle(w518) -> ("CYCLE"=w516:dbl, "MINS"=w517:dbl)  [unwired: 1 out]
                        n362 = case shown="\"CHART TEST\", Default" w519 {
                          tunnel: w517 -> [_ _ w526]
                          tunnel: w516 -> [w524 w525 _]
                          tunnel: [w524 w525 w526] -> w515
                          frame "CHART TEST", Default {
                          }
                          frame "CYCLE TEST" {
                          }
                          frame "T-RISE TEST" {
                          }
                        }
                        n363 = local read "TDMS LAB01-2"() -> (w523:refnum<k34>)
                        n364 = Build Array("STOPPED") -> (w520:string[])
                        n365 = Build Array(w515) -> (w514:dbl[])
                        n366 = TDMS Write(0:w523, 5:"TEST RESULT", 7:w520, 9:w514) -> (4:w512:refnum<k34>, 15:w513:errorcluster)  [unwired: 2 in, 2 out]
                        n367 = TDMS Close(8:w513, 11:w512) -> (0:w511:errorcluster)  [unwired: 1 out]
                      }
                      frame #1 {
                        n368 = local read "DISP LAB01-2"() -> (w532:T4)
                        n369 = Bundle(cluster=w532, "STATUS"="STOP") -> (w530:T4)  [unwired: 2 in]
                        n370 = call "Save data file to network drive v1.vi"("panel id"="LAB01-2") -> ("network file save error"=w527:errorcluster)  [unwired: 9 in, 1 out]
                        n371 = local write "RESULT LAB01-2"(FALSE) -> ()
                        n372 = local write "DISP LAB01-2"(w530) -> ()
                        n373 = local write "data file error"(w527) -> ()
                      }
                    }
                  }
                  frame True {
                    # "start new test and create test file"
                    n374 = stacked-sequence {
                      seq-local: [w539 _ _ _ _] -> [_ w564 _ _ _]
                      tunnel: w538 -> [w544 _ _ _ _]
                      tunnel: w537 -> [w541 _ _ _ _]
                      tunnel: w536 -> [w554 _ _ _ _]
                      tunnel: w535 -> [w547 _ _ _ _]
                      tunnel: w534 -> [w542 _ _ _ _]
                      tunnel: [_ w558 _ _ _] -> w533
                      frame #0 {
                        w540 = "\\"
                        n375 = local read "SET LAB01-2"() -> (w549:T5)
                        n376 = case shown="\"CHART TEST\", Default" w554 {
                          tunnel: ["CHART TEST-" "CYCLE TEST-" "T-RISE TEST-"] -> w550
                          frame "CHART TEST", Default {
                          }
                          frame "CYCLE TEST" {
                          }
                          frame "T-RISE TEST" {
                          }
                        }
                        n377 = Unbundle(w549) -> ("DESCRIPTION"=w548:string)  [unwired: 4 out]
                        n378 = Concatenate Strings(w544, "LAB01-2\\", w542, w540, w541, w540) -> (w551:string)
                        n379 = String To Path(string=w551) -> (path=w553:path)
                        n380 = Concatenate Strings(w551, w550, w548, "-", w547, ".tdms") -> (w539:string)
                        n381 = Create Folder(path (use dialog)=w553) -> (error out=w552:errorcluster)  [unwired: 2 in, 2 out]
                        n382 = global write "Global 1.vi" "LAB01-2 FILE"(w539) -> ()
                        n383 = call <vilib>:"Clear Errors.vi"("error in (no error)"=w552) -> ()  [unwired: 6 in, 1 out]
                      }
                      frame #1 {
                        n384 = String To Path(string=w564) -> (path=w559:path)
                        n385 = TDMS Open(5:FALSE, 6:FALSE, 10:T15."create or replace" ("operation (0:open)"), 11:w559) -> (0:w558:errorcluster, 3:→"TDMS LAB01-2":refnum<k34>)  [unwired: 3 in]
                      }
                      frame #2 {
                        n386 = local read "SET LAB01-2"() -> (w570:T5)
                        n387 = local read "TDMS LAB01-2"() -> (w581:refnum<k34>)
                        n388 = Build Array("Testers Name", "Description", "Set Test Cycles", "T-Rise minutes", "T-Rise Deg C") -> (w571:string[])
                        n389 = Unbundle(w570) -> ("NAME"=w569:string, "DESCRIPTION"=w568:string, "CYCLES"=w567:dbl, "T-RISE mins"=w566:dbl, "T-RISE deg C"=w565:dbl)
                        n390 = Number To Decimal String(number=w567) -> (decimal integer string=w580:string)  [unwired: 1 in]
                        n391 = Number To Decimal String(number=w566) -> (decimal integer string=w579:string)  [unwired: 1 in]
                        n392 = Number To Decimal String(number=w565) -> (decimal integer string=w578:string)  [unwired: 1 in]
                        n393 = Build Array(w569, w568, w580, w579, w578) -> (w577:string[])
                        n394 = TDMS Set Properties(5:w577, 7:w571, 11:w581) -> ()  [unwired: 3 in, 4 out]
                      }
                      frame #3 {
                        w583 = 0.0
                        n395 = local read "DISP LAB01-2"() -> (w585:T4)
                        n396 = Bundle(cluster=w585, "CYCLE"=w583, "MINS"=w583, "STATUS"="RUN") -> (w584:T4)
                        n397 = local write "DISP LAB01-2"(w584) -> ()
                      }
                      frame #4 {
                        n398 = local read "SIG LAB01-2"() -> (w588:T2)
                        n399 = local read "TEMP START LAB01-2"() -> (w590:cluster{"TL":dbl, "TN":dbl})
                        n400 = Unbundle(w588) -> ("Tmp Live"=w587:dbl, "Tmp Neut"=w586:dbl)  [unwired: 3 out]
                        n401 = Bundle(cluster=w590, "TL"=w587, "TN"=w586) -> (w589:cluster{"TL":dbl, "TN":dbl})
                        n402 = local write "TEMP START LAB01-2"(w589) -> ()
                      }
                    }
                  }
                }
              }
              event "RUN LAB02-1": Value Change {
                n403 = event-data() -> ("NewVal"=w591:bool)  [unwired: 1 in, 5 out]
                n404 = local write "run lab02-1"(w591) -> ()
                n405 = case shown="False" w591 {
                  tunnel: w597 -> [_ w627]
                  tunnel: w596 -> [_ w626]
                  tunnel: w594 -> [w599 w625]
                  tunnel: w595 -> [_ w624]
                  tunnel: w593 -> [_ w623]
                  tunnel: [w598 w622] -> w592
                  frame False {
                    # "stop test"
                    n406 = stacked-sequence {
                      tunnel: w599 -> [w608 _]
                      tunnel: [w600 _] -> w598
                      frame #0 {
                        n407 = local read "DISP LAB02-1"() -> (w607:T4)
                        n408 = Unbundle(w607) -> ("CYCLE"=w605:dbl, "MINS"=w606:dbl)  [unwired: 1 out]
                        n409 = case shown="\"CYCLE TEST\"" w608 {
                          tunnel: w606 -> [_ _ w615]
                          tunnel: w605 -> [w613 w614 _]
                          tunnel: [w613 w614 w615] -> w604
                          frame "CHART TEST", Default {
                          }
                          frame "CYCLE TEST" {
                          }
                          frame "T-RISE TEST" {
                          }
                        }
                        n410 = local read "TDMS LAB02-1"() -> (w612:refnum<k34>)
                        n411 = Build Array("STOPPED") -> (w609:string[])
                        n412 = Build Array(w604) -> (w603:dbl[])
                        n413 = TDMS Write(0:w612, 5:"TEST RESULT", 7:w609, 9:w603) -> (4:w601:refnum<k34>, 15:w602:errorcluster)  [unwired: 2 in, 2 out]
                        n414 = TDMS Close(8:w602, 11:w601) -> (0:w600:errorcluster)  [unwired: 1 out]
                      }
                      frame #1 {
                        n415 = local read "DISP LAB02-1"() -> (w621:T4)
                        n416 = Bundle(cluster=w621, "STATUS"="STOP") -> (w619:T4)  [unwired: 2 in]
                        n417 = local write "RESULT LAB02-1"(FALSE) -> ()
                        n418 = local write "DISP LAB02-1"(w619) -> ()
                        n419 = call "Save data file to network drive v1.vi"("panel id"="LAB02-1") -> ("network file save error"=w616:errorcluster)  [unwired: 9 in, 1 out]
                        n420 = local write "data file error"(w616) -> ()
                      }
                    }
                  }
                  frame True {
                    # "start new test and create test file"
                    n421 = stacked-sequence {
                      seq-local: [w628 _ _ _ _] -> [_ w653 _ _ _]
                      tunnel: w627 -> [w633 _ _ _ _]
                      tunnel: w626 -> [w630 _ _ _ _]
                      tunnel: w625 -> [w643 _ _ _ _]
                      tunnel: w624 -> [w636 _ _ _ _]
                      tunnel: w623 -> [w631 _ _ _ _]
                      tunnel: [_ w647 _ _ _] -> w622
                      frame #0 {
                        w629 = "\\"
                        n422 = local read "SET LAB02-1"() -> (w638:T5)
                        n423 = case shown="\"CHART TEST\", Default" w643 {
                          tunnel: ["CHART TEST-" "CYCLE TEST-" "T-RISE TEST-"] -> w639
                          frame "CHART TEST", Default {
                          }
                          frame "CYCLE TEST" {
                          }
                          frame "T-RISE TEST" {
                          }
                        }
                        n424 = Unbundle(w638) -> ("DESCRIPTION"=w637:string)  [unwired: 4 out]
                        n425 = Concatenate Strings(w633, "LAB02-1\\", w631, w629, w630, w629) -> (w640:string)
                        n426 = String To Path(string=w640) -> (path=w642:path)
                        n427 = Concatenate Strings(w640, w639, w637, "-", w636, ".tdms") -> (w628:string)
                        n428 = Create Folder(path (use dialog)=w642) -> (error out=w641:errorcluster)  [unwired: 2 in, 2 out]
                        n429 = global write "Global 1.vi" "LAB02-1 FILE"(w628) -> ()
                        n430 = call <vilib>:"Clear Errors.vi"("error in (no error)"=w641) -> ()  [unwired: 6 in, 1 out]
                      }
                      frame #1 {
                        n431 = String To Path(string=w653) -> (path=w648:path)
                        n432 = TDMS Open(5:FALSE, 6:FALSE, 10:T15."create or replace" ("operation (0:open)"), 11:w648) -> (0:w647:errorcluster, 3:→"TDMS LAB02-1":refnum<k34>)  [unwired: 3 in]
                      }
                      frame #2 {
                        n433 = local read "SET LAB02-1"() -> (w659:T5)
                        n434 = local read "TDMS LAB02-1"() -> (w670:refnum<k34>)
                        n435 = Build Array("Testers Name", "Description", "Set Test Cycles", "T-Rise minutes", "T-Rise Deg C") -> (w660:string[])
                        n436 = Unbundle(w659) -> ("NAME"=w658:string, "DESCRIPTION"=w657:string, "CYCLES"=w656:dbl, "T-RISE mins"=w655:dbl, "T-RISE deg C"=w654:dbl)
                        n437 = Number To Decimal String(number=w656) -> (decimal integer string=w669:string)  [unwired: 1 in]
                        n438 = Number To Decimal String(number=w655) -> (decimal integer string=w668:string)  [unwired: 1 in]
                        n439 = Number To Decimal String(number=w654) -> (decimal integer string=w667:string)  [unwired: 1 in]
                        n440 = Build Array(w658, w657, w669, w668, w667) -> (w666:string[])
                        n441 = TDMS Set Properties(5:w666, 7:w660, 11:w670) -> ()  [unwired: 3 in, 4 out]
                      }
                      frame #3 {
                        w672 = 0.0
                        n442 = local read "DISP LAB02-1"() -> (w674:T4)
                        n443 = Bundle(cluster=w674, "CYCLE"=w672, "MINS"=w672, "STATUS"="RUN") -> (w673:T4)
                        n444 = local write "DISP LAB02-1"(w673) -> ()
                      }
                      frame #4 {
                        n445 = local read "SIG LAB02-1"() -> (w677:T2)
                        n446 = local read "TEMP START LAB02-1"() -> (w679:cluster{"TL":dbl, "TN":dbl})
                        n447 = Unbundle(w677) -> ("Tmp Live"=w676:dbl, "Tmp Neut"=w675:dbl)  [unwired: 3 out]
                        n448 = Bundle(cluster=w679, "TL"=w676, "TN"=w675) -> (w678:cluster{"TL":dbl, "TN":dbl})
                        n449 = local write "TEMP START LAB02-1"(w678) -> ()
                      }
                    }
                  }
                }
              }
              event "RUN LAB02-2": Value Change {
                n450 = event-data() -> ("NewVal"=w680:bool)  [unwired: 1 in, 5 out]
                n451 = local write "run lab02-2"(w680) -> ()
                n452 = case shown="False" w680 {
                  tunnel: w686 -> [_ w716]
                  tunnel: w685 -> [_ w715]
                  tunnel: w683 -> [w688 w714]
                  tunnel: w684 -> [_ w713]
                  tunnel: w682 -> [_ w712]
                  tunnel: [w687 w711] -> w681
                  frame False {
                    # "stop test"
                    n453 = stacked-sequence {
                      tunnel: w688 -> [w697 _]
                      tunnel: [w689 _] -> w687
                      frame #0 {
                        n454 = local read "DISP LAB02-2"() -> (w696:T4)
                        n455 = Unbundle(w696) -> ("CYCLE"=w694:dbl, "MINS"=w695:dbl)  [unwired: 1 out]
                        n456 = case shown="\"CYCLE TEST\"" w697 {
                          tunnel: w695 -> [_ _ w704]
                          tunnel: w694 -> [w702 w703 _]
                          tunnel: [w702 w703 w704] -> w693
                          frame "CHART TEST", Default {
                          }
                          frame "CYCLE TEST" {
                          }
                          frame "T-RISE TEST" {
                          }
                        }
                        n457 = local read "TDMS LAB02-2"() -> (w701:refnum<k34>)
                        n458 = Build Array("STOPPED") -> (w698:string[])
                        n459 = Build Array(w693) -> (w692:dbl[])
                        n460 = TDMS Write(0:w701, 5:"TEST RESULT", 7:w698, 9:w692) -> (4:w690:refnum<k34>, 15:w691:errorcluster)  [unwired: 2 in, 2 out]
                        n461 = TDMS Close(8:w691, 11:w690) -> (0:w689:errorcluster)  [unwired: 1 out]
                      }
                      frame #1 {
                        n462 = local read "DISP LAB02-2"() -> (w710:T4)
                        n463 = Bundle(cluster=w710, "STATUS"="STOP") -> (w708:T4)  [unwired: 2 in]
                        n464 = call "Save data file to network drive v1.vi"("panel id"="LAB02-2") -> ("network file save error"=w705:errorcluster)  [unwired: 9 in, 1 out]
                        n465 = local write "RESULT LAB02-2"(FALSE) -> ()
                        n466 = local write "DISP LAB02-2"(w708) -> ()
                        n467 = local write "data file error"(w705) -> ()
                      }
                    }
                  }
                  frame True {
                    # "start new test and create test file"
                    n468 = stacked-sequence {
                      seq-local: [w717 _ _ _ _] -> [_ w742 _ _ _]
                      tunnel: w716 -> [w722 _ _ _ _]
                      tunnel: w715 -> [w719 _ _ _ _]
                      tunnel: w714 -> [w732 _ _ _ _]
                      tunnel: w713 -> [w725 _ _ _ _]
                      tunnel: w712 -> [w720 _ _ _ _]
                      tunnel: [_ w736 _ _ _] -> w711
                      frame #0 {
                        w718 = "\\"
                        n469 = local read "SET LAB02-2"() -> (w727:T5)
                        n470 = case shown="\"CHART TEST\", Default" w732 {
                          tunnel: ["CHART TEST-" "CYCLE TEST-" "T-RISE TEST-"] -> w728
                          frame "CHART TEST", Default {
                          }
                          frame "CYCLE TEST" {
                          }
                          frame "T-RISE TEST" {
                          }
                        }
                        n471 = Unbundle(w727) -> ("DESCRIPTION"=w726:string)  [unwired: 4 out]
                        n472 = Concatenate Strings(w722, "LAB02-2\\", w720, w718, w719, w718) -> (w729:string)
                        n473 = String To Path(string=w729) -> (path=w731:path)
                        n474 = Concatenate Strings(w729, w728, w726, "-", w725, ".tdms") -> (w717:string)
                        n475 = Create Folder(path (use dialog)=w731) -> (error out=w730:errorcluster)  [unwired: 2 in, 2 out]
                        n476 = global write "Global 1.vi" "LAB02-2 FILE"(w717) -> ()
                        n477 = call <vilib>:"Clear Errors.vi"("error in (no error)"=w730) -> ()  [unwired: 6 in, 1 out]
                      }
                      frame #1 {
                        n478 = String To Path(string=w742) -> (path=w737:path)
                        n479 = TDMS Open(5:FALSE, 6:FALSE, 10:T15."create or replace" ("operation (0:open)"), 11:w737) -> (0:w736:errorcluster, 3:→"TDMS LAB02-2":refnum<k34>)  [unwired: 3 in]
                      }
                      frame #2 {
                        n480 = local read "SET LAB02-2"() -> (w748:T5)
                        n481 = local read "TDMS LAB02-2"() -> (w759:refnum<k34>)
                        n482 = Build Array("Testers Name", "Description", "Set Test Cycles", "T-Rise minutes", "T-Rise Deg C") -> (w749:string[])
                        n483 = Unbundle(w748) -> ("NAME"=w747:string, "DESCRIPTION"=w746:string, "CYCLES"=w745:dbl, "T-RISE mins"=w744:dbl, "T-RISE deg C"=w743:dbl)
                        n484 = Number To Decimal String(number=w745) -> (decimal integer string=w758:string)  [unwired: 1 in]
                        n485 = Number To Decimal String(number=w744) -> (decimal integer string=w757:string)  [unwired: 1 in]
                        n486 = Number To Decimal String(number=w743) -> (decimal integer string=w756:string)  [unwired: 1 in]
                        n487 = Build Array(w747, w746, w758, w757, w756) -> (w755:string[])
                        n488 = TDMS Set Properties(5:w755, 7:w749, 11:w759) -> ()  [unwired: 3 in, 4 out]
                      }
                      frame #3 {
                        w761 = 0.0
                        n489 = local read "DISP LAB02-2"() -> (w763:T4)
                        n490 = Bundle(cluster=w763, "CYCLE"=w761, "MINS"=w761, "STATUS"="RUN") -> (w762:T4)
                        n491 = local write "DISP LAB02-2"(w762) -> ()
                      }
                      frame #4 {
                        n492 = local read "SIG LAB02-2"() -> (w766:T2)
                        n493 = local read "TEMP START LAB02-2"() -> (w768:cluster{"TL":dbl, "TN":dbl})
                        n494 = Unbundle(w766) -> ("Tmp Live"=w765:dbl, "Tmp Neut"=w764:dbl)  [unwired: 3 out]
                        n495 = Bundle(cluster=w768, "TL"=w765, "TN"=w764) -> (w767:cluster{"TL":dbl, "TN":dbl})
                        n496 = local write "TEMP START LAB02-2"(w767) -> ()
                      }
                    }
                  }
                }
              }
              event "RUN LAB03-1": Value Change {
                n497 = event-data() -> ("NewVal"=w769:bool)  [unwired: 1 in, 5 out]
                n498 = local write "run lab03-1"(w769) -> ()
                n499 = case shown="False" w769 {
                  tunnel: w775 -> [_ w805]
                  tunnel: w774 -> [_ w804]
                  tunnel: w772 -> [w777 w803]
                  tunnel: w773 -> [_ w802]
                  tunnel: w771 -> [_ w801]
                  tunnel: [w776 w800] -> w770
                  frame False {
                    # "stop test"
                    n500 = stacked-sequence {
                      tunnel: w777 -> [w786 _]
                      tunnel: [w778 _] -> w776
                      frame #0 {
                        n501 = local read "DISP LAB03-1"() -> (w785:T4)
                        n502 = Unbundle(w785) -> ("CYCLE"=w783:dbl, "MINS"=w784:dbl)  [unwired: 1 out]
                        n503 = case shown="\"CYCLE TEST\"" w786 {
                          tunnel: w784 -> [_ _ w793]
                          tunnel: w783 -> [w791 w792 _]
                          tunnel: [w791 w792 w793] -> w782
                          frame "CHART TEST", Default {
                          }
                          frame "CYCLE TEST" {
                          }
                          frame "T-RISE TEST" {
                          }
                        }
                        n504 = local read "TDMS LAB03-1"() -> (w790:refnum<k34>)
                        n505 = Build Array("STOPPED") -> (w787:string[])
                        n506 = Build Array(w782) -> (w781:dbl[])
                        n507 = TDMS Write(0:w790, 5:"TEST RESULT", 7:w787, 9:w781) -> (4:w779:refnum<k34>, 15:w780:errorcluster)  [unwired: 2 in, 2 out]
                        n508 = TDMS Close(8:w780, 11:w779) -> (0:w778:errorcluster)  [unwired: 1 out]
                      }
                      frame #1 {
                        n509 = local read "DISP LAB03-1"() -> (w799:T4)
                        n510 = Bundle(cluster=w799, "STATUS"="STOP") -> (w797:T4)  [unwired: 2 in]
                        n511 = call "Save data file to network drive v1.vi"("panel id"="LAB03-1") -> ("network file save error"=w794:errorcluster)  [unwired: 9 in, 1 out]
                        n512 = local write "RESULT LAB03-1"(FALSE) -> ()
                        n513 = local write "data file error"(w794) -> ()
                        n514 = local write "DISP LAB03-1"(w797) -> ()
                      }
                    }
                  }
                  frame True {
                    # "start new test and create test file"
                    n515 = stacked-sequence {
                      seq-local: [w806 _ _ _ _] -> [_ w831 _ _ _]
                      tunnel: w805 -> [w811 _ _ _ _]
                      tunnel: w804 -> [w808 _ _ _ _]
                      tunnel: w803 -> [w821 _ _ _ _]
                      tunnel: w802 -> [w814 _ _ _ _]
                      tunnel: w801 -> [w809 _ _ _ _]
                      tunnel: [_ w825 _ _ _] -> w800
                      frame #0 {
                        w807 = "\\"
                        n516 = local read "SET LAB03-1"() -> (w816:T5)
                        n517 = case shown="\"CHART TEST\", Default" w821 {
                          tunnel: ["CHART TEST-" "CYCLE TEST-" "T-RISE TEST-"] -> w817
                          frame "CHART TEST", Default {
                          }
                          frame "CYCLE TEST" {
                          }
                          frame "T-RISE TEST" {
                          }
                        }
                        n518 = Unbundle(w816) -> ("DESCRIPTION"=w815:string)  [unwired: 4 out]
                        n519 = Concatenate Strings(w811, "LAB03-1\\", w809, w807, w808, w807) -> (w818:string)
                        n520 = String To Path(string=w818) -> (path=w820:path)
                        n521 = Concatenate Strings(w818, w817, w815, "-", w814, ".tdms") -> (w806:string)
                        n522 = Create Folder(path (use dialog)=w820) -> (error out=w819:errorcluster)  [unwired: 2 in, 2 out]
                        n523 = global write "Global 1.vi" "LAB03-1 FILE"(w806) -> ()
                        n524 = call <vilib>:"Clear Errors.vi"("error in (no error)"=w819) -> ()  [unwired: 6 in, 1 out]
                      }
                      frame #1 {
                        n525 = String To Path(string=w831) -> (path=w826:path)
                        n526 = TDMS Open(5:FALSE, 6:FALSE, 10:T15."create or replace" ("operation (0:open)"), 11:w826) -> (0:w825:errorcluster, 3:→"TDMS LAB03-1":refnum<k34>)  [unwired: 3 in]
                      }
                      frame #2 {
                        n527 = local read "SET LAB03-1"() -> (w837:T5)
                        n528 = local read "TDMS LAB03-1"() -> (w848:refnum<k34>)
                        n529 = Build Array("Testers Name", "Description", "Set Test Cycles", "T-Rise minutes", "T-Rise Deg C") -> (w838:string[])
                        n530 = Unbundle(w837) -> ("NAME"=w836:string, "DESCRIPTION"=w835:string, "CYCLES"=w834:dbl, "T-RISE mins"=w833:dbl, "T-RISE deg C"=w832:dbl)
                        n531 = Number To Decimal String(number=w834) -> (decimal integer string=w847:string)  [unwired: 1 in]
                        n532 = Number To Decimal String(number=w833) -> (decimal integer string=w846:string)  [unwired: 1 in]
                        n533 = Number To Decimal String(number=w832) -> (decimal integer string=w845:string)  [unwired: 1 in]
                        n534 = Build Array(w836, w835, w847, w846, w845) -> (w844:string[])
                        n535 = TDMS Set Properties(5:w844, 7:w838, 11:w848) -> ()  [unwired: 3 in, 4 out]
                      }
                      frame #3 {
                        w850 = 0.0
                        n536 = local read "DISP LAB03-1"() -> (w852:T4)
                        n537 = Bundle(cluster=w852, "CYCLE"=w850, "MINS"=w850, "STATUS"="RUN") -> (w851:T4)
                        n538 = local write "DISP LAB03-1"(w851) -> ()
                      }
                      frame #4 {
                        n539 = local read "SIG LAB03-1"() -> (w855:T2)
                        n540 = local read "TEMP START LAB03-1"() -> (w857:cluster{"TL":dbl, "TN":dbl})
                        n541 = Unbundle(w855) -> ("Tmp Live"=w854:dbl, "Tmp Neut"=w853:dbl)  [unwired: 3 out]
                        n542 = Bundle(cluster=w857, "TL"=w854, "TN"=w853) -> (w856:cluster{"TL":dbl, "TN":dbl})
                        n543 = local write "TEMP START LAB03-1"(w856) -> ()
                      }
                    }
                  }
                }
              }
              event "RUN LAB03-2": Value Change {
                n544 = event-data() -> ("NewVal"=w858:bool)  [unwired: 1 in, 5 out]
                n545 = local write "run lab03-2"(w858) -> ()
                n546 = case shown="False" w858 {
                  tunnel: w864 -> [_ w894]
                  tunnel: w863 -> [_ w893]
                  tunnel: w861 -> [w866 w892]
                  tunnel: w862 -> [_ w891]
                  tunnel: w860 -> [_ w890]
                  tunnel: [w865 w889] -> w859
                  frame False {
                    # "stop test"
                    n547 = stacked-sequence {
                      tunnel: w866 -> [w875 _]
                      tunnel: [w867 _] -> w865
                      frame #0 {
                        n548 = local read "DISP LAB03-2"() -> (w874:T4)
                        n549 = Unbundle(w874) -> ("CYCLE"=w872:dbl, "MINS"=w873:dbl)  [unwired: 1 out]
                        n550 = case shown="\"CYCLE TEST\"" w875 {
                          tunnel: w873 -> [_ _ w882]
                          tunnel: w872 -> [w880 w881 _]
                          tunnel: [w880 w881 w882] -> w871
                          frame "CHART TEST", Default {
                          }
                          frame "CYCLE TEST" {
                          }
                          frame "T-RISE TEST" {
                          }
                        }
                        n551 = local read "TDMS LAB03-2"() -> (w879:refnum<k34>)
                        n552 = Build Array("STOPPED") -> (w876:string[])
                        n553 = Build Array(w871) -> (w870:dbl[])
                        n554 = TDMS Write(0:w879, 5:"TEST RESULT", 7:w876, 9:w870) -> (4:w868:refnum<k34>, 15:w869:errorcluster)  [unwired: 2 in, 2 out]
                        n555 = TDMS Close(8:w869, 11:w868) -> (0:w867:errorcluster)  [unwired: 1 out]
                      }
                      frame #1 {
                        n556 = local read "DISP LAB03-2"() -> (w888:T4)
                        n557 = Bundle(cluster=w888, "STATUS"="STOP") -> (w886:T4)  [unwired: 2 in]
                        n558 = call "Save data file to network drive v1.vi"("panel id"="LAB03-2") -> ("network file save error"=w883:errorcluster)  [unwired: 9 in, 1 out]
                        n559 = local write "RESULT LAB03-2"(FALSE) -> ()
                        n560 = local write "DISP LAB03-2"(w886) -> ()
                        n561 = local write "data file error"(w883) -> ()
                      }
                    }
                  }
                  frame True {
                    # "start new test and create test file"
                    n562 = stacked-sequence {
                      seq-local: [w895 _ _ _ _] -> [_ w920 _ _ _]
                      tunnel: w894 -> [w900 _ _ _ _]
                      tunnel: w893 -> [w897 _ _ _ _]
                      tunnel: w892 -> [w910 _ _ _ _]
                      tunnel: w891 -> [w903 _ _ _ _]
                      tunnel: w890 -> [w898 _ _ _ _]
                      tunnel: [_ w914 _ _ _] -> w889
                      frame #0 {
                        w896 = "\\"
                        n563 = local read "SET LAB03-2"() -> (w905:T5)
                        n564 = case shown="\"CHART TEST\", Default" w910 {
                          tunnel: ["CHART TEST-" "CYCLE TEST-" "T-RISE TEST-"] -> w906
                          frame "CHART TEST", Default {
                          }
                          frame "CYCLE TEST" {
                          }
                          frame "T-RISE TEST" {
                          }
                        }
                        n565 = Unbundle(w905) -> ("DESCRIPTION"=w904:string)  [unwired: 4 out]
                        n566 = Concatenate Strings(w900, "LAB03-2\\", w898, w896, w897, w896) -> (w907:string)
                        n567 = String To Path(string=w907) -> (path=w909:path)
                        n568 = Concatenate Strings(w907, w906, w904, "-", w903, ".tdms") -> (w895:string)
                        n569 = Create Folder(path (use dialog)=w909) -> (error out=w908:errorcluster)  [unwired: 2 in, 2 out]
                        n570 = global write "Global 1.vi" "LAB03-2 FILE"(w895) -> ()
                        n571 = call <vilib>:"Clear Errors.vi"("error in (no error)"=w908) -> ()  [unwired: 6 in, 1 out]
                      }
                      frame #1 {
                        n572 = String To Path(string=w920) -> (path=w915:path)
                        n573 = TDMS Open(5:FALSE, 6:FALSE, 10:T15."create or replace" ("operation (0:open)"), 11:w915) -> (0:w914:errorcluster, 3:→"TDMS LAB03-2":refnum<k34>)  [unwired: 3 in]
                      }
                      frame #2 {
                        n574 = local read "SET LAB03-2"() -> (w926:T5)
                        n575 = local read "TDMS LAB03-2"() -> (w937:refnum<k34>)
                        n576 = Build Array("Testers Name", "Description", "Set Test Cycles", "T-Rise minutes", "T-Rise Deg C") -> (w927:string[])
                        n577 = Unbundle(w926) -> ("NAME"=w925:string, "DESCRIPTION"=w924:string, "CYCLES"=w923:dbl, "T-RISE mins"=w922:dbl, "T-RISE deg C"=w921:dbl)
                        n578 = Number To Decimal String(number=w923) -> (decimal integer string=w936:string)  [unwired: 1 in]
                        n579 = Number To Decimal String(number=w922) -> (decimal integer string=w935:string)  [unwired: 1 in]
                        n580 = Number To Decimal String(number=w921) -> (decimal integer string=w934:string)  [unwired: 1 in]
                        n581 = Build Array(w925, w924, w936, w935, w934) -> (w933:string[])
                        n582 = TDMS Set Properties(5:w933, 7:w927, 11:w937) -> ()  [unwired: 3 in, 4 out]
                      }
                      frame #3 {
                        w939 = 0.0
                        n583 = local read "DISP LAB03-2"() -> (w941:T4)
                        n584 = Bundle(cluster=w941, "CYCLE"=w939, "MINS"=w939, "STATUS"="RUN") -> (w940:T4)
                        n585 = local write "DISP LAB03-2"(w940) -> ()
                      }
                      frame #4 {
                        n586 = local read "SIG LAB03-2"() -> (w944:T2)
                        n587 = local read "TEMP START LAB03-2"() -> (w946:cluster{"TL":dbl, "TN":dbl})
                        n588 = Unbundle(w944) -> ("Tmp Live"=w943:dbl, "Tmp Neut"=w942:dbl)  [unwired: 3 out]
                        n589 = Bundle(cluster=w946, "TL"=w943, "TN"=w942) -> (w945:cluster{"TL":dbl, "TN":dbl})
                        n590 = local write "TEMP START LAB03-2"(w945) -> ()
                      }
                    }
                  }
                }
              }
              event "RUN LAB04-1": Value Change {
                n591 = event-data() -> ("NewVal"=w947:bool)  [unwired: 1 in, 5 out]
                n592 = local write "run lab04-1"(w947) -> ()
                n593 = case shown="False" w947 {
                  tunnel: w953 -> [_ w983]
                  tunnel: w952 -> [_ w982]
                  tunnel: w950 -> [w955 w981]
                  tunnel: w951 -> [_ w980]
                  tunnel: w949 -> [_ w979]
                  tunnel: [w954 w978] -> w948
                  frame False {
                    # "stop test"
                    n594 = stacked-sequence {
                      tunnel: w955 -> [w964 _]
                      tunnel: [w956 _] -> w954
                      frame #0 {
                        n595 = local read "DISP LAB04-1"() -> (w963:T4)
                        n596 = Unbundle(w963) -> ("CYCLE"=w961:dbl, "MINS"=w962:dbl)  [unwired: 1 out]
                        n597 = case shown="\"CYCLE TEST\"" w964 {
                          tunnel: w962 -> [_ _ w971]
                          tunnel: w961 -> [w969 w970 _]
                          tunnel: [w969 w970 w971] -> w960
                          frame "CHART TEST", Default {
                          }
                          frame "CYCLE TEST" {
                          }
                          frame "T-RISE TEST" {
                          }
                        }
                        n598 = local read "TDMS LAB04-1"() -> (w968:refnum<k34>)
                        n599 = Build Array("STOPPED") -> (w965:string[])
                        n600 = Build Array(w960) -> (w959:dbl[])
                        n601 = TDMS Write(0:w968, 5:"TEST RESULT", 7:w965, 9:w959) -> (4:w957:refnum<k34>, 15:w958:errorcluster)  [unwired: 2 in, 2 out]
                        n602 = TDMS Close(8:w958, 11:w957) -> (0:w956:errorcluster)  [unwired: 1 out]
                      }
                      frame #1 {
                        n603 = local read "DISP LAB04-1"() -> (w977:T4)
                        n604 = Bundle(cluster=w977, "STATUS"="STOP") -> (w975:T4)  [unwired: 2 in]
                        n605 = call "Save data file to network drive v1.vi"("panel id"="LAB04-1") -> ("network file save error"=w972:errorcluster)  [unwired: 9 in, 1 out]
                        n606 = local write "RESULT LAB04-1"(FALSE) -> ()
                        n607 = local write "DISP LAB04-1"(w975) -> ()
                        n608 = local write "data file error"(w972) -> ()
                      }
                    }
                  }
                  frame True {
                    # "start new test and create test file"
                    n609 = stacked-sequence {
                      seq-local: [w984 _ _ _ _] -> [_ w1009 _ _ _]
                      tunnel: w983 -> [w989 _ _ _ _]
                      tunnel: w982 -> [w985 _ _ _ _]
                      tunnel: w981 -> [w999 _ _ _ _]
                      tunnel: w980 -> [w992 _ _ _ _]
                      tunnel: w979 -> [w987 _ _ _ _]
                      tunnel: [_ w1003 _ _ _] -> w978
                      frame #0 {
                        w986 = "\\"
                        n610 = local read "SET LAB04-1"() -> (w994:T5)
                        n611 = case shown="\"CHART TEST\", Default" w999 {
                          tunnel: ["CHART TEST-" "CYCLE TEST-" "T-RISE TEST-"] -> w995
                          frame "CHART TEST", Default {
                          }
                          frame "CYCLE TEST" {
                          }
                          frame "T-RISE TEST" {
                          }
                        }
                        n612 = Unbundle(w994) -> ("DESCRIPTION"=w993:string)  [unwired: 4 out]
                        n613 = Concatenate Strings(w989, "LAB04-1\\", w987, w986, w985, w986) -> (w996:string)
                        n614 = String To Path(string=w996) -> (path=w998:path)
                        n615 = Concatenate Strings(w996, w995, w993, "-", w992, ".tdms") -> (w984:string)
                        n616 = Create Folder(path (use dialog)=w998) -> (error out=w997:errorcluster)  [unwired: 2 in, 2 out]
                        n617 = global write "Global 1.vi" "LAB04-1 FILE"(w984) -> ()
                        n618 = call <vilib>:"Clear Errors.vi"("error in (no error)"=w997) -> ()  [unwired: 6 in, 1 out]
                      }
                      frame #1 {
                        n619 = String To Path(string=w1009) -> (path=w1004:path)
                        n620 = TDMS Open(5:FALSE, 6:FALSE, 10:T15."create or replace" ("operation (0:open)"), 11:w1004) -> (0:w1003:errorcluster, 3:→"TDMS LAB04-1":refnum<k34>)  [unwired: 3 in]
                      }
                      frame #2 {
                        n621 = local read "SET LAB04-1"() -> (w1015:T5)
                        n622 = local read "TDMS LAB04-1"() -> (w1026:refnum<k34>)
                        n623 = Build Array("Testers Name", "Description", "Set Test Cycles", "T-Rise minutes", "T-Rise Deg C") -> (w1016:string[])
                        n624 = Unbundle(w1015) -> ("NAME"=w1014:string, "DESCRIPTION"=w1013:string, "CYCLES"=w1012:dbl, "T-RISE mins"=w1011:dbl, "T-RISE deg C"=w1010:dbl)
                        n625 = Number To Decimal String(number=w1012) -> (decimal integer string=w1025:string)  [unwired: 1 in]
                        n626 = Number To Decimal String(number=w1011) -> (decimal integer string=w1024:string)  [unwired: 1 in]
                        n627 = Number To Decimal String(number=w1010) -> (decimal integer string=w1023:string)  [unwired: 1 in]
                        n628 = Build Array(w1014, w1013, w1025, w1024, w1023) -> (w1022:string[])
                        n629 = TDMS Set Properties(5:w1022, 7:w1016, 11:w1026) -> ()  [unwired: 3 in, 4 out]
                      }
                      frame #3 {
                        w1028 = 0.0
                        n630 = local read "DISP LAB04-1"() -> (w1030:T4)
                        n631 = Bundle(cluster=w1030, "CYCLE"=w1028, "MINS"=w1028, "STATUS"="RUN") -> (w1029:T4)
                        n632 = local write "DISP LAB04-1"(w1029) -> ()
                      }
                      frame #4 {
                        n633 = local read "SIG LAB04-1"() -> (w1033:T2)
                        n634 = local read "TEMP START LAB04-1"() -> (w1035:cluster{"TL":dbl, "TN":dbl})
                        n635 = Unbundle(w1033) -> ("Tmp Live"=w1032:dbl, "Tmp Neut"=w1031:dbl)  [unwired: 3 out]
                        n636 = Bundle(cluster=w1035, "TL"=w1032, "TN"=w1031) -> (w1034:cluster{"TL":dbl, "TN":dbl})
                        n637 = local write "TEMP START LAB04-1"(w1034) -> ()
                      }
                    }
                  }
                }
              }
              event "RUN LAB04-2": Value Change {
                n638 = event-data() -> ("NewVal"=w1036:bool)  [unwired: 1 in, 5 out]
                n639 = local write "run lab04-2"(w1036) -> ()
                n640 = case shown="False" w1036 {
                  tunnel: w1042 -> [_ w1072]
                  tunnel: w1041 -> [_ w1071]
                  tunnel: w1039 -> [w1044 w1070]
                  tunnel: w1040 -> [_ w1069]
                  tunnel: w1038 -> [_ w1068]
                  tunnel: [w1043 w1067] -> w1037
                  frame False {
                    # "stop test"
                    n641 = stacked-sequence {
                      tunnel: w1044 -> [w1053 _]
                      tunnel: [w1045 _] -> w1043
                      frame #0 {
                        n642 = local read "DISP LAB04-2"() -> (w1052:T4)
                        n643 = Unbundle(w1052) -> ("CYCLE"=w1050:dbl, "MINS"=w1051:dbl)  [unwired: 1 out]
                        n644 = case shown="\"CYCLE TEST\"" w1053 {
                          tunnel: w1051 -> [_ _ w1060]
                          tunnel: w1050 -> [w1058 w1059 _]
                          tunnel: [w1058 w1059 w1060] -> w1049
                          frame "CHART TEST", Default {
                          }
                          frame "CYCLE TEST" {
                          }
                          frame "T-RISE TEST" {
                          }
                        }
                        n645 = local read "TDMS LAB04-2"() -> (w1057:refnum<k34>)
                        n646 = Build Array("STOPPED") -> (w1054:string[])
                        n647 = Build Array(w1049) -> (w1048:dbl[])
                        n648 = TDMS Write(0:w1057, 5:"TEST RESULT", 7:w1054, 9:w1048) -> (4:w1046:refnum<k34>, 15:w1047:errorcluster)  [unwired: 2 in, 2 out]
                        n649 = TDMS Close(8:w1047, 11:w1046) -> (0:w1045:errorcluster)  [unwired: 1 out]
                      }
                      frame #1 {
                        n650 = local read "DISP LAB04-2"() -> (w1066:T4)
                        n651 = Bundle(cluster=w1066, "STATUS"="STOP") -> (w1064:T4)  [unwired: 2 in]
                        n652 = call "Save data file to network drive v1.vi"("panel id"="LAB04-2") -> ("network file save error"=w1061:errorcluster)  [unwired: 9 in, 1 out]
                        n653 = local write "RESULT LAB04-2"(FALSE) -> ()
                        n654 = local write "DISP LAB04-2"(w1064) -> ()
                        n655 = local write "data file error"(w1061) -> ()
                      }
                    }
                  }
                  frame True {
                    # "start new test and create test file"
                    n656 = stacked-sequence {
                      seq-local: [w1073 _ _ _ _] -> [_ w1098 _ _ _]
                      tunnel: w1072 -> [w1078 _ _ _ _]
                      tunnel: w1071 -> [w1074 _ _ _ _]
                      tunnel: w1070 -> [w1088 _ _ _ _]
                      tunnel: w1069 -> [w1081 _ _ _ _]
                      tunnel: w1068 -> [w1076 _ _ _ _]
                      tunnel: [_ w1092 _ _ _] -> w1067
                      frame #0 {
                        w1075 = "\\"
                        n657 = local read "SET LAB04-2"() -> (w1083:T5)
                        n658 = case shown="\"CHART TEST\", Default" w1088 {
                          tunnel: ["CHART TEST-" "CYCLE TEST-" "T-RISE TEST-"] -> w1084
                          frame "CHART TEST", Default {
                          }
                          frame "CYCLE TEST" {
                          }
                          frame "T-RISE TEST" {
                          }
                        }
                        n659 = Unbundle(w1083) -> ("DESCRIPTION"=w1082:string)  [unwired: 4 out]
                        n660 = Concatenate Strings(w1078, "LAB04-2\\", w1076, w1075, w1074, w1075) -> (w1085:string)
                        n661 = String To Path(string=w1085) -> (path=w1087:path)
                        n662 = Concatenate Strings(w1085, w1084, w1082, "-", w1081, ".tdms") -> (w1073:string)
                        n663 = Create Folder(path (use dialog)=w1087) -> (error out=w1086:errorcluster)  [unwired: 2 in, 2 out]
                        n664 = global write "Global 1.vi" "LAB04-2 FILE"(w1073) -> ()
                        n665 = call <vilib>:"Clear Errors.vi"("error in (no error)"=w1086) -> ()  [unwired: 6 in, 1 out]
                      }
                      frame #1 {
                        n666 = String To Path(string=w1098) -> (path=w1093:path)
                        n667 = TDMS Open(5:FALSE, 6:FALSE, 10:T15."create or replace" ("operation (0:open)"), 11:w1093) -> (0:w1092:errorcluster, 3:→"TDMS LAB04-2":refnum<k34>)  [unwired: 3 in]
                      }
                      frame #2 {
                        n668 = local read "SET LAB04-2"() -> (w1104:T5)
                        n669 = local read "TDMS LAB04-2"() -> (w1115:refnum<k34>)
                        n670 = Build Array("Testers Name", "Description", "Set Test Cycles", "T-Rise minutes", "T-Rise Deg C") -> (w1105:string[])
                        n671 = Unbundle(w1104) -> ("NAME"=w1103:string, "DESCRIPTION"=w1102:string, "CYCLES"=w1101:dbl, "T-RISE mins"=w1100:dbl, "T-RISE deg C"=w1099:dbl)
                        n672 = Number To Decimal String(number=w1101) -> (decimal integer string=w1114:string)  [unwired: 1 in]
                        n673 = Number To Decimal String(number=w1100) -> (decimal integer string=w1113:string)  [unwired: 1 in]
                        n674 = Number To Decimal String(number=w1099) -> (decimal integer string=w1112:string)  [unwired: 1 in]
                        n675 = Build Array(w1103, w1102, w1114, w1113, w1112) -> (w1111:string[])
                        n676 = TDMS Set Properties(5:w1111, 7:w1105, 11:w1115) -> ()  [unwired: 3 in, 4 out]
                      }
                      frame #3 {
                        w1117 = 0.0
                        n677 = local read "DISP LAB04-2"() -> (w1119:T4)
                        n678 = Bundle(cluster=w1119, "CYCLE"=w1117, "MINS"=w1117, "STATUS"="RUN") -> (w1118:T4)
                        n679 = local write "DISP LAB04-2"(w1118) -> ()
                      }
                      frame #4 {
                        n680 = local read "SIG LAB04-2"() -> (w1122:T2)
                        n681 = local read "TEMP START LAB04-2"() -> (w1124:cluster{"TL":dbl, "TN":dbl})
                        n682 = Unbundle(w1122) -> ("Tmp Live"=w1121:dbl, "Tmp Neut"=w1120:dbl)  [unwired: 3 out]
                        n683 = Bundle(cluster=w1124, "TL"=w1121, "TN"=w1120) -> (w1123:cluster{"TL":dbl, "TN":dbl})
                        n684 = local write "TEMP START LAB04-2"(w1123) -> ()
                      }
                    }
                  }
                }
              }
              event "RUN LAB05-1": Value Change {
                n685 = event-data() -> ("NewVal"=w1125:bool)  [unwired: 1 in, 5 out]
                n686 = local write "run lab05-1"(w1125) -> ()
                n687 = case shown="False" w1125 {
                  tunnel: w1131 -> [_ w1161]
                  tunnel: w1130 -> [_ w1160]
                  tunnel: w1128 -> [w1133 w1159]
                  tunnel: w1129 -> [_ w1158]
                  tunnel: w1127 -> [_ w1157]
                  tunnel: [w1132 w1156] -> w1126
                  frame False {
                    # "stop test"
                    n688 = stacked-sequence {
                      tunnel: w1133 -> [w1142 _]
                      tunnel: [w1134 _] -> w1132
                      frame #0 {
                        n689 = local read "DISP LAB05-1"() -> (w1141:T4)
                        n690 = Unbundle(w1141) -> ("CYCLE"=w1139:dbl, "MINS"=w1140:dbl)  [unwired: 1 out]
                        n691 = case shown="\"CYCLE TEST\"" w1142 {
                          tunnel: w1140 -> [_ _ w1149]
                          tunnel: w1139 -> [w1147 w1148 _]
                          tunnel: [w1147 w1148 w1149] -> w1138
                          frame "CHART TEST", Default {
                          }
                          frame "CYCLE TEST" {
                          }
                          frame "T-RISE TEST" {
                          }
                        }
                        n692 = local read "TDMS LAB05-1"() -> (w1146:refnum<k34>)
                        n693 = Build Array("STOPPED") -> (w1143:string[])
                        n694 = Build Array(w1138) -> (w1137:dbl[])
                        n695 = TDMS Write(0:w1146, 5:"TEST RESULT", 7:w1143, 9:w1137) -> (4:w1135:refnum<k34>, 15:w1136:errorcluster)  [unwired: 2 in, 2 out]
                        n696 = TDMS Close(8:w1136, 11:w1135) -> (0:w1134:errorcluster)  [unwired: 1 out]
                      }
                      frame #1 {
                        n697 = local read "DISP LAB05-1"() -> (w1155:T4)
                        n698 = Bundle(cluster=w1155, "STATUS"="STOP") -> (w1153:T4)  [unwired: 2 in]
                        n699 = call "Save data file to network drive v1.vi"("panel id"="LAB05-1") -> ("network file save error"=w1150:errorcluster)  [unwired: 9 in, 1 out]
                        n700 = local write "RESULT LAB05-1"(FALSE) -> ()
                        n701 = local write "DISP LAB05-1"(w1153) -> ()
                        n702 = local write "data file error"(w1150) -> ()
                      }
                    }
                  }
                  frame True {
                    # "start new test and create test file"
                    n703 = stacked-sequence {
                      seq-local: [w1162 _ _ _ _] -> [_ w1187 _ _ _]
                      tunnel: w1161 -> [w1167 _ _ _ _]
                      tunnel: w1160 -> [w1163 _ _ _ _]
                      tunnel: w1159 -> [w1177 _ _ _ _]
                      tunnel: w1158 -> [w1170 _ _ _ _]
                      tunnel: w1157 -> [w1165 _ _ _ _]
                      tunnel: [_ w1181 _ _ _] -> w1156
                      frame #0 {
                        w1164 = "\\"
                        n704 = local read "SET LAB05-1"() -> (w1172:T5)
                        n705 = case shown="\"CHART TEST\", Default" w1177 {
                          tunnel: ["CHART TEST-" "CYCLE TEST-" "T-RISE TEST-"] -> w1173
                          frame "CHART TEST", Default {
                          }
                          frame "CYCLE TEST" {
                          }
                          frame "T-RISE TEST" {
                          }
                        }
                        n706 = Unbundle(w1172) -> ("DESCRIPTION"=w1171:string)  [unwired: 4 out]
                        n707 = Concatenate Strings(w1167, "LAB05-1\\", w1165, w1164, w1163, w1164) -> (w1174:string)
                        n708 = String To Path(string=w1174) -> (path=w1176:path)
                        n709 = Concatenate Strings(w1174, w1173, w1171, "-", w1170, ".tdms") -> (w1162:string)
                        n710 = Create Folder(path (use dialog)=w1176) -> (error out=w1175:errorcluster)  [unwired: 2 in, 2 out]
                        n711 = global write "Global 1.vi" "LAB05-1 FILE"(w1162) -> ()
                        n712 = call <vilib>:"Clear Errors.vi"("error in (no error)"=w1175) -> ()  [unwired: 6 in, 1 out]
                      }
                      frame #1 {
                        n713 = String To Path(string=w1187) -> (path=w1182:path)
                        n714 = TDMS Open(5:FALSE, 6:FALSE, 10:T15."create or replace" ("operation (0:open)"), 11:w1182) -> (0:w1181:errorcluster, 3:→"TDMS LAB05-1":refnum<k34>)  [unwired: 3 in]
                      }
                      frame #2 {
                        n715 = local read "SET LAB05-1"() -> (w1193:T5)
                        n716 = local read "TDMS LAB05-1"() -> (w1204:refnum<k34>)
                        n717 = Build Array("Testers Name", "Description", "Set Test Cycles", "T-Rise minutes", "T-Rise Deg C") -> (w1194:string[])
                        n718 = Unbundle(w1193) -> ("NAME"=w1192:string, "DESCRIPTION"=w1191:string, "CYCLES"=w1190:dbl, "T-RISE mins"=w1189:dbl, "T-RISE deg C"=w1188:dbl)
                        n719 = Number To Decimal String(number=w1190) -> (decimal integer string=w1203:string)  [unwired: 1 in]
                        n720 = Number To Decimal String(number=w1189) -> (decimal integer string=w1202:string)  [unwired: 1 in]
                        n721 = Number To Decimal String(number=w1188) -> (decimal integer string=w1201:string)  [unwired: 1 in]
                        n722 = Build Array(w1192, w1191, w1203, w1202, w1201) -> (w1200:string[])
                        n723 = TDMS Set Properties(5:w1200, 7:w1194, 11:w1204) -> ()  [unwired: 3 in, 4 out]
                      }
                      frame #3 {
                        w1206 = 0.0
                        n724 = local read "DISP LAB05-1"() -> (w1208:T4)
                        n725 = Bundle(cluster=w1208, "CYCLE"=w1206, "MINS"=w1206, "STATUS"="RUN") -> (w1207:T4)
                        n726 = local write "DISP LAB05-1"(w1207) -> ()
                      }
                      frame #4 {
                        n727 = local read "SIG LAB05-1"() -> (w1211:T2)
                        n728 = local read "TEMP START LAB05-1"() -> (w1213:cluster{"TL":dbl, "TN":dbl})
                        n729 = Unbundle(w1211) -> ("Tmp Live"=w1210:dbl, "Tmp Neut"=w1209:dbl)  [unwired: 3 out]
                        n730 = Bundle(cluster=w1213, "TL"=w1210, "TN"=w1209) -> (w1212:cluster{"TL":dbl, "TN":dbl})
                        n731 = local write "TEMP START LAB05-1"(w1212) -> ()
                      }
                    }
                  }
                }
              }
              event "RUN LAB05-2": Value Change {
                n732 = event-data() -> ("NewVal"=w1214:bool)  [unwired: 1 in, 5 out]
                n733 = local write "run lab05-2"(w1214) -> ()
                n734 = case shown="False" w1214 {
                  tunnel: w1220 -> [_ w1250]
                  tunnel: w1219 -> [_ w1249]
                  tunnel: w1217 -> [w1222 w1248]
                  tunnel: w1218 -> [_ w1247]
                  tunnel: w1216 -> [_ w1246]
                  tunnel: [w1221 w1245] -> w1215
                  frame False {
                    # "stop test"
                    n735 = stacked-sequence {
                      tunnel: w1222 -> [w1231 _]
                      tunnel: [w1223 _] -> w1221
                      frame #0 {
                        n736 = local read "DISP LAB05-2"() -> (w1230:T4)
                        n737 = Unbundle(w1230) -> ("CYCLE"=w1228:dbl, "MINS"=w1229:dbl)  [unwired: 1 out]
                        n738 = case shown="\"CYCLE TEST\"" w1231 {
                          tunnel: w1229 -> [_ _ w1238]
                          tunnel: w1228 -> [w1236 w1237 _]
                          tunnel: [w1236 w1237 w1238] -> w1227
                          frame "CHART TEST", Default {
                          }
                          frame "CYCLE TEST" {
                          }
                          frame "T-RISE TEST" {
                          }
                        }
                        n739 = local read "TDMS LAB05-2"() -> (w1235:refnum<k34>)
                        n740 = Build Array("STOPPED") -> (w1232:string[])
                        n741 = Build Array(w1227) -> (w1226:dbl[])
                        n742 = TDMS Write(0:w1235, 5:"TEST RESULT", 7:w1232, 9:w1226) -> (4:w1224:refnum<k34>, 15:w1225:errorcluster)  [unwired: 2 in, 2 out]
                        n743 = TDMS Close(8:w1225, 11:w1224) -> (0:w1223:errorcluster)  [unwired: 1 out]
                      }
                      frame #1 {
                        n744 = local read "DISP LAB05-2"() -> (w1244:T4)
                        n745 = Bundle(cluster=w1244, "STATUS"="STOP") -> (w1242:T4)  [unwired: 2 in]
                        n746 = local write "RESULT LAB05-2"(FALSE) -> ()
                        n747 = local write "DISP LAB05-2"(w1242) -> ()
                        n748 = call "Save data file to network drive v1.vi"("panel id"="LAB05-2") -> ("network file save error"=w1239:errorcluster)  [unwired: 9 in, 1 out]
                        n749 = local write "data file error"(w1239) -> ()
                      }
                    }
                  }
                  frame True {
                    # "start new test and create test file"
                    n750 = stacked-sequence {
                      seq-local: [w1251 _ _ _ _] -> [_ w1276 _ _ _]
                      tunnel: w1250 -> [w1256 _ _ _ _]
                      tunnel: w1249 -> [w1252 _ _ _ _]
                      tunnel: w1248 -> [w1266 _ _ _ _]
                      tunnel: w1247 -> [w1259 _ _ _ _]
                      tunnel: w1246 -> [w1254 _ _ _ _]
                      tunnel: [_ w1270 _ _ _] -> w1245
                      frame #0 {
                        w1253 = "\\"
                        n751 = local read "SET LAB05-2"() -> (w1261:T5)
                        n752 = case shown="\"CHART TEST\", Default" w1266 {
                          tunnel: ["CHART TEST-" "CYCLE TEST-" "T-RISE TEST-"] -> w1262
                          frame "CHART TEST", Default {
                          }
                          frame "CYCLE TEST" {
                          }
                          frame "T-RISE TEST" {
                          }
                        }
                        n753 = Unbundle(w1261) -> ("DESCRIPTION"=w1260:string)  [unwired: 4 out]
                        n754 = Concatenate Strings(w1256, "LAB05-2\\", w1254, w1253, w1252, w1253) -> (w1263:string)
                        n755 = String To Path(string=w1263) -> (path=w1265:path)
                        n756 = Concatenate Strings(w1263, w1262, w1260, "-", w1259, ".tdms") -> (w1251:string)
                        n757 = Create Folder(path (use dialog)=w1265) -> (error out=w1264:errorcluster)  [unwired: 2 in, 2 out]
                        n758 = global write "Global 1.vi" "LAB05-2 FILE"(w1251) -> ()
                        n759 = call <vilib>:"Clear Errors.vi"("error in (no error)"=w1264) -> ()  [unwired: 6 in, 1 out]
                      }
                      frame #1 {
                        n760 = String To Path(string=w1276) -> (path=w1271:path)
                        n761 = TDMS Open(5:FALSE, 6:FALSE, 10:T15."create or replace" ("operation (0:open)"), 11:w1271) -> (0:w1270:errorcluster, 3:→"TDMS LAB05-2":refnum<k34>)  [unwired: 3 in]
                      }
                      frame #2 {
                        n762 = local read "SET LAB05-2"() -> (w1282:T5)
                        n763 = local read "TDMS LAB05-2"() -> (w1293:refnum<k34>)
                        n764 = Build Array("Testers Name", "Description", "Set Test Cycles", "T-Rise minutes", "T-Rise Deg C") -> (w1283:string[])
                        n765 = Unbundle(w1282) -> ("NAME"=w1281:string, "DESCRIPTION"=w1280:string, "CYCLES"=w1279:dbl, "T-RISE mins"=w1278:dbl, "T-RISE deg C"=w1277:dbl)
                        n766 = Number To Decimal String(number=w1279) -> (decimal integer string=w1292:string)  [unwired: 1 in]
                        n767 = Number To Decimal String(number=w1278) -> (decimal integer string=w1291:string)  [unwired: 1 in]
                        n768 = Number To Decimal String(number=w1277) -> (decimal integer string=w1290:string)  [unwired: 1 in]
                        n769 = Build Array(w1281, w1280, w1292, w1291, w1290) -> (w1289:string[])
                        n770 = TDMS Set Properties(5:w1289, 7:w1283, 11:w1293) -> ()  [unwired: 3 in, 4 out]
                      }
                      frame #3 {
                        w1295 = 0.0
                        n771 = local read "DISP LAB05-2"() -> (w1297:T4)
                        n772 = Bundle(cluster=w1297, "CYCLE"=w1295, "MINS"=w1295, "STATUS"="RUN") -> (w1296:T4)
                        n773 = local write "DISP LAB05-2"(w1296) -> ()
                      }
                      frame #4 {
                        n774 = local read "SIG LAB05-2"() -> (w1300:T2)
                        n775 = local read "TEMP START LAB05-2"() -> (w1302:cluster{"TL":dbl, "TN":dbl})
                        n776 = Unbundle(w1300) -> ("Tmp Live"=w1299:dbl, "Tmp Neut"=w1298:dbl)  [unwired: 3 out]
                        n777 = Bundle(cluster=w1302, "TL"=w1299, "TN"=w1298) -> (w1301:cluster{"TL":dbl, "TN":dbl})
                        n778 = local write "TEMP START LAB05-2"(w1301) -> ()
                      }
                    }
                  }
                }
              }
            }
            n779 = local write "data file error"(w384) -> ()
          }
          frame #4 {
            # "check if test cycles reached for cycle tests, if so then test pass"
            n780 = stacked-sequence {
              tunnel: w1322 -> [_ _ _ _ _ _ _ _ _ _]
              tunnel: w1321 -> [_ _ _ _ _ _ _ _ _ _]
              tunnel: w1320 -> [_ _ _ _ _ _ _ _ _ _]
              tunnel: w1319 -> [_ _ _ _ _ _ _ _ _ _]
              tunnel: w1318 -> [_ _ _ _ _ _ _ _ _ _]
              tunnel: w1317 -> [_ _ _ _ _ _ _ _ _ _]
              tunnel: w1316 -> [_ _ _ _ _ _ _ _ _ _]
              tunnel: w1315 -> [_ _ _ _ _ _ _ _ _ _]
              tunnel: w1314 -> [_ _ _ _ _ _ _ _ _ _]
              tunnel: w1313 -> [_ _ _ _ _ _ _ _ _ _]
              tunnel: w1312 -> [w1327 _ _ _ _ _ _ _ _ _]
              tunnel: w1311 -> [_ w1362 _ _ _ _ _ _ _ _]
              tunnel: w1310 -> [_ _ w1401 _ _ _ _ _ _ _]
              tunnel: w1309 -> [_ _ _ w1440 _ _ _ _ _ _]
              tunnel: w1308 -> [_ _ _ _ w1479 _ _ _ _ _]
              tunnel: w1307 -> [_ _ _ _ _ w1518 _ _ _ _]
              tunnel: w1306 -> [_ _ _ _ _ _ w1557 _ _ _]
              tunnel: w1305 -> [_ _ _ _ _ _ _ w1596 _ _]
              tunnel: w1304 -> [_ _ _ _ _ _ _ _ w1635 _]
              tunnel: w1303 -> [_ _ _ _ _ _ _ _ _ w1674]
              frame #0 {
                # "LAB01-1"
                n781 = Less?(x=w1327, y=2) -> (x < y?=w1325:bool)
                n782 = local read "DISP LAB01-1"() -> (w1328:T4)
                n783 = Unbundle(w1328) -> ("STATUS"=w1329:string)  [unwired: 2 out]
                n784 = Equal?(x=w1329, y="RUN") -> (x = y?=w1324:bool)
                n785 = And(x=w1324, y=w1325) -> (x .and. y?=w1323:bool)
                n786 = case shown="True" w1323 {
                  tunnel: w1328 -> [_ w1332]
                  tunnel: w1327 -> [_ w1337]
                  frame False {
                  }
                  frame True {
                    n787 = local read "SET LAB01-1"() -> (w1339:T5)
                    n788 = local read "TDMS LAB01-1"() -> (w1331:refnum<k34>)
                    n789 = Unbundle(w1332) -> ("CYCLE"=w1338:dbl)  [unwired: 2 out]
                    n790 = Unbundle(w1339) -> ("CYCLES"=w1334:dbl, "T-RISE mins"=w1336:dbl)  [unwired: 3 out]
                    n791 = case shown="\"CHART TEST\", Default" w1337 {
                      tunnel: w1336 -> [_ _ w1346]
                      tunnel: [w1341 w1343 w1346] -> w1335
                      tunnel: w1334 -> [w1341 w1343 _]
                      tunnel: ["CHART TEST" "CYCLES" "T-RISE TEST"] -> w1333
                      frame "CHART TEST", Default {
                      }
                      frame "CYCLE TEST" {
                      }
                      frame "T-RISE TEST" {
                      }
                    }
                    n792 = Greater Or Equal?(x=w1338, y=w1334) -> (x >= y?=w1340:bool)
                    n793 = case shown="True" w1340 {
                      tunnel: w1335 -> [w1350 _]
                      tunnel: w1333 -> [w1349 _]
                      tunnel: w1332 -> [w1348 _]
                      tunnel: w1331 -> [w1347 _]
                      frame True {
                        n794 = stacked-sequence {
                          tunnel: w1350 -> [w1354 _]
                          tunnel: w1349 -> [w1352 _]
                          tunnel: w1348 -> [_ w1360]
                          tunnel: w1347 -> [w1351 _]
                          frame #0 {
                            n795 = Build Array(w1352) -> (w1355:string[])
                            n796 = Build Array(w1354) -> (w1353:dbl[])
                            n797 = TDMS Write(0:w1351, 5:"TEST PASS", 7:w1355, 9:w1353) -> (15:w1357:errorcluster)  [unwired: 2 in, 3 out]
                            n798 = local write "data file error"(w1357) -> ()
                          }
                          frame #1 {
                            n799 = Bundle(cluster=w1360, "STATUS"="CYCLE PASS") -> (w1358:T4)  [unwired: 2 in]
                            n800 = local write "RESULT LAB01-1"(TRUE) -> ()
                            n801 = local write "DISP LAB01-1"(w1358) -> ()
                          }
                        }
                      }
                      frame False {
                      }
                    }
                  }
                }
              }
              frame #1 {
                # "LAB01-2"
                n802 = Less?(x=w1362, y=2) -> (x < y?=w1365:bool)
                n803 = local read "DISP LAB01-2"() -> (w1367:T4)
                n804 = Unbundle(w1367) -> ("STATUS"=w1368:string)  [unwired: 2 out]
                n805 = Equal?(x=w1368, y="RUN") -> (x = y?=w1364:bool)
                n806 = And(x=w1364, y=w1365) -> (x .and. y?=w1363:bool)
                n807 = case shown="True" w1363 {
                  tunnel: w1367 -> [_ w1371]
                  tunnel: w1362 -> [_ w1376]
                  frame False {
                  }
                  frame True {
                    n808 = local read "SET LAB01-2"() -> (w1378:T5)
                    n809 = local read "TDMS LAB01-2"() -> (w1370:refnum<k34>)
                    n810 = Unbundle(w1371) -> ("CYCLE"=w1377:dbl)  [unwired: 2 out]
                    n811 = Unbundle(w1378) -> ("CYCLES"=w1373:dbl, "T-RISE mins"=w1375:dbl)  [unwired: 3 out]
                    n812 = case shown="\"CHART TEST\", Default" w1376 {
                      tunnel: w1375 -> [_ _ w1385]
                      tunnel: [w1380 w1382 w1385] -> w1374
                      tunnel: w1373 -> [w1380 w1382 _]
                      tunnel: ["CHART TEST " "CYCLES" "T-RISE TEST"] -> w1372
                      frame "CHART TEST", Default {
                      }
                      frame "CYCLE TEST" {
                      }
                      frame "T-RISE TEST" {
                      }
                    }
                    n813 = Greater Or Equal?(x=w1377, y=w1373) -> (x >= y?=w1379:bool)
                    n814 = case shown="True" w1379 {
                      tunnel: w1374 -> [w1389 _]
                      tunnel: w1372 -> [w1388 _]
                      tunnel: w1371 -> [w1387 _]
                      tunnel: w1370 -> [w1386 _]
                      frame True {
                        n815 = stacked-sequence {
                          tunnel: w1389 -> [w1393 _]
                          tunnel: w1388 -> [w1391 _]
                          tunnel: w1387 -> [_ w1399]
                          tunnel: w1386 -> [w1390 _]
                          frame #0 {
                            n816 = Build Array(w1391) -> (w1394:string[])
                            n817 = Build Array(w1393) -> (w1392:dbl[])
                            n818 = TDMS Write(0:w1390, 5:"TEST PASS", 7:w1394, 9:w1392) -> (15:w1396:errorcluster)  [unwired: 2 in, 3 out]
                            n819 = local write "data file error"(w1396) -> ()
                          }
                          frame #1 {
                            n820 = Bundle(cluster=w1399, "STATUS"="CYCLE PASS") -> (w1397:T4)  [unwired: 2 in]
                            n821 = local write "RESULT LAB01-2"(TRUE) -> ()
                            n822 = local write "DISP LAB01-2"(w1397) -> ()
                          }
                        }
                      }
                      frame False {
                      }
                    }
                  }
                }
              }
              frame #2 {
                # "LAB02-1"
                n823 = Less?(x=w1401, y=2) -> (x < y?=w1404:bool)
                n824 = local read "DISP LAB02-1"() -> (w1406:T4)
                n825 = Unbundle(w1406) -> ("STATUS"=w1407:string)  [unwired: 2 out]
                n826 = Equal?(x=w1407, y="RUN") -> (x = y?=w1403:bool)
                n827 = And(x=w1403, y=w1404) -> (x .and. y?=w1402:bool)
                n828 = case shown="True" w1402 {
                  tunnel: w1406 -> [_ w1410]
                  tunnel: w1401 -> [_ w1415]
                  frame False {
                  }
                  frame True {
                    n829 = local read "SET LAB02-1"() -> (w1417:T5)
                    n830 = local read "TDMS LAB02-1"() -> (w1409:refnum<k34>)
                    n831 = Unbundle(w1410) -> ("CYCLE"=w1416:dbl)  [unwired: 2 out]
                    n832 = Unbundle(w1417) -> ("CYCLES"=w1412:dbl, "T-RISE mins"=w1414:dbl)  [unwired: 3 out]
                    n833 = case shown="\"CHART TEST\", Default" w1415 {
                      tunnel: w1414 -> [_ _ w1424]
                      tunnel: [w1419 w1421 w1424] -> w1413
                      tunnel: w1412 -> [w1419 w1421 _]
                      tunnel: ["CHART TEST" "CYCLES" "T-RISE TEST"] -> w1411
                      frame "CHART TEST", Default {
                      }
                      frame "CYCLE TEST" {
                      }
                      frame "T-RISE TEST" {
                      }
                    }
                    n834 = Greater Or Equal?(x=w1416, y=w1412) -> (x >= y?=w1418:bool)
                    n835 = case shown="True" w1418 {
                      tunnel: w1413 -> [w1428 _]
                      tunnel: w1411 -> [w1427 _]
                      tunnel: w1410 -> [w1426 _]
                      tunnel: w1409 -> [w1425 _]
                      frame True {
                        n836 = stacked-sequence {
                          tunnel: w1428 -> [w1432 _]
                          tunnel: w1427 -> [w1430 _]
                          tunnel: w1426 -> [_ w1438]
                          tunnel: w1425 -> [w1429 _]
                          frame #0 {
                            n837 = Build Array(w1430) -> (w1433:string[])
                            n838 = Build Array(w1432) -> (w1431:dbl[])
                            n839 = TDMS Write(0:w1429, 5:"TEST PASS", 7:w1433, 9:w1431) -> (15:w1435:errorcluster)  [unwired: 2 in, 3 out]
                            n840 = local write "data file error"(w1435) -> ()
                          }
                          frame #1 {
                            n841 = Bundle(cluster=w1438, "STATUS"="CYCLE PASS") -> (w1436:T4)  [unwired: 2 in]
                            n842 = local write "RESULT LAB02-1"(TRUE) -> ()
                            n843 = local write "DISP LAB02-1"(w1436) -> ()
                          }
                        }
                      }
                      frame False {
                      }
                    }
                  }
                }
              }
              frame #3 {
                # "LAB02-2"
                n844 = Less?(x=w1440, y=2) -> (x < y?=w1443:bool)
                n845 = local read "DISP LAB02-2"() -> (w1445:T4)
                n846 = Unbundle(w1445) -> ("STATUS"=w1446:string)  [unwired: 2 out]
                n847 = Equal?(x=w1446, y="RUN") -> (x = y?=w1442:bool)
                n848 = And(x=w1442, y=w1443) -> (x .and. y?=w1441:bool)
                n849 = case shown="True" w1441 {
                  tunnel: w1445 -> [_ w1449]
                  tunnel: w1440 -> [_ w1454]
                  frame False {
                  }
                  frame True {
                    n850 = local read "SET LAB02-2"() -> (w1456:T5)
                    n851 = local read "TDMS LAB02-2"() -> (w1448:refnum<k34>)
                    n852 = Unbundle(w1449) -> ("CYCLE"=w1455:dbl)  [unwired: 2 out]
                    n853 = Unbundle(w1456) -> ("CYCLES"=w1451:dbl, "T-RISE mins"=w1453:dbl)  [unwired: 3 out]
                    n854 = case shown="\"CHART TEST\", Default" w1454 {
                      tunnel: w1453 -> [_ _ w1463]
                      tunnel: [w1458 w1460 w1463] -> w1452
                      tunnel: w1451 -> [w1458 w1460 _]
                      tunnel: ["CHART TEST" "CYCLES" "T-RISE TEST"] -> w1450
                      frame "CHART TEST", Default {
                      }
                      frame "CYCLE TEST" {
                      }
                      frame "T-RISE TEST" {
                      }
                    }
                    n855 = Greater Or Equal?(x=w1455, y=w1451) -> (x >= y?=w1457:bool)
                    n856 = case shown="True" w1457 {
                      tunnel: w1452 -> [w1467 _]
                      tunnel: w1450 -> [w1466 _]
                      tunnel: w1449 -> [w1465 _]
                      tunnel: w1448 -> [w1464 _]
                      frame True {
                        n857 = stacked-sequence {
                          tunnel: w1467 -> [w1471 _]
                          tunnel: w1466 -> [w1469 _]
                          tunnel: w1465 -> [_ w1477]
                          tunnel: w1464 -> [w1468 _]
                          frame #0 {
                            n858 = Build Array(w1469) -> (w1472:string[])
                            n859 = Build Array(w1471) -> (w1470:dbl[])
                            n860 = TDMS Write(0:w1468, 5:"TEST PASS", 7:w1472, 9:w1470) -> (15:w1474:errorcluster)  [unwired: 2 in, 3 out]
                            n861 = local write "data file error"(w1474) -> ()
                          }
                          frame #1 {
                            n862 = Bundle(cluster=w1477, "STATUS"="CYCLE PASS") -> (w1475:T4)  [unwired: 2 in]
                            n863 = local write "RESULT LAB02-2"(TRUE) -> ()
                            n864 = local write "DISP LAB02-2"(w1475) -> ()
                          }
                        }
                      }
                      frame False {
                      }
                    }
                  }
                }
              }
              frame #4 {
                # "LAB03-1"
                n865 = Less?(x=w1479, y=2) -> (x < y?=w1482:bool)
                n866 = local read "DISP LAB03-1"() -> (w1484:T4)
                n867 = Unbundle(w1484) -> ("STATUS"=w1485:string)  [unwired: 2 out]
                n868 = Equal?(x=w1485, y="RUN") -> (x = y?=w1481:bool)
                n869 = And(x=w1481, y=w1482) -> (x .and. y?=w1480:bool)
                n870 = case shown="True" w1480 {
                  tunnel: w1484 -> [_ w1488]
                  tunnel: w1479 -> [_ w1493]
                  frame False {
                  }
                  frame True {
                    n871 = local read "SET LAB03-1"() -> (w1495:T5)
                    n872 = local read "TDMS LAB03-1"() -> (w1487:refnum<k34>)
                    n873 = Unbundle(w1488) -> ("CYCLE"=w1494:dbl)  [unwired: 2 out]
                    n874 = Unbundle(w1495) -> ("CYCLES"=w1490:dbl, "T-RISE mins"=w1492:dbl)  [unwired: 3 out]
                    n875 = case shown="\"CHART TEST\", Default" w1493 {
                      tunnel: w1492 -> [_ _ w1502]
                      tunnel: [w1497 w1499 w1502] -> w1491
                      tunnel: w1490 -> [w1497 w1499 _]
                      tunnel: ["CHART TEST" "CYCLES" "T-RISE TEST"] -> w1489
                      frame "CHART TEST", Default {
                      }
                      frame "CYCLE TEST" {
                      }
                      frame "T-RISE TEST" {
                      }
                    }
                    n876 = Greater Or Equal?(x=w1494, y=w1490) -> (x >= y?=w1496:bool)
                    n877 = case shown="True" w1496 {
                      tunnel: w1491 -> [w1506 _]
                      tunnel: w1489 -> [w1505 _]
                      tunnel: w1488 -> [w1504 _]
                      tunnel: w1487 -> [w1503 _]
                      frame True {
                        n878 = stacked-sequence {
                          tunnel: w1506 -> [w1510 _]
                          tunnel: w1505 -> [w1508 _]
                          tunnel: w1504 -> [_ w1516]
                          tunnel: w1503 -> [w1507 _]
                          frame #0 {
                            n879 = Build Array(w1508) -> (w1511:string[])
                            n880 = Build Array(w1510) -> (w1509:dbl[])
                            n881 = TDMS Write(0:w1507, 5:"TEST PASS", 7:w1511, 9:w1509) -> (15:w1513:errorcluster)  [unwired: 2 in, 3 out]
                            n882 = local write "data file error"(w1513) -> ()
                          }
                          frame #1 {
                            n883 = Bundle(cluster=w1516, "STATUS"="CYCLE PASS") -> (w1514:T4)  [unwired: 2 in]
                            n884 = local write "RESULT LAB03-1"(TRUE) -> ()
                            n885 = local write "DISP LAB03-1"(w1514) -> ()
                          }
                        }
                      }
                      frame False {
                      }
                    }
                  }
                }
              }
              frame #5 {
                # "LAB03-2"
                n886 = Less?(x=w1518, y=2) -> (x < y?=w1521:bool)
                n887 = local read "DISP LAB03-2"() -> (w1523:T4)
                n888 = Unbundle(w1523) -> ("STATUS"=w1524:string)  [unwired: 2 out]
                n889 = Equal?(x=w1524, y="RUN") -> (x = y?=w1520:bool)
                n890 = And(x=w1520, y=w1521) -> (x .and. y?=w1519:bool)
                n891 = case shown="True" w1519 {
                  tunnel: w1523 -> [_ w1527]
                  tunnel: w1518 -> [_ w1532]
                  frame False {
                  }
                  frame True {
                    n892 = local read "SET LAB03-2"() -> (w1534:T5)
                    n893 = local read "TDMS LAB03-2"() -> (w1526:refnum<k34>)
                    n894 = Unbundle(w1527) -> ("CYCLE"=w1533:dbl)  [unwired: 2 out]
                    n895 = Unbundle(w1534) -> ("CYCLES"=w1529:dbl, "T-RISE mins"=w1531:dbl)  [unwired: 3 out]
                    n896 = case shown="\"CHART TEST\", Default" w1532 {
                      tunnel: w1531 -> [_ _ w1541]
                      tunnel: [w1536 w1538 w1541] -> w1530
                      tunnel: w1529 -> [w1536 w1538 _]
                      tunnel: ["CHART TEST" "CYCLES" "T-RISE TEST"] -> w1528
                      frame "CHART TEST", Default {
                      }
                      frame "CYCLE TEST" {
                      }
                      frame "T-RISE TEST" {
                      }
                    }
                    n897 = Greater Or Equal?(x=w1533, y=w1529) -> (x >= y?=w1535:bool)
                    n898 = case shown="True" w1535 {
                      tunnel: w1530 -> [w1545 _]
                      tunnel: w1528 -> [w1544 _]
                      tunnel: w1527 -> [w1543 _]
                      tunnel: w1526 -> [w1542 _]
                      frame True {
                        n899 = stacked-sequence {
                          tunnel: w1545 -> [w1549 _]
                          tunnel: w1544 -> [w1547 _]
                          tunnel: w1543 -> [_ w1555]
                          tunnel: w1542 -> [w1546 _]
                          frame #0 {
                            n900 = Build Array(w1547) -> (w1550:string[])
                            n901 = Build Array(w1549) -> (w1548:dbl[])
                            n902 = TDMS Write(0:w1546, 5:"TEST PASS", 7:w1550, 9:w1548) -> (15:w1552:errorcluster)  [unwired: 2 in, 3 out]
                            n903 = local write "data file error"(w1552) -> ()
                          }
                          frame #1 {
                            n904 = Bundle(cluster=w1555, "STATUS"="CYCLE PASS") -> (w1553:T4)  [unwired: 2 in]
                            n905 = local write "RESULT LAB03-2"(TRUE) -> ()
                            n906 = local write "DISP LAB03-2"(w1553) -> ()
                          }
                        }
                      }
                      frame False {
                      }
                    }
                  }
                }
              }
              frame #6 {
                # "LAB04-1"
                n907 = Less?(x=w1557, y=2) -> (x < y?=w1560:bool)
                n908 = local read "DISP LAB04-1"() -> (w1562:T4)
                n909 = Unbundle(w1562) -> ("STATUS"=w1563:string)  [unwired: 2 out]
                n910 = Equal?(x=w1563, y="RUN") -> (x = y?=w1559:bool)
                n911 = And(x=w1559, y=w1560) -> (x .and. y?=w1558:bool)
                n912 = case shown="True" w1558 {
                  tunnel: w1562 -> [_ w1566]
                  tunnel: w1557 -> [_ w1571]
                  frame False {
                  }
                  frame True {
                    n913 = local read "SET LAB04-1"() -> (w1573:T5)
                    n914 = local read "TDMS LAB04-1"() -> (w1565:refnum<k34>)
                    n915 = Unbundle(w1566) -> ("CYCLE"=w1572:dbl)  [unwired: 2 out]
                    n916 = Unbundle(w1573) -> ("CYCLES"=w1568:dbl, "T-RISE mins"=w1570:dbl)  [unwired: 3 out]
                    n917 = case shown="\"CHART TEST\", Default" w1571 {
                      tunnel: w1570 -> [_ _ w1580]
                      tunnel: [w1575 w1577 w1580] -> w1569
                      tunnel: w1568 -> [w1575 w1577 _]
                      tunnel: ["CHART TEST" "CYCLES" "T-RISE TEST"] -> w1567
                      frame "CHART TEST", Default {
                      }
                      frame "CYCLE TEST" {
                      }
                      frame "T-RISE TEST" {
                      }
                    }
                    n918 = Greater Or Equal?(x=w1572, y=w1568) -> (x >= y?=w1574:bool)
                    n919 = case shown="True" w1574 {
                      tunnel: w1569 -> [w1584 _]
                      tunnel: w1567 -> [w1583 _]
                      tunnel: w1566 -> [w1582 _]
                      tunnel: w1565 -> [w1581 _]
                      frame True {
                        n920 = stacked-sequence {
                          tunnel: w1584 -> [w1588 _]
                          tunnel: w1583 -> [w1586 _]
                          tunnel: w1582 -> [_ w1594]
                          tunnel: w1581 -> [w1585 _]
                          frame #0 {
                            n921 = Build Array(w1586) -> (w1589:string[])
                            n922 = Build Array(w1588) -> (w1587:dbl[])
                            n923 = TDMS Write(0:w1585, 5:"TEST PASS", 7:w1589, 9:w1587) -> (15:w1591:errorcluster)  [unwired: 2 in, 3 out]
                            n924 = local write "data file error"(w1591) -> ()
                          }
                          frame #1 {
                            n925 = Bundle(cluster=w1594, "STATUS"="CYCLE PASS") -> (w1592:T4)  [unwired: 2 in]
                            n926 = local write "RESULT LAB04-1"(TRUE) -> ()
                            n927 = local write "DISP LAB04-1"(w1592) -> ()
                          }
                        }
                      }
                      frame False {
                      }
                    }
                  }
                }
              }
              frame #7 {
                # "LAB04-2"
                n928 = Less?(x=w1596, y=2) -> (x < y?=w1599:bool)
                n929 = local read "DISP LAB04-2"() -> (w1601:T4)
                n930 = Unbundle(w1601) -> ("STATUS"=w1602:string)  [unwired: 2 out]
                n931 = Equal?(x=w1602, y="RUN") -> (x = y?=w1598:bool)
                n932 = And(x=w1598, y=w1599) -> (x .and. y?=w1597:bool)
                n933 = case shown="True" w1597 {
                  tunnel: w1601 -> [_ w1605]
                  tunnel: w1596 -> [_ w1610]
                  frame False {
                  }
                  frame True {
                    n934 = local read "SET LAB04-2"() -> (w1612:T5)
                    n935 = local read "TDMS LAB04-2"() -> (w1604:refnum<k34>)
                    n936 = Unbundle(w1605) -> ("CYCLE"=w1611:dbl)  [unwired: 2 out]
                    n937 = Unbundle(w1612) -> ("CYCLES"=w1607:dbl, "T-RISE mins"=w1609:dbl)  [unwired: 3 out]
                    n938 = case shown="\"CHART TEST\", Default" w1610 {
                      tunnel: w1609 -> [_ _ w1619]
                      tunnel: [w1614 w1616 w1619] -> w1608
                      tunnel: w1607 -> [w1614 w1616 _]
                      tunnel: ["CHART TEST" "CYCLES" "T-RISE TEST"] -> w1606
                      frame "CHART TEST", Default {
                      }
                      frame "CYCLE TEST" {
                      }
                      frame "T-RISE TEST" {
                      }
                    }
                    n939 = Greater Or Equal?(x=w1611, y=w1607) -> (x >= y?=w1613:bool)
                    n940 = case shown="True" w1613 {
                      tunnel: w1608 -> [w1623 _]
                      tunnel: w1606 -> [w1622 _]
                      tunnel: w1605 -> [w1621 _]
                      tunnel: w1604 -> [w1620 _]
                      frame True {
                        n941 = stacked-sequence {
                          tunnel: w1623 -> [w1627 _]
                          tunnel: w1622 -> [w1625 _]
                          tunnel: w1621 -> [_ w1633]
                          tunnel: w1620 -> [w1624 _]
                          frame #0 {
                            n942 = Build Array(w1625) -> (w1628:string[])
                            n943 = Build Array(w1627) -> (w1626:dbl[])
                            n944 = TDMS Write(0:w1624, 5:"TEST PASS", 7:w1628, 9:w1626) -> (15:w1630:errorcluster)  [unwired: 2 in, 3 out]
                            n945 = local write "data file error"(w1630) -> ()
                          }
                          frame #1 {
                            n946 = Bundle(cluster=w1633, "STATUS"="CYCLE PASS") -> (w1631:T4)  [unwired: 2 in]
                            n947 = local write "RESULT LAB04-2"(TRUE) -> ()
                            n948 = local write "DISP LAB04-2"(w1631) -> ()
                          }
                        }
                      }
                      frame False {
                      }
                    }
                  }
                }
              }
              frame #8 {
                # "LAB05-1"
                n949 = Less?(x=w1635, y=2) -> (x < y?=w1638:bool)
                n950 = local read "DISP LAB05-1"() -> (w1640:T4)
                n951 = Unbundle(w1640) -> ("STATUS"=w1641:string)  [unwired: 2 out]
                n952 = Equal?(x=w1641, y="RUN") -> (x = y?=w1637:bool)
                n953 = And(x=w1637, y=w1638) -> (x .and. y?=w1636:bool)
                n954 = case shown="True" w1636 {
                  tunnel: w1640 -> [_ w1644]
                  tunnel: w1635 -> [_ w1649]
                  frame False {
                  }
                  frame True {
                    n955 = local read "SET LAB05-1"() -> (w1651:T5)
                    n956 = local read "TDMS LAB05-1"() -> (w1643:refnum<k34>)
                    n957 = Unbundle(w1644) -> ("CYCLE"=w1650:dbl)  [unwired: 2 out]
                    n958 = Unbundle(w1651) -> ("CYCLES"=w1646:dbl, "T-RISE mins"=w1648:dbl)  [unwired: 3 out]
                    n959 = case shown="\"CHART TEST\", Default" w1649 {
                      tunnel: w1648 -> [_ _ w1658]
                      tunnel: [w1653 w1655 w1658] -> w1647
                      tunnel: w1646 -> [w1653 w1655 _]
                      tunnel: ["CHART TEST" "CYCLES" "T-RISE TEST"] -> w1645
                      frame "CHART TEST", Default {
                      }
                      frame "CYCLE TEST" {
                      }
                      frame "T-RISE TEST" {
                      }
                    }
                    n960 = Greater Or Equal?(x=w1650, y=w1646) -> (x >= y?=w1652:bool)
                    n961 = case shown="True" w1652 {
                      tunnel: w1647 -> [w1662 _]
                      tunnel: w1645 -> [w1661 _]
                      tunnel: w1644 -> [w1660 _]
                      tunnel: w1643 -> [w1659 _]
                      frame True {
                        n962 = stacked-sequence {
                          tunnel: w1662 -> [w1666 _]
                          tunnel: w1661 -> [w1664 _]
                          tunnel: w1660 -> [_ w1672]
                          tunnel: w1659 -> [w1663 _]
                          frame #0 {
                            n963 = Build Array(w1664) -> (w1667:string[])
                            n964 = Build Array(w1666) -> (w1665:dbl[])
                            n965 = TDMS Write(0:w1663, 5:"TEST PASS", 7:w1667, 9:w1665) -> (15:w1669:errorcluster)  [unwired: 2 in, 3 out]
                            n966 = local write "data file error"(w1669) -> ()
                          }
                          frame #1 {
                            n967 = Bundle(cluster=w1672, "STATUS"="CYCLE PASS") -> (w1670:T4)  [unwired: 2 in]
                            n968 = local write "RESULT LAB05-1"(TRUE) -> ()
                            n969 = local write "DISP LAB05-1"(w1670) -> ()
                          }
                        }
                      }
                      frame False {
                      }
                    }
                  }
                }
              }
              frame #9 {
                # "LAB05-2"
                n970 = Less?(x=w1674, y=2) -> (x < y?=w1677:bool)
                n971 = local read "DISP LAB05-2"() -> (w1679:T4)
                n972 = Unbundle(w1679) -> ("STATUS"=w1680:string)  [unwired: 2 out]
                n973 = Equal?(x=w1680, y="RUN") -> (x = y?=w1676:bool)
                n974 = And(x=w1676, y=w1677) -> (x .and. y?=w1675:bool)
                n975 = case shown="True" w1675 {
                  tunnel: w1679 -> [_ w1683]
                  tunnel: w1674 -> [_ w1688]
                  frame False {
                  }
                  frame True {
                    n976 = local read "SET LAB05-2"() -> (w1690:T5)
                    n977 = local read "TDMS LAB05-2"() -> (w1682:refnum<k34>)
                    n978 = Unbundle(w1683) -> ("CYCLE"=w1689:dbl)  [unwired: 2 out]
                    n979 = Unbundle(w1690) -> ("CYCLES"=w1685:dbl, "T-RISE mins"=w1687:dbl)  [unwired: 3 out]
                    n980 = case shown="\"CHART TEST\", Default" w1688 {
                      tunnel: w1687 -> [_ _ w1697]
                      tunnel: [w1692 w1694 w1697] -> w1686
                      tunnel: w1685 -> [w1692 w1694 _]
                      tunnel: ["CHART TEST" "CYCLES" "T-RISE TEST"] -> w1684
                      frame "CHART TEST", Default {
                      }
                      frame "CYCLE TEST" {
                      }
                      frame "T-RISE TEST" {
                      }
                    }
                    n981 = Greater Or Equal?(x=w1689, y=w1685) -> (x >= y?=w1691:bool)
                    n982 = case shown="True" w1691 {
                      tunnel: w1686 -> [w1701 _]
                      tunnel: w1684 -> [w1700 _]
                      tunnel: w1683 -> [w1699 _]
                      tunnel: w1682 -> [w1698 _]
                      frame True {
                        n983 = stacked-sequence {
                          tunnel: w1701 -> [w1705 _]
                          tunnel: w1700 -> [w1703 _]
                          tunnel: w1699 -> [_ w1711]
                          tunnel: w1698 -> [w1702 _]
                          frame #0 {
                            n984 = Build Array(w1703) -> (w1706:string[])
                            n985 = Build Array(w1705) -> (w1704:dbl[])
                            n986 = TDMS Write(0:w1702, 5:"TEST PASS", 7:w1706, 9:w1704) -> (15:w1708:errorcluster)  [unwired: 2 in, 3 out]
                            n987 = local write "data file error"(w1708) -> ()
                          }
                          frame #1 {
                            n988 = Bundle(cluster=w1711, "STATUS"="CYCLE PASS") -> (w1709:T4)  [unwired: 2 in]
                            n989 = local write "RESULT LAB05-2"(TRUE) -> ()
                            n990 = local write "DISP LAB05-2"(w1709) -> ()
                          }
                        }
                      }
                      frame False {
                      }
                    }
                  }
                }
              }
            }
          }
          frame #5 {
            # "check if test cycles reached for temperature rise test"
            n991 = stacked-sequence {
              tunnel: w1742 -> [_ _ _ _ _ _ _ _ _ _]
              tunnel: w1741 -> [_ _ _ _ _ _ _ _ _ _]
              tunnel: w1740 -> [_ _ _ _ _ _ _ _ _ _]
              tunnel: w1739 -> [_ _ _ _ _ _ _ _ _ _]
              tunnel: w1738 -> [_ _ _ _ _ _ _ _ _ _]
              tunnel: w1737 -> [_ _ _ _ _ _ _ _ _ _]
              tunnel: w1736 -> [_ _ _ _ _ _ _ _ _ _]
              tunnel: w1735 -> [_ _ _ _ _ _ _ _ _ _]
              tunnel: w1734 -> [_ _ _ _ _ _ _ _ _ _]
              tunnel: w1733 -> [_ _ _ _ _ _ _ _ _ _]
              tunnel: w1732 -> [w1748 _ _ _ _ _ _ _ _ _]
              tunnel: w1722 -> [w1743 _ _ _ _ _ _ _ _ _]
              tunnel: w1731 -> [_ w1774 _ _ _ _ _ _ _ _]
              tunnel: w1730 -> [_ _ w1804 _ _ _ _ _ _ _]
              tunnel: w1729 -> [_ _ _ w1834 _ _ _ _ _ _]
              tunnel: w1728 -> [_ _ _ _ w1864 _ _ _ _ _]
              tunnel: w1727 -> [_ _ _ _ _ w1894 _ _ _ _]
              tunnel: w1726 -> [_ _ _ _ _ _ w1924 _ _ _]
              tunnel: w1725 -> [_ _ _ _ _ _ _ w1954 _ _]
              tunnel: w1724 -> [_ _ _ _ _ _ _ _ w1984 _]
              tunnel: w1723 -> [_ _ _ _ _ _ _ _ _ w2014]
              tunnel: w1721 -> [_ w1773 _ _ _ _ _ _ _ _]
              tunnel: w1720 -> [_ _ w1803 _ _ _ _ _ _ _]
              tunnel: w1719 -> [_ _ _ w1833 _ _ _ _ _ _]
              tunnel: w1718 -> [_ _ _ _ w1863 _ _ _ _ _]
              tunnel: w1717 -> [_ _ _ _ _ w1893 _ _ _ _]
              tunnel: w1716 -> [_ _ _ _ _ _ w1923 _ _ _]
              tunnel: w1715 -> [_ _ _ _ _ _ _ w1953 _ _]
              tunnel: w1714 -> [_ _ _ _ _ _ _ _ w1983 _]
              tunnel: w1713 -> [_ _ _ _ _ _ _ _ _ w2013]
              frame #0 {
                # "LAB01-1"
                n992 = Equal?(x=w1748, y=2) -> (x = y?=w1746:bool)
                n993 = local read "DISP LAB01-1"() -> (w1749:T4)
                n994 = Unbundle(w1749) -> ("STATUS"=w1750:string)  [unwired: 2 out]
                n995 = Equal?(x=w1750, y="RUN") -> (x = y?=w1745:bool)
                n996 = And(x=w1745, y=w1746) -> (x .and. y?=w1744:bool)
                n997 = case shown="True" w1744 {
                  tunnel: w1749 -> [_ w1753]
                  tunnel: w1743 -> [_ w1756]
                  frame False {
                  }
                  frame True {
                    n998 = local read "SET LAB01-1"() -> (w1755:T5)
                    n999 = local read "TDMS LAB01-1"() -> (w1752:refnum<k34>)
                    n1000 = Unbundle(w1753) -> ("CYCLE"=w1757:dbl)  [unwired: 2 out]
                    n1001 = Unbundle(w1755) -> ("T-RISE mins"=w1754:dbl)  [unwired: 4 out]
                    n1002 = Greater Or Equal?(x=w1757, y=w1756) -> (x >= y?=w1758:bool)
                    n1003 = case shown="True" w1758 {
                      tunnel: w1754 -> [w1761 _]
                      tunnel: w1753 -> [w1760 _]
                      tunnel: w1752 -> [w1759 _]
                      frame True {
                        n1004 = stacked-sequence {
                          tunnel: w1761 -> [w1764 _]
                          tunnel: w1760 -> [_ w1769]
                          tunnel: w1759 -> [w1762 _]
                          frame #0 {
                            n1005 = Build Array("T-RISE") -> (w1766:string[])
                            n1006 = Build Array(w1764) -> (w1765:dbl[])
                            n1007 = TDMS Write(0:w1762, 5:"TEST PASS", 7:w1766, 9:w1765) -> (15:w1768:errorcluster)  [unwired: 2 in, 3 out]
                            n1008 = local write "data file error"(w1768) -> ()
                          }
                          frame #1 {
                            n1009 = Bundle(cluster=w1769, "STATUS"="T-RISE PASS") -> (w1771:T4)  [unwired: 2 in]
                            n1010 = local write "RESULT LAB01-1"(TRUE) -> ()
                            n1011 = local write "DISP LAB01-1"(w1771) -> ()
                          }
                        }
                      }
                      frame False {
                      }
                    }
                  }
                }
              }
              frame #1 {
                # "LAB01-2"
                n1012 = Equal?(x=w1774, y=2) -> (x = y?=w1777:bool)
                n1013 = local read "DISP LAB01-2"() -> (w1779:T4)
                n1014 = Unbundle(w1779) -> ("STATUS"=w1780:string)  [unwired: 2 out]
                n1015 = Equal?(x=w1780, y="RUN") -> (x = y?=w1776:bool)
                n1016 = And(x=w1776, y=w1777) -> (x .and. y?=w1775:bool)
                n1017 = case shown="True" w1775 {
                  tunnel: w1779 -> [_ w1783]
                  tunnel: w1773 -> [_ w1786]
                  frame False {
                  }
                  frame True {
                    n1018 = local read "SET LAB01-2"() -> (w1785:T5)
                    n1019 = local read "TDMS LAB01-2"() -> (w1782:refnum<k34>)
                    n1020 = Unbundle(w1783) -> ("CYCLE"=w1787:dbl)  [unwired: 2 out]
                    n1021 = Unbundle(w1785) -> ("T-RISE mins"=w1784:dbl)  [unwired: 4 out]
                    n1022 = Greater Or Equal?(x=w1787, y=w1786) -> (x >= y?=w1788:bool)
                    n1023 = case shown="True" w1788 {
                      tunnel: w1784 -> [w1791 _]
                      tunnel: w1783 -> [w1790 _]
                      tunnel: w1782 -> [w1789 _]
                      frame True {
                        n1024 = stacked-sequence {
                          tunnel: w1791 -> [w1794 _]
                          tunnel: w1790 -> [_ w1799]
                          tunnel: w1789 -> [w1792 _]
                          frame #0 {
                            n1025 = Build Array("T-RISE") -> (w1796:string[])
                            n1026 = Build Array(w1794) -> (w1795:dbl[])
                            n1027 = TDMS Write(0:w1792, 5:"TEST PASS", 7:w1796, 9:w1795) -> (15:w1798:errorcluster)  [unwired: 2 in, 3 out]
                            n1028 = local write "data file error"(w1798) -> ()
                          }
                          frame #1 {
                            n1029 = Bundle(cluster=w1799, "STATUS"="T-RISE PASS") -> (w1801:T4)  [unwired: 2 in]
                            n1030 = local write "RESULT LAB01-2"(TRUE) -> ()
                            n1031 = local write "DISP LAB01-2"(w1801) -> ()
                          }
                        }
                      }
                      frame False {
                      }
                    }
                  }
                }
              }
              frame #2 {
                # "LAB02-1"
                n1032 = Equal?(x=w1804, y=2) -> (x = y?=w1807:bool)
                n1033 = local read "DISP LAB02-1"() -> (w1809:T4)
                n1034 = Unbundle(w1809) -> ("STATUS"=w1810:string)  [unwired: 2 out]
                n1035 = Equal?(x=w1810, y="RUN") -> (x = y?=w1806:bool)
                n1036 = And(x=w1806, y=w1807) -> (x .and. y?=w1805:bool)
                n1037 = case shown="True" w1805 {
                  tunnel: w1809 -> [_ w1813]
                  tunnel: w1803 -> [_ w1816]
                  frame False {
                  }
                  frame True {
                    n1038 = local read "SET LAB02-1"() -> (w1815:T5)
                    n1039 = local read "TDMS LAB02-1"() -> (w1812:refnum<k34>)
                    n1040 = Unbundle(w1813) -> ("CYCLE"=w1817:dbl)  [unwired: 2 out]
                    n1041 = Unbundle(w1815) -> ("T-RISE mins"=w1814:dbl)  [unwired: 4 out]
                    n1042 = Greater Or Equal?(x=w1817, y=w1816) -> (x >= y?=w1818:bool)
                    n1043 = case shown="True" w1818 {
                      tunnel: w1814 -> [w1821 _]
                      tunnel: w1813 -> [w1820 _]
                      tunnel: w1812 -> [w1819 _]
                      frame True {
                        n1044 = stacked-sequence {
                          tunnel: w1821 -> [w1824 _]
                          tunnel: w1820 -> [_ w1829]
                          tunnel: w1819 -> [w1822 _]
                          frame #0 {
                            n1045 = Build Array("T-RISE") -> (w1826:string[])
                            n1046 = Build Array(w1824) -> (w1825:dbl[])
                            n1047 = TDMS Write(0:w1822, 5:"TEST PASS", 7:w1826, 9:w1825) -> (15:w1828:errorcluster)  [unwired: 2 in, 3 out]
                            n1048 = local write "data file error"(w1828) -> ()
                          }
                          frame #1 {
                            n1049 = Bundle(cluster=w1829, "STATUS"="T-RISE PASS") -> (w1831:T4)  [unwired: 2 in]
                            n1050 = local write "RESULT LAB02-1"(TRUE) -> ()
                            n1051 = local write "DISP LAB02-1"(w1831) -> ()
                          }
                        }
                      }
                      frame False {
                      }
                    }
                  }
                }
              }
              frame #3 {
                # "LAB02-2"
                n1052 = Equal?(x=w1834, y=2) -> (x = y?=w1837:bool)
                n1053 = local read "DISP LAB02-2"() -> (w1839:T4)
                n1054 = Unbundle(w1839) -> ("STATUS"=w1840:string)  [unwired: 2 out]
                n1055 = Equal?(x=w1840, y="RUN") -> (x = y?=w1836:bool)
                n1056 = And(x=w1836, y=w1837) -> (x .and. y?=w1835:bool)
                n1057 = case shown="True" w1835 {
                  tunnel: w1839 -> [_ w1843]
                  tunnel: w1833 -> [_ w1846]
                  frame False {
                  }
                  frame True {
                    n1058 = local read "SET LAB02-2"() -> (w1845:T5)
                    n1059 = local read "TDMS LAB02-2"() -> (w1842:refnum<k34>)
                    n1060 = Unbundle(w1843) -> ("CYCLE"=w1847:dbl)  [unwired: 2 out]
                    n1061 = Unbundle(w1845) -> ("T-RISE mins"=w1844:dbl)  [unwired: 4 out]
                    n1062 = Greater Or Equal?(x=w1847, y=w1846) -> (x >= y?=w1848:bool)
                    n1063 = case shown="True" w1848 {
                      tunnel: w1844 -> [w1851 _]
                      tunnel: w1843 -> [w1850 _]
                      tunnel: w1842 -> [w1849 _]
                      frame True {
                        n1064 = stacked-sequence {
                          tunnel: w1851 -> [w1854 _]
                          tunnel: w1850 -> [_ w1859]
                          tunnel: w1849 -> [w1852 _]
                          frame #0 {
                            n1065 = Build Array("T-RISE") -> (w1856:string[])
                            n1066 = Build Array(w1854) -> (w1855:dbl[])
                            n1067 = TDMS Write(0:w1852, 5:"TEST PASS", 7:w1856, 9:w1855) -> (15:w1858:errorcluster)  [unwired: 2 in, 3 out]
                            n1068 = local write "data file error"(w1858) -> ()
                          }
                          frame #1 {
                            n1069 = Bundle(cluster=w1859, "STATUS"="T-RISE PASS") -> (w1861:T4)  [unwired: 2 in]
                            n1070 = local write "RESULT LAB02-2"(TRUE) -> ()
                            n1071 = local write "DISP LAB02-2"(w1861) -> ()
                          }
                        }
                      }
                      frame False {
                      }
                    }
                  }
                }
              }
              frame #4 {
                # "LAB03-1"
                n1072 = Equal?(x=w1864, y=2) -> (x = y?=w1867:bool)
                n1073 = local read "DISP LAB03-1"() -> (w1869:T4)
                n1074 = Unbundle(w1869) -> ("STATUS"=w1870:string)  [unwired: 2 out]
                n1075 = Equal?(x=w1870, y="RUN") -> (x = y?=w1866:bool)
                n1076 = And(x=w1866, y=w1867) -> (x .and. y?=w1865:bool)
                n1077 = case shown="True" w1865 {
                  tunnel: w1869 -> [_ w1873]
                  tunnel: w1863 -> [_ w1876]
                  frame False {
                  }
                  frame True {
                    n1078 = local read "SET LAB03-1"() -> (w1875:T5)
                    n1079 = local read "TDMS LAB03-1"() -> (w1872:refnum<k34>)
                    n1080 = Unbundle(w1873) -> ("CYCLE"=w1877:dbl)  [unwired: 2 out]
                    n1081 = Unbundle(w1875) -> ("T-RISE mins"=w1874:dbl)  [unwired: 4 out]
                    n1082 = Greater Or Equal?(x=w1877, y=w1876) -> (x >= y?=w1878:bool)
                    n1083 = case shown="True" w1878 {
                      tunnel: w1874 -> [w1881 _]
                      tunnel: w1873 -> [w1880 _]
                      tunnel: w1872 -> [w1879 _]
                      frame True {
                        n1084 = stacked-sequence {
                          tunnel: w1881 -> [w1884 _]
                          tunnel: w1880 -> [_ w1889]
                          tunnel: w1879 -> [w1882 _]
                          frame #0 {
                            n1085 = Build Array("T-RISE") -> (w1886:string[])
                            n1086 = Build Array(w1884) -> (w1885:dbl[])
                            n1087 = TDMS Write(0:w1882, 5:"TEST PASS", 7:w1886, 9:w1885) -> (15:w1888:errorcluster)  [unwired: 2 in, 3 out]
                            n1088 = local write "data file error"(w1888) -> ()
                          }
                          frame #1 {
                            n1089 = Bundle(cluster=w1889, "STATUS"="T-RISE PASS") -> (w1891:T4)  [unwired: 2 in]
                            n1090 = local write "RESULT LAB03-1"(TRUE) -> ()
                            n1091 = local write "DISP LAB03-1"(w1891) -> ()
                          }
                        }
                      }
                      frame False {
                      }
                    }
                  }
                }
              }
              frame #5 {
                # "LAB03-2"
                n1092 = Equal?(x=w1894, y=2) -> (x = y?=w1897:bool)
                n1093 = local read "DISP LAB03-2"() -> (w1899:T4)
                n1094 = Unbundle(w1899) -> ("STATUS"=w1900:string)  [unwired: 2 out]
                n1095 = Equal?(x=w1900, y="RUN") -> (x = y?=w1896:bool)
                n1096 = And(x=w1896, y=w1897) -> (x .and. y?=w1895:bool)
                n1097 = case shown="True" w1895 {
                  tunnel: w1899 -> [_ w1903]
                  tunnel: w1893 -> [_ w1906]
                  frame False {
                  }
                  frame True {
                    n1098 = local read "SET LAB03-2"() -> (w1905:T5)
                    n1099 = local read "TDMS LAB03-2"() -> (w1902:refnum<k34>)
                    n1100 = Unbundle(w1903) -> ("CYCLE"=w1907:dbl)  [unwired: 2 out]
                    n1101 = Unbundle(w1905) -> ("T-RISE mins"=w1904:dbl)  [unwired: 4 out]
                    n1102 = Greater Or Equal?(x=w1907, y=w1906) -> (x >= y?=w1908:bool)
                    n1103 = case shown="True" w1908 {
                      tunnel: w1904 -> [w1911 _]
                      tunnel: w1903 -> [w1910 _]
                      tunnel: w1902 -> [w1909 _]
                      frame True {
                        n1104 = stacked-sequence {
                          tunnel: w1911 -> [w1914 _]
                          tunnel: w1910 -> [_ w1919]
                          tunnel: w1909 -> [w1912 _]
                          frame #0 {
                            n1105 = Build Array("T-RISE") -> (w1916:string[])
                            n1106 = Build Array(w1914) -> (w1915:dbl[])
                            n1107 = TDMS Write(0:w1912, 5:"TEST PASS", 7:w1916, 9:w1915) -> (15:w1918:errorcluster)  [unwired: 2 in, 3 out]
                            n1108 = local write "data file error"(w1918) -> ()
                          }
                          frame #1 {
                            n1109 = Bundle(cluster=w1919, "STATUS"="T-RISE PASS") -> (w1921:T4)  [unwired: 2 in]
                            n1110 = local write "RESULT LAB03-2"(TRUE) -> ()
                            n1111 = local write "DISP LAB03-2"(w1921) -> ()
                          }
                        }
                      }
                      frame False {
                      }
                    }
                  }
                }
              }
              frame #6 {
                # "LAB04-1"
                n1112 = Equal?(x=w1924, y=2) -> (x = y?=w1927:bool)
                n1113 = local read "DISP LAB04-1"() -> (w1929:T4)
                n1114 = Unbundle(w1929) -> ("STATUS"=w1930:string)  [unwired: 2 out]
                n1115 = Equal?(x=w1930, y="RUN") -> (x = y?=w1926:bool)
                n1116 = And(x=w1926, y=w1927) -> (x .and. y?=w1925:bool)
                n1117 = case shown="True" w1925 {
                  tunnel: w1929 -> [_ w1933]
                  tunnel: w1923 -> [_ w1936]
                  frame False {
                  }
                  frame True {
                    n1118 = local read "SET LAB04-1"() -> (w1935:T5)
                    n1119 = local read "TDMS LAB04-1"() -> (w1932:refnum<k34>)
                    n1120 = Unbundle(w1933) -> ("CYCLE"=w1937:dbl)  [unwired: 2 out]
                    n1121 = Unbundle(w1935) -> ("T-RISE mins"=w1934:dbl)  [unwired: 4 out]
                    n1122 = Greater Or Equal?(x=w1937, y=w1936) -> (x >= y?=w1938:bool)
                    n1123 = case shown="True" w1938 {
                      tunnel: w1934 -> [w1941 _]
                      tunnel: w1933 -> [w1940 _]
                      tunnel: w1932 -> [w1939 _]
                      frame True {
                        n1124 = stacked-sequence {
                          tunnel: w1941 -> [w1944 _]
                          tunnel: w1940 -> [_ w1949]
                          tunnel: w1939 -> [w1942 _]
                          frame #0 {
                            n1125 = Build Array("T-RISE") -> (w1946:string[])
                            n1126 = Build Array(w1944) -> (w1945:dbl[])
                            n1127 = TDMS Write(0:w1942, 5:"TEST PASS", 7:w1946, 9:w1945) -> (15:w1948:errorcluster)  [unwired: 2 in, 3 out]
                            n1128 = local write "data file error"(w1948) -> ()
                          }
                          frame #1 {
                            n1129 = Bundle(cluster=w1949, "STATUS"="T-RISE PASS") -> (w1951:T4)  [unwired: 2 in]
                            n1130 = local write "RESULT LAB04-1"(TRUE) -> ()
                            n1131 = local write "DISP LAB04-1"(w1951) -> ()
                          }
                        }
                      }
                      frame False {
                      }
                    }
                  }
                }
              }
              frame #7 {
                # "LAB04-2"
                n1132 = Equal?(x=w1954, y=2) -> (x = y?=w1957:bool)
                n1133 = local read "DISP LAB04-2"() -> (w1959:T4)
                n1134 = Unbundle(w1959) -> ("STATUS"=w1960:string)  [unwired: 2 out]
                n1135 = Equal?(x=w1960, y="RUN") -> (x = y?=w1956:bool)
                n1136 = And(x=w1956, y=w1957) -> (x .and. y?=w1955:bool)
                n1137 = case shown="True" w1955 {
                  tunnel: w1959 -> [_ w1963]
                  tunnel: w1953 -> [_ w1966]
                  frame False {
                  }
                  frame True {
                    n1138 = local read "SET LAB04-2"() -> (w1965:T5)
                    n1139 = local read "TDMS LAB04-2"() -> (w1962:refnum<k34>)
                    n1140 = Unbundle(w1963) -> ("CYCLE"=w1967:dbl)  [unwired: 2 out]
                    n1141 = Unbundle(w1965) -> ("T-RISE mins"=w1964:dbl)  [unwired: 4 out]
                    n1142 = Greater Or Equal?(x=w1967, y=w1966) -> (x >= y?=w1968:bool)
                    n1143 = case shown="True" w1968 {
                      tunnel: w1964 -> [w1971 _]
                      tunnel: w1963 -> [w1970 _]
                      tunnel: w1962 -> [w1969 _]
                      frame True {
                        n1144 = stacked-sequence {
                          tunnel: w1971 -> [w1974 _]
                          tunnel: w1970 -> [_ w1979]
                          tunnel: w1969 -> [w1972 _]
                          frame #0 {
                            n1145 = Build Array("T-RISE") -> (w1976:string[])
                            n1146 = Build Array(w1974) -> (w1975:dbl[])
                            n1147 = TDMS Write(0:w1972, 5:"TEST PASS", 7:w1976, 9:w1975) -> (15:w1978:errorcluster)  [unwired: 2 in, 3 out]
                            n1148 = local write "data file error"(w1978) -> ()
                          }
                          frame #1 {
                            n1149 = Bundle(cluster=w1979, "STATUS"="T-RISE PASS") -> (w1981:T4)  [unwired: 2 in]
                            n1150 = local write "RESULT LAB04-2"(TRUE) -> ()
                            n1151 = local write "DISP LAB04-2"(w1981) -> ()
                          }
                        }
                      }
                      frame False {
                      }
                    }
                  }
                }
              }
              frame #8 {
                # "LAB05-1"
                n1152 = Equal?(x=w1984, y=2) -> (x = y?=w1987:bool)
                n1153 = local read "DISP LAB05-1"() -> (w1989:T4)
                n1154 = Unbundle(w1989) -> ("STATUS"=w1990:string)  [unwired: 2 out]
                n1155 = Equal?(x=w1990, y="RUN") -> (x = y?=w1986:bool)
                n1156 = And(x=w1986, y=w1987) -> (x .and. y?=w1985:bool)
                n1157 = case shown="True" w1985 {
                  tunnel: w1989 -> [_ w1993]
                  tunnel: w1983 -> [_ w1996]
                  frame False {
                  }
                  frame True {
                    n1158 = local read "SET LAB05-1"() -> (w1995:T5)
                    n1159 = local read "TDMS LAB05-1"() -> (w1992:refnum<k34>)
                    n1160 = Unbundle(w1993) -> ("CYCLE"=w1997:dbl)  [unwired: 2 out]
                    n1161 = Unbundle(w1995) -> ("T-RISE mins"=w1994:dbl)  [unwired: 4 out]
                    n1162 = Greater Or Equal?(x=w1997, y=w1996) -> (x >= y?=w1998:bool)
                    n1163 = case shown="True" w1998 {
                      tunnel: w1994 -> [w2001 _]
                      tunnel: w1993 -> [w2000 _]
                      tunnel: w1992 -> [w1999 _]
                      frame True {
                        n1164 = stacked-sequence {
                          tunnel: w2001 -> [w2004 _]
                          tunnel: w2000 -> [_ w2009]
                          tunnel: w1999 -> [w2002 _]
                          frame #0 {
                            n1165 = Build Array("T-RISE") -> (w2006:string[])
                            n1166 = Build Array(w2004) -> (w2005:dbl[])
                            n1167 = TDMS Write(0:w2002, 5:"TEST PASS", 7:w2006, 9:w2005) -> (15:w2008:errorcluster)  [unwired: 2 in, 3 out]
                            n1168 = local write "data file error"(w2008) -> ()
                          }
                          frame #1 {
                            n1169 = Bundle(cluster=w2009, "STATUS"="T-RISE PASS") -> (w2011:T4)  [unwired: 2 in]
                            n1170 = local write "RESULT LAB05-1"(TRUE) -> ()
                            n1171 = local write "DISP LAB05-1"(w2011) -> ()
                          }
                        }
                      }
                      frame False {
                      }
                    }
                  }
                }
              }
              frame #9 {
                # "LAB05-2"
                n1172 = Equal?(x=w2014, y=2) -> (x = y?=w2017:bool)
                n1173 = local read "DISP LAB05-2"() -> (w2019:T4)
                n1174 = Unbundle(w2019) -> ("STATUS"=w2020:string)  [unwired: 2 out]
                n1175 = Equal?(x=w2020, y="RUN") -> (x = y?=w2016:bool)
                n1176 = And(x=w2016, y=w2017) -> (x .and. y?=w2015:bool)
                n1177 = case shown="True" w2015 {
                  tunnel: w2019 -> [_ w2023]
                  tunnel: w2013 -> [_ w2026]
                  frame False {
                  }
                  frame True {
                    n1178 = local read "SET LAB05-2"() -> (w2025:T5)
                    n1179 = local read "TDMS LAB05-2"() -> (w2022:refnum<k34>)
                    n1180 = Unbundle(w2023) -> ("CYCLE"=w2027:dbl)  [unwired: 2 out]
                    n1181 = Unbundle(w2025) -> ("T-RISE mins"=w2024:dbl)  [unwired: 4 out]
                    n1182 = Greater Or Equal?(x=w2027, y=w2026) -> (x >= y?=w2028:bool)
                    n1183 = case shown="True" w2028 {
                      tunnel: w2024 -> [w2031 _]
                      tunnel: w2023 -> [w2030 _]
                      tunnel: w2022 -> [w2029 _]
                      frame True {
                        n1184 = stacked-sequence {
                          tunnel: w2031 -> [w2034 _]
                          tunnel: w2030 -> [_ w2039]
                          tunnel: w2029 -> [w2032 _]
                          frame #0 {
                            n1185 = Build Array("T-RISE") -> (w2036:string[])
                            n1186 = Build Array(w2034) -> (w2035:dbl[])
                            n1187 = TDMS Write(0:w2032, 5:"TEST PASS", 7:w2036, 9:w2035) -> (15:w2038:errorcluster)  [unwired: 2 in, 3 out]
                            n1188 = local write "data file error"(w2038) -> ()
                          }
                          frame #1 {
                            n1189 = Bundle(cluster=w2039, "STATUS"="T-RISE PASS") -> (w2041:T4)  [unwired: 2 in]
                            n1190 = local write "RESULT LAB05-2"(TRUE) -> ()
                            n1191 = local write "DISP LAB05-2"(w2041) -> ()
                          }
                        }
                      }
                      frame False {
                      }
                    }
                  }
                }
              }
            }
          }
          frame #6 {
            # "end test & close test files"
            n1192 = stacked-sequence {
              tunnel: w2052 -> [_ _ _ _ _ _ _ _ _ _]
              tunnel: w2053 -> [_ _ _ _ _ _ _ _ _ _]
              tunnel: w2051 -> [_ _ _ _ _ _ _ _ _ _]
              tunnel: w2050 -> [_ _ _ _ _ _ _ _ _ _]
              tunnel: w2049 -> [_ _ _ _ _ _ _ _ _ _]
              tunnel: w2048 -> [_ _ _ _ _ _ _ _ _ _]
              tunnel: w2047 -> [_ _ _ _ _ _ _ _ _ _]
              tunnel: w2046 -> [_ _ _ _ _ _ _ _ _ _]
              tunnel: w2045 -> [_ _ _ _ _ _ _ _ _ _]
              tunnel: w2044 -> [_ _ _ _ _ _ _ _ _ _]
              frame #0 {
                # "LAB01-1"
                n1193 = local read "DISP LAB01-1"() -> (w2057:T4)
                n1194 = local read "run lab01-1"() -> (w2054:bool)
                n1195 = local read "TDMS LAB01-1"() -> (w2055:refnum<k34>)
                n1196 = Unbundle(w2057) -> ("CYCLE"=w2058:dbl, "STATUS"=w2056:string)  [unwired: 1 out]
                n1197 = case shown="True" w2054 {
                  tunnel: w2058 -> [_ w2062]
                  tunnel: w2057 -> [_ w2061]
                  tunnel: w2056 -> [_ w2060]
                  tunnel: w2055 -> [_ w2059]
                  frame False {
                  }
                  frame True {
                    n1198 = Not Equal?(x=w2060, y="RUN") -> (x != y?=w2063:bool)
                    n1199 = Greater?(x=w2062, y=2.0) -> (0:w2065:bool)
                    n1200 = And(x=w2065, y=w2063) -> (x .and. y?=w2064:bool)
                    n1201 = case shown="True" w2064 {
                      tunnel: w2061 -> [_ w2069]
                      tunnel: w2059 -> [_ w2068]
                      frame False {
                      }
                      frame True {
                        n1202 = stacked-sequence {
                          tunnel: w2069 -> [w2072 _ _]
                          tunnel: w2068 -> [_ w2074 _]
                          frame #0 {
                            n1203 = local write "mail control"("END") -> ()
                            n1204 = Bundle(cluster=w2072) -> (w2071:T4)  [unwired: 3 in]
                            n1205 = local write "DISP LAB01-1"(w2071) -> ()
                          }
                          frame #1 {
                            n1206 = TDMS Close(11:w2074) -> (0:w2073:errorcluster)  [unwired: 1 in, 1 out]
                            n1207 = local write "data file error"(w2073) -> ()
                          }
                          frame #2 {
                            w2075 = FALSE
                            n1208 = local write "run lab01-1"(w2075) -> ()
                            n1209 = local write "RUN LAB01-1"(w2075) -> ()
                            n1210 = call "Save data file to network drive v1.vi"("panel id"="LAB01-1") -> ("network file save error"=w2076:errorcluster)  [unwired: 9 in, 1 out]
                            n1211 = local write "data file error"(w2076) -> ()
                          }
                        }
                      }
                    }
                  }
                }
              }
              frame #1 {
                # "LAB01-2"
                n1212 = local read "run lab01-2"() -> (w2078:bool)
                n1213 = case shown="True" w2078 {
                  frame False {
                  }
                  frame True {
                    n1214 = local read "DISP LAB01-2"() -> (w2085:T4)
                    n1215 = local read "TDMS LAB01-2"() -> (w2084:refnum<k34>)
                    n1216 = Unbundle(w2085) -> ("CYCLE"=w2081:dbl, "STATUS"=w2086:string)  [unwired: 1 out]
                    n1217 = Not Equal?(x=w2086, y="RUN") -> (x != y?=w2080:bool)
                    n1218 = Greater?(x=w2081, y=2.0) -> (0:w2082:bool)
                    n1219 = And(x=w2082, y=w2080) -> (x .and. y?=w2079:bool)
                    n1220 = case shown="True" w2079 {
                      tunnel: w2085 -> [_ w2089]
                      tunnel: w2084 -> [_ w2088]
                      frame False {
                      }
                      frame True {
                        n1221 = stacked-sequence {
                          tunnel: w2089 -> [w2092 _ _]
                          tunnel: w2088 -> [_ w2094 _]
                          frame #0 {
                            w2090 = FALSE
                            n1222 = local write "mail control"("END") -> ()
                            n1223 = Bundle(cluster=w2092) -> (w2093:T4)  [unwired: 3 in]
                            n1224 = local write "RUN LAB01-2"(w2090) -> ()
                            n1225 = local write "run lab01-2"(w2090) -> ()
                            n1226 = local write "DISP LAB01-2"(w2093) -> ()
                          }
                          frame #1 {
                            n1227 = TDMS Close(11:w2094) -> (0:w2095:errorcluster)  [unwired: 1 in, 1 out]
                            n1228 = local write "data file error"(w2095) -> ()
                          }
                          frame #2 {
                            n1229 = call "Save data file to network drive v1.vi"("panel id"="LAB01-2") -> ("network file save error"=w2096:errorcluster)  [unwired: 9 in, 1 out]
                            n1230 = local write "data file error"(w2096) -> ()
                          }
                        }
                      }
                    }
                  }
                }
              }
              frame #2 {
                # "LAB02-1"
                n1231 = local read "run lab02-1"() -> (w2098:bool)
                n1232 = case shown="True" w2098 {
                  frame False {
                  }
                  frame True {
                    n1233 = local read "DISP LAB02-1"() -> (w2105:T4)
                    n1234 = Unbundle(w2105) -> ("CYCLE"=w2101:dbl, "STATUS"=w2106:string)  [unwired: 1 out]
                    n1235 = local read "TDMS LAB02-1"() -> (w2104:refnum<k34>)
                    n1236 = Not Equal?(x=w2106, y="RUN") -> (x != y?=w2100:bool)
                    n1237 = Greater?(x=w2101, y=2.0) -> (0:w2102:bool)
                    n1238 = And(x=w2102, y=w2100) -> (x .and. y?=w2099:bool)
                    n1239 = case shown="True" w2099 {
                      tunnel: w2105 -> [_ w2109]
                      tunnel: w2104 -> [_ w2108]
                      frame False {
                      }
                      frame True {
                        n1240 = stacked-sequence {
                          tunnel: w2109 -> [w2112 _ _]
                          tunnel: w2108 -> [_ w2114 _]
                          frame #0 {
                            w2110 = FALSE
                            n1241 = local write "mail control"("END") -> ()
                            n1242 = Bundle(cluster=w2112) -> (w2113:T4)  [unwired: 3 in]
                            n1243 = local write "RUN LAB02-1"(w2110) -> ()
                            n1244 = local write "run lab02-1"(w2110) -> ()
                            n1245 = local write "DISP LAB02-1"(w2113) -> ()
                          }
                          frame #1 {
                            n1246 = TDMS Close(11:w2114) -> (0:w2115:errorcluster)  [unwired: 1 in, 1 out]
                            n1247 = local write "data file error"(w2115) -> ()
                          }
                          frame #2 {
                            n1248 = call "Save data file to network drive v1.vi"("panel id"="LAB02-1") -> ("network file save error"=w2116:errorcluster)  [unwired: 9 in, 1 out]
                            n1249 = local write "data file error"(w2116) -> ()
                          }
                        }
                      }
                    }
                  }
                }
              }
              frame #3 {
                # "LAB02-2"
                n1250 = local read "run lab02-2"() -> (w2118:bool)
                n1251 = case shown="True" w2118 {
                  frame False {
                  }
                  frame True {
                    n1252 = local read "DISP LAB02-2"() -> (w2125:T4)
                    n1253 = local read "TDMS LAB02-2"() -> (w2124:refnum<k34>)
                    n1254 = Unbundle(w2125) -> ("CYCLE"=w2121:dbl, "STATUS"=w2126:string)  [unwired: 1 out]
                    n1255 = Not Equal?(x=w2126, y="RUN") -> (x != y?=w2120:bool)
                    n1256 = Greater?(x=w2121, y=2.0) -> (0:w2122:bool)
                    n1257 = And(x=w2122, y=w2120) -> (x .and. y?=w2119:bool)
                    n1258 = case shown="True" w2119 {
                      tunnel: w2125 -> [_ w2129]
                      tunnel: w2124 -> [_ w2128]
                      frame False {
                      }
                      frame True {
                        n1259 = stacked-sequence {
                          tunnel: w2129 -> [w2132 _ _]
                          tunnel: w2128 -> [_ w2134 _]
                          frame #0 {
                            w2130 = FALSE
                            n1260 = local write "mail control"("END") -> ()
                            n1261 = Bundle(cluster=w2132) -> (w2133:T4)  [unwired: 3 in]
                            n1262 = local write "run lab02-2"(w2130) -> ()
                            n1263 = local write "RUN LAB02-2"(w2130) -> ()
                            n1264 = local write "DISP LAB02-2"(w2133) -> ()
                          }
                          frame #1 {
                            n1265 = TDMS Close(11:w2134) -> (0:w2135:errorcluster)  [unwired: 1 in, 1 out]
                            n1266 = local write "data file error"(w2135) -> ()
                          }
                          frame #2 {
                            n1267 = call "Save data file to network drive v1.vi"("panel id"="LAB02-2") -> ("network file save error"=w2136:errorcluster)  [unwired: 9 in, 1 out]
                            n1268 = local write "data file error"(w2136) -> ()
                          }
                        }
                      }
                    }
                  }
                }
              }
              frame #4 {
                # "LAB03-1"
                n1269 = local read "run lab03-1"() -> (w2138:bool)
                n1270 = case shown="True" w2138 {
                  frame False {
                  }
                  frame True {
                    n1271 = local read "DISP LAB03-1"() -> (w2145:T4)
                    n1272 = local read "TDMS LAB03-1"() -> (w2144:refnum<k34>)
                    n1273 = Unbundle(w2145) -> ("CYCLE"=w2141:dbl, "STATUS"=w2146:string)  [unwired: 1 out]
                    n1274 = Not Equal?(x=w2146, y="RUN") -> (x != y?=w2140:bool)
                    n1275 = Greater?(x=w2141, y=2.0) -> (0:w2142:bool)
                    n1276 = And(x=w2142, y=w2140) -> (x .and. y?=w2139:bool)
                    n1277 = case shown="True" w2139 {
                      tunnel: w2145 -> [_ w2149]
                      tunnel: w2144 -> [_ w2148]
                      frame False {
                      }
                      frame True {
                        n1278 = stacked-sequence {
                          tunnel: w2149 -> [w2152 _ _]
                          tunnel: w2148 -> [_ w2154 _]
                          frame #0 {
                            w2150 = FALSE
                            n1279 = local write "mail control"("END") -> ()
                            n1280 = Bundle(cluster=w2152) -> (w2153:T4)  [unwired: 3 in]
                            n1281 = local write "run lab03-1"(w2150) -> ()
                            n1282 = local write "RUN LAB03-1"(w2150) -> ()
                            n1283 = local write "DISP LAB03-1"(w2153) -> ()
                          }
                          frame #1 {
                            n1284 = TDMS Close(11:w2154) -> (0:w2155:errorcluster)  [unwired: 1 in, 1 out]
                            n1285 = local write "data file error"(w2155) -> ()
                          }
                          frame #2 {
                            n1286 = call "Save data file to network drive v1.vi"("panel id"="LAB03-1") -> ("network file save error"=w2156:errorcluster)  [unwired: 9 in, 1 out]
                            n1287 = local write "data file error"(w2156) -> ()
                          }
                        }
                      }
                    }
                  }
                }
              }
              frame #5 {
                # "LAB03-2"
                n1288 = local read "run lab03-2"() -> (w2158:bool)
                n1289 = case shown="True" w2158 {
                  frame False {
                  }
                  frame True {
                    n1290 = local read "DISP LAB03-2"() -> (w2165:T4)
                    n1291 = Unbundle(w2165) -> ("CYCLE"=w2161:dbl, "STATUS"=w2166:string)  [unwired: 1 out]
                    n1292 = local read "TDMS LAB03-2"() -> (w2164:refnum<k34>)
                    n1293 = Not Equal?(x=w2166, y="RUN") -> (x != y?=w2160:bool)
                    n1294 = Greater?(x=w2161, y=2.0) -> (0:w2162:bool)
                    n1295 = And(x=w2162, y=w2160) -> (x .and. y?=w2159:bool)
                    n1296 = case shown="True" w2159 {
                      tunnel: w2165 -> [_ w2169]
                      tunnel: w2164 -> [_ w2168]
                      frame False {
                      }
                      frame True {
                        n1297 = stacked-sequence {
                          tunnel: w2169 -> [w2172 _ _]
                          tunnel: w2168 -> [_ w2174 _]
                          frame #0 {
                            w2170 = FALSE
                            n1298 = local write "mail control"("END") -> ()
                            n1299 = Bundle(cluster=w2172) -> (w2173:T4)  [unwired: 3 in]
                            n1300 = local write "RUN LAB03-2"(w2170) -> ()
                            n1301 = local write "DISP LAB03-2"(w2173) -> ()
                            n1302 = local write "run lab03-2"(w2170) -> ()
                          }
                          frame #1 {
                            n1303 = TDMS Close(11:w2174) -> (0:w2175:errorcluster)  [unwired: 1 in, 1 out]
                            n1304 = local write "data file error"(w2175) -> ()
                          }
                          frame #2 {
                            n1305 = call "Save data file to network drive v1.vi"("panel id"="LAB03-2") -> ("network file save error"=w2176:errorcluster)  [unwired: 9 in, 1 out]
                            n1306 = local write "data file error"(w2176) -> ()
                          }
                        }
                      }
                    }
                  }
                }
              }
              frame #6 {
                # "LAB04-1"
                n1307 = local read "run lab04-1"() -> (w2178:bool)
                n1308 = case shown="True" w2178 {
                  frame False {
                  }
                  frame True {
                    n1309 = local read "DISP LAB04-1"() -> (w2185:T4)
                    n1310 = Unbundle(w2185) -> ("CYCLE"=w2181:dbl, "STATUS"=w2186:string)  [unwired: 1 out]
                    n1311 = local read "TDMS LAB04-1"() -> (w2184:refnum<k34>)
                    n1312 = Not Equal?(x=w2186, y="RUN") -> (x != y?=w2180:bool)
                    n1313 = Greater?(x=w2181, y=2.0) -> (0:w2182:bool)
                    n1314 = And(x=w2182, y=w2180) -> (x .and. y?=w2179:bool)
                    n1315 = case shown="True" w2179 {
                      tunnel: w2185 -> [_ w2189]
                      tunnel: w2184 -> [_ w2188]
                      frame False {
                      }
                      frame True {
                        n1316 = stacked-sequence {
                          tunnel: w2189 -> [w2192 _ _]
                          tunnel: w2188 -> [_ w2194 _]
                          frame #0 {
                            w2190 = FALSE
                            n1317 = local write "mail control"("END") -> ()
                            n1318 = Bundle(cluster=w2192) -> (w2193:T4)  [unwired: 3 in]
                            n1319 = local write "RUN LAB04-1"(w2190) -> ()
                            n1320 = local write "run lab04-1"(w2190) -> ()
                            n1321 = local write "DISP LAB04-1"(w2193) -> ()
                          }
                          frame #1 {
                            n1322 = TDMS Close(11:w2194) -> (0:w2195:errorcluster)  [unwired: 1 in, 1 out]
                            n1323 = local write "data file error"(w2195) -> ()
                          }
                          frame #2 {
                            n1324 = call "Save data file to network drive v1.vi"("panel id"="LAB04-1") -> ("network file save error"=w2196:errorcluster)  [unwired: 9 in, 1 out]
                            n1325 = local write "data file error"(w2196) -> ()
                          }
                        }
                      }
                    }
                  }
                }
              }
              frame #7 {
                # "LAB04-2"
                n1326 = local read "run lab04-2"() -> (w2198:bool)
                n1327 = case shown="True" w2198 {
                  frame False {
                  }
                  frame True {
                    n1328 = local read "DISP LAB04-2"() -> (w2205:T4)
                    n1329 = Unbundle(w2205) -> ("CYCLE"=w2201:dbl, "STATUS"=w2206:string)  [unwired: 1 out]
                    n1330 = Not Equal?(x=w2206, y="RUN") -> (x != y?=w2200:bool)
                    n1331 = local read "TDMS LAB04-2"() -> (w2204:refnum<k34>)
                    n1332 = Greater?(x=w2201, y=2.0) -> (0:w2202:bool)
                    n1333 = And(x=w2202, y=w2200) -> (x .and. y?=w2199:bool)
                    n1334 = case shown="True" w2199 {
                      tunnel: w2205 -> [_ w2209]
                      tunnel: w2204 -> [_ w2208]
                      frame False {
                      }
                      frame True {
                        n1335 = stacked-sequence {
                          tunnel: w2209 -> [w2212 _ _]
                          tunnel: w2208 -> [_ w2214 _]
                          frame #0 {
                            w2210 = FALSE
                            n1336 = local write "mail control"("END") -> ()
                            n1337 = Bundle(cluster=w2212) -> (w2213:T4)  [unwired: 3 in]
                            n1338 = local write "RUN LAB04-2"(w2210) -> ()
                            n1339 = local write "run lab04-2"(w2210) -> ()
                            n1340 = local write "DISP LAB04-2"(w2213) -> ()
                          }
                          frame #1 {
                            n1341 = TDMS Close(11:w2214) -> (0:w2215:errorcluster)  [unwired: 1 in, 1 out]
                            n1342 = local write "data file error"(w2215) -> ()
                          }
                          frame #2 {
                            n1343 = call "Save data file to network drive v1.vi"("panel id"="LAB04-2") -> ("network file save error"=w2216:errorcluster)  [unwired: 9 in, 1 out]
                            n1344 = local write "data file error"(w2216) -> ()
                          }
                        }
                      }
                    }
                  }
                }
              }
              frame #8 {
                # "LAB05-1"
                n1345 = local read "run lab05-1"() -> (w2218:bool)
                n1346 = case shown="True" w2218 {
                  frame False {
                  }
                  frame True {
                    n1347 = local read "DISP LAB05-1"() -> (w2225:T4)
                    n1348 = Unbundle(w2225) -> ("CYCLE"=w2221:dbl, "STATUS"=w2226:string)  [unwired: 1 out]
                    n1349 = Not Equal?(x=w2226, y="RUN") -> (x != y?=w2220:bool)
                    n1350 = local read "TDMS LAB05-1"() -> (w2224:refnum<k34>)
                    n1351 = Greater?(x=w2221, y=2.0) -> (0:w2222:bool)
                    n1352 = And(x=w2222, y=w2220) -> (x .and. y?=w2219:bool)
                    n1353 = case shown="True" w2219 {
                      tunnel: w2225 -> [_ w2229]
                      tunnel: w2224 -> [_ w2228]
                      frame False {
                      }
                      frame True {
                        n1354 = stacked-sequence {
                          tunnel: w2229 -> [w2232 _ _]
                          tunnel: w2228 -> [_ w2234 _]
                          frame #0 {
                            w2230 = FALSE
                            n1355 = local write "mail control"("END") -> ()
                            n1356 = Bundle(cluster=w2232) -> (w2233:T4)  [unwired: 3 in]
                            n1357 = local write "RUN LAB05-1"(w2230) -> ()
                            n1358 = local write "run lab05-1"(w2230) -> ()
                            n1359 = local write "DISP LAB05-1"(w2233) -> ()
                          }
                          frame #1 {
                            n1360 = TDMS Close(11:w2234) -> (0:w2235:errorcluster)  [unwired: 1 in, 1 out]
                            n1361 = local write "data file error"(w2235) -> ()
                          }
                          frame #2 {
                            n1362 = call "Save data file to network drive v1.vi"("panel id"="LAB05-1") -> ("network file save error"=w2236:errorcluster)  [unwired: 9 in, 1 out]
                            n1363 = local write "data file error"(w2236) -> ()
                          }
                        }
                      }
                    }
                  }
                }
              }
              frame #9 {
                # "LAB05-2"
                n1364 = local read "run lab05-2"() -> (w2238:bool)
                n1365 = case shown="True" w2238 {
                  frame False {
                  }
                  frame True {
                    n1366 = local read "DISP LAB05-2"() -> (w2245:T4)
                    n1367 = Unbundle(w2245) -> ("CYCLE"=w2241:dbl, "STATUS"=w2246:string)  [unwired: 1 out]
                    n1368 = Not Equal?(x=w2246, y="RUN") -> (x != y?=w2240:bool)
                    n1369 = local read "TDMS LAB05-2"() -> (w2244:refnum<k34>)
                    n1370 = Greater?(x=w2241, y=2.0) -> (0:w2242:bool)
                    n1371 = And(x=w2242, y=w2240) -> (x .and. y?=w2239:bool)
                    n1372 = case shown="True" w2239 {
                      tunnel: w2245 -> [_ w2249]
                      tunnel: w2244 -> [_ w2248]
                      frame False {
                      }
                      frame True {
                        n1373 = stacked-sequence {
                          tunnel: w2249 -> [w2252 _ _]
                          tunnel: w2248 -> [_ w2254 _]
                          frame #0 {
                            w2250 = FALSE
                            n1374 = local write "mail control"("END") -> ()
                            n1375 = Bundle(cluster=w2252) -> (w2253:T4)  [unwired: 3 in]
                            n1376 = local write "RUN LAB05-2"(w2250) -> ()
                            n1377 = local write "run lab05-2"(w2250) -> ()
                            n1378 = local write "DISP LAB05-2"(w2253) -> ()
                          }
                          frame #1 {
                            n1379 = TDMS Close(11:w2254) -> (0:w2255:errorcluster)  [unwired: 1 in, 1 out]
                            n1380 = local write "data file error"(w2255) -> ()
                          }
                          frame #2 {
                            n1381 = call "Save data file to network drive v1.vi"("panel id"="LAB05-2") -> ("network file save error"=w2256:errorcluster)  [unwired: 9 in, 1 out]
                            n1382 = local write "data file error"(w2256) -> ()
                          }
                        }
                      }
                    }
                  }
                }
              }
            }
            n1383 = local read "Network Directory"() -> (w2043:path)
            n1384 = global write "Global 1.vi" "Network Drive"(w2043) -> ()
          }
          frame #7 {
            # "disable functions"
            n1385 = stacked-sequence {
              tunnel: w2267 -> [w2281 _ w2337]
              tunnel: w2266 -> [w2276 _ w2336]
              tunnel: w2265 -> [w2275 _ w2335]
              tunnel: w2264 -> [w2273 _ w2334]
              tunnel: w2263 -> [w2274 _ w2333]
              tunnel: w2262 -> [_ w2298 w2332]
              tunnel: w2261 -> [_ w2299 w2331]
              tunnel: w2260 -> [_ w2300 w2330]
              tunnel: w2259 -> [_ w2301 w2329]
              tunnel: w2258 -> [_ w2302 w2328]
              frame #0 {
                n1386 = Select(t=2, s=w2273, f=0) -> (s? t:f=w2269:i32)
                n1387 = Select(t=2, s=w2275, f=0) -> (s? t:f=w2270:i32)
                n1388 = Select(t=2, s=w2274, f=0) -> (s? t:f=w2268:i32)
                n1389 = Select(t=2, s=w2281, f=0) -> (s? t:f=w2272:i32)
                n1390 = Select(t=2, s=w2276, f=0) -> (s? t:f=w2271:i32)
                n1391 = property on="SELECT LAB02-2" class="RadioBtnsControl (strict)"("DisabledEnum"=w2269) -> ()  [unwired: 2 in, 2 out]
                n1392 = property on="SELECT LAB02-1" class="RadioBtnsControl (strict)"("DisabledEnum"=w2270) -> ()  [unwired: 2 in, 2 out]
                n1393 = property on="SELECT LAB03-1" class="RadioBtnsControl (strict)"("DisabledEnum"=w2268) -> ()  [unwired: 2 in, 2 out]
                n1394 = property on="SELECT LAB01-1" class="RadioBtnsControl (strict)"("DisabledEnum"=w2272) -> ()  [unwired: 2 in, 2 out]
                n1395 = property on="SELECT LAB01-2" class="RadioBtnsControl (strict)"("DisabledEnum"=w2271) -> ()  [unwired: 2 in, 2 out]
                n1396 = Not(x=w2281) -> (.not. x?=w2282:bool)
                n1397 = property on="RESULT LAB01-1" class="Bool (strict)"("Visible"=w2282) -> ()  [unwired: 2 in, 2 out]
                n1398 = Not(x=w2276) -> (.not. x?=w2280:bool)
                n1399 = Not(x=w2275) -> (.not. x?=w2279:bool)
                n1400 = Not(x=w2273) -> (.not. x?=w2278:bool)
                n1401 = property on="RESULT LAB01-2" class="Bool (strict)"("Visible"=w2280) -> ()  [unwired: 2 in, 2 out]
                n1402 = Not(x=w2274) -> (.not. x?=w2277:bool)
                n1403 = property on="RESULT LAB02-1" class="Bool (strict)"("Visible"=w2279) -> ()  [unwired: 2 in, 2 out]
                n1404 = property on="RESULT LAB02-2" class="Bool (strict)"("Visible"=w2278) -> ()  [unwired: 2 in, 2 out]
                n1405 = property on="RESULT LAB03-1" class="Bool (strict)"("Visible"=w2277) -> ()  [unwired: 2 in, 2 out]
                n1406 = property on="SET LAB01-1" class="Clust (strict)"("DisabledEnum"=w2272) -> ()  [unwired: 2 in, 2 out]
                n1407 = property on="SET LAB01-2" class="Clust (strict)"("DisabledEnum"=w2271) -> ()  [unwired: 2 in, 2 out]
                n1408 = property on="SET LAB02-1" class="Clust (strict)"("DisabledEnum"=w2270) -> ()  [unwired: 2 in, 2 out]
                n1409 = property on="SET LAB02-2" class="Clust (strict)"("DisabledEnum"=w2269) -> ()  [unwired: 2 in, 2 out]
                n1410 = property on="SET LAB03-1" class="Clust (strict)"("DisabledEnum"=w2268) -> ()  [unwired: 2 in, 2 out]
                n1411 = property on="O/I  LAB01-1" class="Bool (strict)"("DisabledEnum"=w2272) -> ()  [unwired: 2 in, 2 out]
                n1412 = property on="O/I  LAB01-2" class="Bool (strict)"("DisabledEnum"=w2271) -> ()  [unwired: 2 in, 2 out]
                n1413 = property on="O/I  LAB02-1" class="Bool (strict)"("DisabledEnum"=w2270) -> ()  [unwired: 2 in, 2 out]
                n1414 = property on="O/1  LAB02-2" class="Bool (strict)"("DisabledEnum"=w2269) -> ()  [unwired: 2 in, 2 out]
                n1415 = property on="O/I  LAB03-1" class="Bool (strict)"("DisabledEnum"=w2268) -> ()  [unwired: 2 in, 2 out]
              }
              frame #1 {
                n1416 = Select(t=2, s=w2302, f=0) -> (s? t:f=w2293:i32)
                n1417 = Select(t=2, s=w2301, f=0) -> (s? t:f=w2294:i32)
                n1418 = Select(t=2, s=w2298, f=0) -> (s? t:f=w2297:i32)
                n1419 = Select(t=2, s=w2299, f=0) -> (s? t:f=w2296:i32)
                n1420 = Select(t=2, s=w2300, f=0) -> (s? t:f=w2295:i32)
                n1421 = property on="SELECT LAB05-2" class="RadioBtnsControl (strict)"("DisabledEnum"=w2293) -> ()  [unwired: 2 in, 2 out]
                n1422 = property on="SELECT LAB05-1" class="RadioBtnsControl (strict)"("DisabledEnum"=w2294) -> ()  [unwired: 2 in, 2 out]
                n1423 = property on="SELECT LAB03-2" class="RadioBtnsControl (strict)"("DisabledEnum"=w2297) -> ()  [unwired: 2 in, 2 out]
                n1424 = property on="SELECT LAB04-1" class="RadioBtnsControl (strict)"("DisabledEnum"=w2296) -> ()  [unwired: 2 in, 2 out]
                n1425 = property on="SELECT LAB04-2" class="RadioBtnsControl (strict)"("DisabledEnum"=w2295) -> ()  [unwired: 2 in, 2 out]
                n1426 = property on="SET LAB05-2" class="Clust (strict)"("DisabledEnum"=w2293) -> ()  [unwired: 2 in, 2 out]
                n1427 = property on="SET LAB05-1" class="Clust (strict)"("DisabledEnum"=w2294) -> ()  [unwired: 2 in, 2 out]
                n1428 = property on="SET LAB03-2" class="Clust (strict)"("DisabledEnum"=w2297) -> ()  [unwired: 2 in, 2 out]
                n1429 = property on="SET LAB04-1" class="Clust (strict)"("DisabledEnum"=w2296) -> ()  [unwired: 2 in, 2 out]
                n1430 = property on="SET LAB04-2" class="Clust (strict)"("DisabledEnum"=w2295) -> ()  [unwired: 2 in, 2 out]
                n1431 = property on="O/I  LAB05-2" class="Bool (strict)"("DisabledEnum"=w2293) -> ()  [unwired: 2 in, 2 out]
                n1432 = property on="O/I  LAB05-1" class="Bool (strict)"("DisabledEnum"=w2294) -> ()  [unwired: 2 in, 2 out]
                n1433 = property on="O/I  LAB04-1" class="Bool (strict)"("DisabledEnum"=w2296) -> ()  [unwired: 2 in, 2 out]
                n1434 = property on="O/I  LAB04-2" class="Bool (strict)"("DisabledEnum"=w2295) -> ()  [unwired: 2 in, 2 out]
                n1435 = property on="O/I  LAB03-2" class="Bool (strict)"("DisabledEnum"=w2297) -> ()  [unwired: 2 in, 2 out]
                n1436 = Not(x=w2302) -> (.not. x?=w2303:bool)
                n1437 = Not(x=w2301) -> (.not. x?=w2304:bool)
                n1438 = Not(x=w2300) -> (.not. x?=w2305:bool)
                n1439 = property on="RESULT LAB05-2" class="Bool (strict)"("Visible"=w2303) -> ()  [unwired: 2 in, 2 out]
                n1440 = property on="RESULT LAB05-1" class="Bool (strict)"("Visible"=w2304) -> ()  [unwired: 2 in, 2 out]
                n1441 = Not(x=w2299) -> (.not. x?=w2306:bool)
                n1442 = property on="RESULT LAB04-2" class="Bool (strict)"("Visible"=w2305) -> ()  [unwired: 2 in, 2 out]
                n1443 = Not(x=w2298) -> (.not. x?=w2307:bool)
                n1444 = property on="RESULT LAB04-1" class="Bool (strict)"("Visible"=w2306) -> ()  [unwired: 2 in, 2 out]
                n1445 = property on="RESULT LAB03-2" class="Bool (strict)"("Visible"=w2307) -> ()  [unwired: 2 in, 2 out]
              }
              frame #2 {
                # "disable calibrate if any test running"
                n1446 = Or(x=w2329, y=w2328) -> (x .or. y?=w2322:bool)
                n1447 = Or(x=w2331, y=w2330) -> (x .or. y?=w2324:bool)
                n1448 = Or(x=w2335, y=w2334) -> (x .or. y?=w2326:bool)
                n1449 = Or(x=w2333, y=w2332) -> (x .or. y?=w2325:bool)
                n1450 = Or(x=w2337, y=w2336) -> (x .or. y?=w2327:bool)
                n1451 = Or(x=w2325, y=w2324) -> (x .or. y?=w2323:bool)
                n1452 = Or(x=w2327, y=w2326) -> (x .or. y?=w2321:bool)
                n1453 = Or(x=w2323, y=w2322) -> (x .or. y?=w2320:bool)
                n1454 = Or(x=w2321, y=w2320) -> (x .or. y?=w2319:bool)
                n1455 = case shown="False" w2319 {
                  tunnel: [0 2] -> w2318
                  frame False {
                  }
                  frame True {
                  }
                }
                n1456 = property on="Network Directory" class="Path"("DisabledEnum"=w2318) -> ()  [unwired: 2 in, 2 out]
                n1457 = property on="MAIL SETTINGS" class="Clust (strict)"("DisabledEnum"=w2318) -> ()  [unwired: 2 in, 2 out]
                n1458 = property on="CALIBRATE" class="Bool (strict)"("DisabledEnum"=w2318) -> ()  [unwired: 2 in, 2 out]
                n1459 = property on="SHOW ADMIN PAGE" class="Bool (strict)"("DisabledEnum"=w2318) -> ()  [unwired: 2 in, 2 out]
              }
            }
          }
          frame #8 {
            # "drive jigs"
            n1460 = stacked-sequence {
              frame #0 {
                # "jig on"
                n1461 = local read "jig cycle"() -> (w2340:dbl)
                n1462 = Equal?(x=w2340, y=0) -> (x = y?=w2342:bool)
                n1463 = case shown="True" w2342 {
                  frame False {
                  }
                  frame True {
                    n1464 = local read "RUN LAB01-1"() -> (w2343:bool)
                    n1465 = local read "RUN LAB01-2"() -> (w2344:bool)
                    n1466 = local read "RUN LAB03-1"() -> (w2350:bool)
                    n1467 = local read "RUN LAB03-2"() -> (w2349:bool)
                    n1468 = local read "RUN LAB02-1"() -> (w2352:bool)
                    n1469 = local read "RUN LAB02-2"() -> (w2351:bool)
                    n1470 = local read "RUN LAB04-1"() -> (w2348:bool)
                    n1471 = local read "RUN LAB04-2"() -> (w2347:bool)
                    n1472 = local read "RUN LAB05-1"() -> (w2346:bool)
                    n1473 = local read "RUN LAB05-2"() -> (w2345:bool)
                    n1474 = local write "JIG LAB05-1"(w2346) -> ()
                    n1475 = local write "JIG LAB05-2"(w2345) -> ()
                    n1476 = local write "JIG LAB04-2"(w2347) -> ()
                    n1477 = local write "JIG LAB02-1"(w2352) -> ()
                    n1478 = local write "JIG LAB03-1"(w2350) -> ()
                    n1479 = local write "JIG LAB04-1"(w2348) -> ()
                    n1480 = local write "JIG LAB03-2"(w2349) -> ()
                    n1481 = local write "JIG LAB02-2"(w2351) -> ()
                    n1482 = local write "JIG LAB01-1"(w2343) -> ()
                    n1483 = local write "JIG LAB01-2"(w2344) -> ()
                  }
                }
              }
              frame #1 {
                # "jig off"
                n1484 = local read "jig cycle"() -> (w2355:dbl)
                n1485 = local read "on loops"() -> (w2354:dbl)
                n1486 = Equal?(x=w2355, y=w2354) -> (x = y?=w2353:bool)
                n1487 = case shown="True" w2353 {
                  frame False {
                  }
                  frame True {
                    w2406 = FALSE
                    w2407 = TRUE
                    w2405 = 2
                    n1488 = local read "SELECT LAB05-2"() -> (w2396:T3)
                    n1489 = local read "SELECT LAB04-2"() -> (w2398:T3)
                    n1490 = local read "SELECT LAB04-1"() -> (w2399:T3)
                    n1491 = local read "SELECT LAB05-1"() -> (w2397:T3)
                    n1492 = local read "SELECT LAB03-2"() -> (w2400:T3)
                    n1493 = local read "SELECT LAB02-1"() -> (w2403:T3)
                    n1494 = local read "SELECT LAB03-1"() -> (w2401:T3)
                    n1495 = local read "SELECT LAB02-2"() -> (w2402:T3)
                    n1496 = local read "SELECT LAB01-2"() -> (w2404:T3)
                    n1497 = local read "RUN LAB05-1"() -> (w2366:bool)
                    n1498 = local read "RUN LAB05-2"() -> (w2365:bool)
                    n1499 = local read "RUN LAB04-2"() -> (w2367:bool)
                    n1500 = local read "RUN LAB04-1"() -> (w2368:bool)
                    n1501 = local read "RUN LAB01-1"() -> (w2384:bool)
                    n1502 = local read "RUN LAB01-2"() -> (w2373:bool)
                    n1503 = local read "RUN LAB03-2"() -> (w2369:bool)
                    n1504 = local read "SELECT LAB01-1"() -> (w2408:T3)
                    n1505 = local read "RUN LAB03-1"() -> (w2370:bool)
                    n1506 = local read "RUN LAB02-1"() -> (w2372:bool)
                    n1507 = local read "RUN LAB02-2"() -> (w2371:bool)
                    n1508 = Equal?(x=w2405, y=w2401) -> (x = y?=w2379:bool)
                    n1509 = Equal?(x=w2405, y=w2400) -> (x = y?=w2378:bool)
                    n1510 = Equal?(x=w2405, y=w2399) -> (x = y?=w2377:bool)
                    n1511 = Equal?(x=w2405, y=w2398) -> (x = y?=w2376:bool)
                    n1512 = Equal?(x=w2405, y=w2397) -> (x = y?=w2375:bool)
                    n1513 = Equal?(x=w2405, y=w2396) -> (x = y?=w2374:bool)
                    n1514 = Equal?(x=w2405, y=w2408) -> (x = y?=w2385:bool)
                    n1515 = Equal?(x=w2405, y=w2403) -> (x = y?=w2381:bool)
                    n1516 = Equal?(x=w2405, y=w2402) -> (x = y?=w2380:bool)
                    n1517 = Equal?(x=w2405, y=w2404) -> (x = y?=w2382:bool)
                    n1518 = And(x=w2376, y=w2367) -> (x .and. y?=w2358:bool)
                    n1519 = And(x=w2379, y=w2370) -> (x .and. y?=w2361:bool)
                    n1520 = And(x=w2377, y=w2368) -> (x .and. y?=w2359:bool)
                    n1521 = And(x=w2374, y=w2365) -> (x .and. y?=w2356:bool)
                    n1522 = And(x=w2380, y=w2371) -> (x .and. y?=w2362:bool)
                    n1523 = And(x=w2378, y=w2369) -> (x .and. y?=w2360:bool)
                    n1524 = And(x=w2375, y=w2366) -> (x .and. y?=w2357:bool)
                    n1525 = And(x=w2382, y=w2373) -> (x .and. y?=w2364:bool)
                    n1526 = And(x=w2385, y=w2384) -> (x .and. y?=w2383:bool)
                    n1527 = And(x=w2381, y=w2372) -> (x .and. y?=w2363:bool)
                    n1528 = Select(t=w2407, s=w2383, f=w2406) -> (s? t:f=w2386:bool)
                    n1529 = Select(t=w2407, s=w2364, f=w2406) -> (s? t:f=w2387:bool)
                    n1530 = Select(t=w2407, s=w2363, f=w2406) -> (s? t:f=w2388:bool)
                    n1531 = Select(t=w2407, s=w2362, f=w2406) -> (s? t:f=w2389:bool)
                    n1532 = Select(t=w2407, s=w2361, f=w2406) -> (s? t:f=w2390:bool)
                    n1533 = Select(t=w2407, s=w2360, f=w2406) -> (s? t:f=w2391:bool)
                    n1534 = Select(t=w2407, s=w2359, f=w2406) -> (s? t:f=w2392:bool)
                    n1535 = Select(t=w2407, s=w2358, f=w2406) -> (s? t:f=w2393:bool)
                    n1536 = Select(t=w2407, s=w2357, f=w2406) -> (s? t:f=w2394:bool)
                    n1537 = Select(t=w2407, s=w2356, f=w2406) -> (s? t:f=w2395:bool)
                    n1538 = local write "JIG LAB03-2"(w2391) -> ()
                    n1539 = local write "JIG LAB02-1"(w2388) -> ()
                    n1540 = local write "JIG LAB02-2"(w2389) -> ()
                    n1541 = local write "JIG LAB01-2"(w2387) -> ()
                    n1542 = local write "JIG LAB03-1"(w2390) -> ()
                    n1543 = local write "JIG LAB01-1"(w2386) -> ()
                    n1544 = local write "JIG LAB05-2"(w2395) -> ()
                    n1545 = local write "JIG LAB04-1"(w2392) -> ()
                    n1546 = local write "JIG LAB05-1"(w2394) -> ()
                    n1547 = local write "JIG LAB04-2"(w2393) -> ()
                  }
                }
              }
            }
          }
          frame #9 {
            # "drive digital output"
            n1548 = local read "O/I  LAB05-2"() -> (w2414:bool)
            n1549 = local read "O/I  LAB05-1"() -> (w2416:bool)
            n1550 = local read "JIG LAB05-2"() -> (w2413:bool)
            n1551 = local read "O/I  LAB04-2"() -> (w2418:bool)
            n1552 = local read "JIG LAB05-1"() -> (w2415:bool)
            n1553 = local read "JIG LAB04-2"() -> (w2417:bool)
            n1554 = local read "O/1  LAB02-2"() -> (w2425:bool)
            n1555 = local read "O/I  LAB03-1"() -> (w2423:bool)
            n1556 = local read "O/I  LAB04-1"() -> (w2419:bool)
            n1557 = local read "O/I  LAB02-1"() -> (w2427:bool)
            n1558 = local read "O/I  LAB03-2"() -> (w2421:bool)
            n1559 = local read "JIG LAB04-1"() -> (w2412:bool)
            n1560 = local read "JIG LAB03-2"() -> (w2420:bool)
            n1561 = local read "O/I  LAB01-2"() -> (w2429:bool)
            n1562 = local read "JIG LAB02-1"() -> (w2426:bool)
            n1563 = local read "JIG LAB02-2"() -> (w2424:bool)
            n1564 = local read "JIG LAB03-1"() -> (w2422:bool)
            n1565 = local read "O/I  LAB01-1"() -> (w2431:bool)
            n1566 = local read "JIG LAB01-2"() -> (w2428:bool)
            n1567 = local read "JIG LAB01-1"() -> (w2430:bool)
            n1568 = Build Array(w2418, w2417, w2416, w2415, w2414, w2413) -> (w2409:bool[])
            n1569 = Build Array(w2424, w2423, w2422, w2421, w2420, w2419, w2412) -> (w2410:bool[])
            n1570 = Build Array(w2431, w2430, w2429, w2428, w2427, w2426, w2425) -> (w2411:bool[])
            n1571 = call "sub vi - Drive Relays All v6.vi"("Array #2"=w2409, "Array #1"=w2410, "Array #0"=w2411) -> ()  [unwired: 8 in, 1 out]
          }
          frame #10 {
            # "get temperature values"
            n1572 = stacked-sequence {
              frame #0 {
                n1573 = local read "jig cycle"() -> (w2432:dbl)
                n1574 = local read "on loops"() -> (w2435:dbl)
                n1575 = local read "jig cycle"() -> (w2437:dbl)
                n1576 = Add(x=w2435, y=2) -> (x+y=w2436:dbl)
                n1577 = Equal?(x=w2437, y=0) -> (x = y?=w2438:bool)
                n1578 = Equal?(x=w2432, y=w2436) -> (x = y?=w2433:bool)
                n1579 = case shown="True" w2438 {
                  frame False {
                  }
                  frame True {
                    w2450 = FALSE
                    w2451 = TRUE
                    n1580 = local write "TEMP update"(TRUE) -> ()
                    n1581 = call "sub vi - GET ALL TEMP v3.vi"("LA01-EN"=w2451, "LA02-EN"=w2451, "LA03-EN"=w2451, "LA04-EN"=w2450, "LA05-EN"=w2450, "Gen Cal Value"=1.0) -> ("LA01 TEMP"=w2449:T19, "LA02 TEMP"=w2447:T19, "LA03 TEMP"=w2446:T19)  [unwired: 4 in, 3 out]
                    n1582 = local write "LAB03 TEMP"(w2446) -> ()
                    n1583 = local write "LAB02 TEMP"(w2447) -> ()
                    n1584 = local write "LAB01 TEMP"(w2449) -> ()
                  }
                }
                n1585 = case shown="True" w2433 {
                  frame False {
                  }
                  frame True {
                    w2443 = TRUE
                    w2444 = FALSE
                    n1586 = local write "TEMP update"(TRUE) -> ()
                    n1587 = call "sub vi - GET ALL TEMP v3.vi"("LA01-EN"=w2444, "LA02-EN"=w2444, "LA03-EN"=w2444, "LA04-EN"=w2443, "LA05-EN"=w2443, "Gen Cal Value"=1.0) -> ("LA04 TEMP"=w2441:T19, "LA05 TEMP"=w2440:T19)  [unwired: 4 in, 4 out]
                    n1588 = local write "LAB04 TEMP"(w2441) -> ()
                    n1589 = local write "LAB05 TEMP"(w2440) -> ()
                  }
                }
              }
              frame #1 {
                n1590 = local read "CAL LAB01"() -> (w2469:T7)
                n1591 = local read "LAB01 TEMP"() -> (w2470:T10)
                n1592 = Unbundle By Name(w2470) -> ("T1 Live"=w2460:dbl, "T1 Neut"=w2459:dbl, "T2 Live"=w2458:dbl, "T2 Neut"=w2457:dbl)  [unwired: 2 out]
                n1593 = Unbundle By Name(w2469) -> ("1 (TL) cal"=w2456:dbl, "1 (TN) cal"=w2455:dbl, "2 (TL) cal"=w2454:dbl, "2 (TN) cal"=w2453:dbl)  [unwired: 6 out]
                n1594 = Multiply(x=w2460, y=w2456) -> (x*y=w2466:dbl)
                n1595 = Multiply(x=w2459, y=w2455) -> (x*y=w2465:dbl)
                n1596 = Multiply(x=w2458, y=w2454) -> (x*y=w2462:dbl)
                n1597 = Multiply(x=w2457, y=w2453) -> (x*y=w2461:dbl)
                n1598 = local read "SIG LAB01-2"() -> (w2464:T2)
                n1599 = local read "SIG LAB01-1"() -> (w2468:T2)
                n1600 = Bundle By Name(cluster=w2468, "Tmp Live"=w2466, "Tmp Neut"=w2465) -> (w2467:T2)
                n1601 = Bundle By Name(cluster=w2464, "Tmp Live"=w2462, "Tmp Neut"=w2461) -> (w2463:T2)
                n1602 = local write "SIG LAB01-1"(w2467) -> ()
                n1603 = local write "SIG LAB01-2"(w2463) -> ()
              }
              frame #2 {
                n1604 = local read "CAL LAB02"() -> (w2487:T8)
                n1605 = local read "LAB02 TEMP"() -> (w2488:T10)
                n1606 = Unbundle By Name(w2488) -> ("T1 Live"=w2478:dbl, "T1 Neut"=w2477:dbl, "T2 Live"=w2476:dbl, "T2 Neut"=w2475:dbl)  [unwired: 2 out]
                n1607 = Unbundle By Name(w2487) -> ("1 (TL) cal"=w2474:dbl, "1 (TN) cal"=w2473:dbl, "2 (TL) cal"=w2472:dbl, "2 (TN) cal"=w2471:dbl)  [unwired: 6 out]
                n1608 = Multiply(x=w2478, y=w2474) -> (x*y=w2484:dbl)
                n1609 = Multiply(x=w2477, y=w2473) -> (x*y=w2483:dbl)
                n1610 = Multiply(x=w2476, y=w2472) -> (x*y=w2480:dbl)
                n1611 = Multiply(x=w2475, y=w2471) -> (x*y=w2479:dbl)
                n1612 = local read "SIG LAB02-2"() -> (w2482:T2)
                n1613 = local read "SIG LAB02-1"() -> (w2486:T2)
                n1614 = Bundle By Name(cluster=w2486, "Tmp Live"=w2484, "Tmp Neut"=w2483) -> (w2485:T2)
                n1615 = Bundle By Name(cluster=w2482, "Tmp Live"=w2480, "Tmp Neut"=w2479) -> (w2481:T2)
                n1616 = local write "SIG LAB02-1"(w2485) -> ()
                n1617 = local write "SIG LAB02-2"(w2481) -> ()
              }
              frame #3 {
                n1618 = local read "CAL LAB03"() -> (w2505:T7)
                n1619 = local read "LAB03 TEMP"() -> (w2506:T10)
                n1620 = Unbundle By Name(w2506) -> ("T1 Live"=w2496:dbl, "T1 Neut"=w2495:dbl, "T2 Live"=w2494:dbl, "T2 Neut"=w2493:dbl)  [unwired: 2 out]
                n1621 = Unbundle By Name(w2505) -> ("1 (TL) cal"=w2492:dbl, "1 (TN) cal"=w2491:dbl, "2 (TL) cal"=w2490:dbl, "2 (TN) cal"=w2489:dbl)  [unwired: 6 out]
                n1622 = Multiply(x=w2496, y=w2492) -> (x*y=w2502:dbl)
                n1623 = Multiply(x=w2495, y=w2491) -> (x*y=w2501:dbl)
                n1624 = Multiply(x=w2494, y=w2490) -> (x*y=w2498:dbl)
                n1625 = Multiply(x=w2493, y=w2489) -> (x*y=w2497:dbl)
                n1626 = local read "SIG LAB03-2"() -> (w2500:T2)
                n1627 = local read "SIG LAB03-1"() -> (w2504:T2)
                n1628 = Bundle By Name(cluster=w2504, "Tmp Live"=w2502, "Tmp Neut"=w2501) -> (w2503:T2)
                n1629 = Bundle By Name(cluster=w2500, "Tmp Live"=w2498, "Tmp Neut"=w2497) -> (w2499:T2)
                n1630 = local write "SIG LAB03-1"(w2503) -> ()
                n1631 = local write "SIG LAB03-2"(w2499) -> ()
              }
              frame #4 {
                n1632 = local read "CAL LAB04"() -> (w2523:T7)
                n1633 = local read "LAB04 TEMP"() -> (w2524:T10)
                n1634 = Unbundle By Name(w2524) -> ("T1 Live"=w2514:dbl, "T1 Neut"=w2513:dbl, "T2 Live"=w2512:dbl, "T2 Neut"=w2511:dbl)  [unwired: 2 out]
                n1635 = Unbundle By Name(w2523) -> ("1 (TL) cal"=w2510:dbl, "1 (TN) cal"=w2509:dbl, "2 (TL) cal"=w2508:dbl, "2 (TN) cal"=w2507:dbl)  [unwired: 6 out]
                n1636 = Multiply(x=w2514, y=w2510) -> (x*y=w2520:dbl)
                n1637 = Multiply(x=w2513, y=w2509) -> (x*y=w2519:dbl)
                n1638 = Multiply(x=w2512, y=w2508) -> (x*y=w2516:dbl)
                n1639 = Multiply(x=w2511, y=w2507) -> (x*y=w2515:dbl)
                n1640 = local read "SIG LAB04-2"() -> (w2518:T2)
                n1641 = local read "SIG LAB04-1"() -> (w2522:T2)
                n1642 = Bundle By Name(cluster=w2522, "Tmp Live"=w2520, "Tmp Neut"=w2519) -> (w2521:T2)
                n1643 = Bundle By Name(cluster=w2518, "Tmp Live"=w2516, "Tmp Neut"=w2515) -> (w2517:T2)
                n1644 = local write "SIG LAB04-1"(w2521) -> ()
                n1645 = local write "SIG LAB04-2"(w2517) -> ()
              }
              frame #5 {
                n1646 = local read "CAL LAB05"() -> (w2541:T7)
                n1647 = local read "LAB05 TEMP"() -> (w2542:T10)
                n1648 = Unbundle By Name(w2542) -> ("T1 Live"=w2532:dbl, "T1 Neut"=w2531:dbl, "T2 Live"=w2530:dbl, "T2 Neut"=w2529:dbl)  [unwired: 2 out]
                n1649 = Unbundle By Name(w2541) -> ("1 (TL) cal"=w2528:dbl, "1 (TN) cal"=w2527:dbl, "2 (TL) cal"=w2526:dbl, "2 (TN) cal"=w2525:dbl)  [unwired: 6 out]
                n1650 = Multiply(x=w2532, y=w2528) -> (x*y=w2538:dbl)
                n1651 = Multiply(x=w2531, y=w2527) -> (x*y=w2537:dbl)
                n1652 = Multiply(x=w2530, y=w2526) -> (x*y=w2534:dbl)
                n1653 = Multiply(x=w2529, y=w2525) -> (x*y=w2533:dbl)
                n1654 = local read "SIG LAB05-2"() -> (w2536:T2)
                n1655 = local read "SIG LAB05-1"() -> (w2540:T2)
                n1656 = Bundle By Name(cluster=w2540, "Tmp Live"=w2538, "Tmp Neut"=w2537) -> (w2539:T2)
                n1657 = Bundle By Name(cluster=w2536, "Tmp Live"=w2534, "Tmp Neut"=w2533) -> (w2535:T2)
                n1658 = local write "SIG LAB05-1"(w2539) -> ()
                n1659 = local write "SIG LAB05-2"(w2535) -> ()
              }
            }
          }
          frame #11 {
            # "get analog values"
            n1660 = local read "on loops"() -> (w2549:dbl)
            n1661 = local read "jig cycle"() -> (w2546:dbl)
            n1662 = Add(x=w2549, y=1) -> (x+y=w2547:dbl)
            n1663 = Equal?(x=w2546, y=1) -> (x = y?=w2544:bool)
            n1664 = Equal?(x=w2546, y=w2547) -> (x = y?=w2545:bool)
            n1665 = Or(x=w2544, y=w2545) -> (x .or. y?=w2543:bool)
            n1666 = case shown="True" w2543 {
              frame False {
              }
              frame True {
                n1667 = call "sub vi - Read Analog All v8.vi"() -> ("Analog loop time"=w2557:dbl, "array GRAPH"=w2556:dynamicdata[], "LAB01"=w2555:T20, "LAB02"=w2554:T21, "LAB03"=w2553:T22, "LAB04"=w2552:T23, "array ERROR"=w2558:errorcluster[], "LAB05"=w2551:T24)  [unwired: 8 in]
                n1668 = stacked-sequence {
                  tunnel: w2558 -> [w2561 _ _ _ _ _]
                  tunnel: w2557 -> [w2560 _ _ _ _ _]
                  tunnel: w2556 -> [w2559 _ _ _ _ _]
                  tunnel: w2555 -> [_ w2606 _ _ _ _]
                  tunnel: w2554 -> [_ _ w2607 _ _ _]
                  tunnel: w2553 -> [_ _ _ w2632 _ _]
                  tunnel: w2552 -> [_ _ _ _ w2655 _]
                  tunnel: w2551 -> [_ _ _ _ _ w2680]
                  frame #0 {
                    n1669 = local write "AI update"(TRUE) -> ()
                    n1670 = Index Array(array=w2559, index=6) -> (element=→"LAB04-1 (GRAPH)":dynamicdata)
                    n1671 = Index Array(array=w2559, index=7) -> (element=→"LAB04-2 (GRAPH)":dynamicdata)
                    n1672 = Index Array(array=w2559, index=9) -> (element=→"LAB05-2 (GRAPH)":dynamicdata)
                    n1673 = Index Array(array=w2559, index=8) -> (element=→"LAB05-1 (GRAPH)":dynamicdata)
                    n1674 = Index Array(array=w2559, index=5) -> (element=→"LAB03-2 (GRAPH)":dynamicdata)
                    n1675 = Index Array(array=w2559, index=0) -> (element=→"LAB01-1 (GRAPH)":dynamicdata)
                    n1676 = Index Array(array=w2559, index=1) -> (element=→"LAB01-2 (GRAPH)":dynamicdata)
                    n1677 = Index Array(array=w2559, index=2) -> (element=→"LAB02-1 (GRAPH)":dynamicdata)
                    n1678 = Index Array(array=w2559, index=3) -> (element=→"LAB02-2 (GRAPH)":dynamicdata)
                    n1679 = Index Array(array=w2559, index=4) -> (element=→"LAB03-1 (GRAPH)":dynamicdata)
                    "AI loop time" <- w2560
                    "Analog Error Array" <- w2561
                  }
                  frame #1 {
                    n1680 = local read "CAL LAB01"() -> (w2605:T7)
                    n1681 = Unbundle By Name(w2606) -> ("LAB01-1 (A)"=w2604:dbl, "LAB01-1 (V)"=w2603:dbl, "LAB01-1 (PF)"=w2602:dbl, "LAB01-2 (A)"=w2601:dbl, "LAB01-2 (V)"=w2600:dbl, "LAB01-2 (PF)"=w2599:dbl)
                    n1682 = Unbundle By Name(w2605) -> ("1  (A) cal"=w2598:dbl, "1 (V) cal"=w2597:dbl, "1 (PF) cal"=w2596:dbl, "2 (A) cal"=w2595:dbl, "2 (V) cal"=w2594:dbl, "2 (PF) cal"=w2593:dbl)  [unwired: 4 out]
                    n1683 = Multiply(x=w2604, y=w2598) -> (x*y=w2591:dbl)
                    n1684 = Multiply(x=w2603, y=w2597) -> (x*y=w2590:dbl)
                    n1685 = Multiply(x=w2602, y=w2596) -> (x*y=w2589:dbl)
                    n1686 = Multiply(x=w2601, y=w2595) -> (x*y=w2585:dbl)
                    n1687 = Multiply(x=w2600, y=w2594) -> (x*y=w2584:dbl)
                    n1688 = Multiply(x=w2599, y=w2593) -> (x*y=w2583:dbl)
                    n1689 = local read "SIG LAB01-1"() -> (w2592:T2)
                    n1690 = local read "SIG LAB01-2"() -> (w2587:T2)
                    n1691 = Bundle By Name(cluster=w2592, "AMPS"=w2591, "VOLTS"=w2590, "PF"=w2589) -> (w2588:T2)
                    n1692 = Bundle By Name(cluster=w2587, "AMPS"=w2585, "VOLTS"=w2584, "PF"=w2583) -> (w2586:T2)
                    n1693 = local write "SIG LAB01-2"(w2586) -> ()
                    n1694 = local write "SIG LAB01-1"(w2588) -> ()
                  }
                  frame #2 {
                    n1695 = local read "CAL LAB02"() -> (w2630:T8)
                    n1696 = Unbundle By Name(w2607) -> ("LAB02-1 (A)"=w2629:dbl, "LAB02-1 (V)"=w2628:dbl, "LAB02-1 (PF)"=w2627:dbl, "LAB02-2 (A)"=w2626:dbl, "LAB02-2 (V)"=w2625:dbl, "LAB02-2 (PF)"=w2624:dbl)
                    n1697 = Unbundle By Name(w2630) -> ("1 (A) cal"=w2623:dbl, "1 (V) cal"=w2622:dbl, "1 (PF) cal"=w2621:dbl, "2 (A) cal"=w2620:dbl, "2 (V) cal"=w2619:dbl, "2 (PF) cal"=w2618:dbl)  [unwired: 4 out]
                    n1698 = Multiply(x=w2629, y=w2623) -> (x*y=w2616:dbl)
                    n1699 = Multiply(x=w2628, y=w2622) -> (x*y=w2615:dbl)
                    n1700 = Multiply(x=w2627, y=w2621) -> (x*y=w2614:dbl)
                    n1701 = Multiply(x=w2626, y=w2620) -> (x*y=w2610:dbl)
                    n1702 = Multiply(x=w2625, y=w2619) -> (x*y=w2609:dbl)
                    n1703 = Multiply(x=w2624, y=w2618) -> (x*y=w2608:dbl)
                    n1704 = local read "SIG LAB02-1"() -> (w2617:T2)
                    n1705 = local read "SIG LAB02-2"() -> (w2612:T2)
                    n1706 = Bundle By Name(cluster=w2617, "AMPS"=w2616, "VOLTS"=w2615, "PF"=w2614) -> (w2613:T2)
                    n1707 = Bundle By Name(cluster=w2612, "AMPS"=w2610, "VOLTS"=w2609, "PF"=w2608) -> (w2611:T2)
                    n1708 = local write "SIG LAB02-2"(w2611) -> ()
                    n1709 = local write "SIG LAB02-1"(w2613) -> ()
                  }
                  frame #3 {
                    n1710 = local read "CAL LAB03"() -> (w2654:T7)
                    n1711 = Unbundle By Name(w2632) -> ("LAB03-1 (A)"=w2653:dbl, "LAB03-1 (V)"=w2652:dbl, "LAB03-1 (PF)"=w2651:dbl, "LAB03-2 (A)"=w2650:dbl, "LAB03-2 (V)"=w2649:dbl, "LAB03-2 (PF)"=w2648:dbl)
                    n1712 = Unbundle By Name(w2654) -> ("1  (A) cal"=w2647:dbl, "1 (V) cal"=w2646:dbl, "1 (PF) cal"=w2645:dbl, "2 (A) cal"=w2644:dbl, "2 (V) cal"=w2643:dbl, "2 (PF) cal"=w2642:dbl)  [unwired: 4 out]
                    n1713 = Multiply(x=w2653, y=w2647) -> (x*y=w2640:dbl)
                    n1714 = Multiply(x=w2652, y=w2646) -> (x*y=w2631:dbl)
                    n1715 = Multiply(x=w2651, y=w2645) -> (x*y=w2639:dbl)
                    n1716 = Multiply(x=w2650, y=w2644) -> (x*y=w2635:dbl)
                    n1717 = Multiply(x=w2649, y=w2643) -> (x*y=w2634:dbl)
                    n1718 = Multiply(x=w2648, y=w2642) -> (x*y=w2633:dbl)
                    n1719 = local read "SIG LAB03-1"() -> (w2641:T2)
                    n1720 = local read "SIG LAB03-2"() -> (w2637:T2)
                    n1721 = Bundle By Name(cluster=w2641, "AMPS"=w2640, "VOLTS"=w2631, "PF"=w2639) -> (w2638:T2)
                    n1722 = Bundle By Name(cluster=w2637, "AMPS"=w2635, "VOLTS"=w2634, "PF"=w2633) -> (w2636:T2)
                    n1723 = local write "SIG LAB03-2"(w2636) -> ()
                    n1724 = local write "SIG LAB03-1"(w2638) -> ()
                  }
                  frame #4 {
                    n1725 = local read "CAL LAB04"() -> (w2678:T7)
                    n1726 = Unbundle By Name(w2655) -> ("LAB04-1 (A)"=w2677:dbl, "LAB04-1 (V)"=w2676:dbl, "LAB04-1 (PF)"=w2675:dbl, "LAB04-2 (A)"=w2674:dbl, "LAB04-2 (V)"=w2673:dbl, "LAB04-2 (PF)"=w2672:dbl)
                    n1727 = Unbundle By Name(w2678) -> ("1  (A) cal"=w2671:dbl, "1 (V) cal"=w2670:dbl, "1 (PF) cal"=w2669:dbl, "2 (A) cal"=w2668:dbl, "2 (V) cal"=w2667:dbl, "2 (PF) cal"=w2666:dbl)  [unwired: 4 out]
                    n1728 = Multiply(x=w2677, y=w2671) -> (x*y=w2664:dbl)
                    n1729 = Multiply(x=w2676, y=w2670) -> (x*y=w2663:dbl)
                    n1730 = Multiply(x=w2675, y=w2669) -> (x*y=w2662:dbl)
                    n1731 = Multiply(x=w2674, y=w2668) -> (x*y=w2658:dbl)
                    n1732 = Multiply(x=w2673, y=w2667) -> (x*y=w2657:dbl)
                    n1733 = Multiply(x=w2672, y=w2666) -> (x*y=w2656:dbl)
                    n1734 = local read "SIG LAB04-1"() -> (w2665:T2)
                    n1735 = local read "SIG LAB04-2"() -> (w2660:T2)
                    n1736 = Bundle By Name(cluster=w2665, "AMPS"=w2664, "VOLTS"=w2663, "PF"=w2662) -> (w2661:T2)
                    n1737 = Bundle By Name(cluster=w2660, "AMPS"=w2658, "VOLTS"=w2657, "PF"=w2656) -> (w2659:T2)
                    n1738 = local write "SIG LAB04-2"(w2659) -> ()
                    n1739 = local write "SIG LAB04-1"(w2661) -> ()
                  }
                  frame #5 {
                    n1740 = local read "CAL LAB05"() -> (w2702:T7)
                    n1741 = Unbundle By Name(w2680) -> ("LAB05-1 (A)"=w2701:dbl, "LAB05-1 (V)"=w2679:dbl, "LAB05-1 (PF)"=w2700:dbl, "LAB05-2 (A)"=w2699:dbl, "LAB05-2 (V)"=w2698:dbl, "LAB05-2 (PF)"=w2697:dbl)
                    n1742 = Unbundle By Name(w2702) -> ("1  (A) cal"=w2696:dbl, "1 (V) cal"=w2695:dbl, "1 (PF) cal"=w2694:dbl, "2 (A) cal"=w2693:dbl, "2 (V) cal"=w2692:dbl, "2 (PF) cal"=w2691:dbl)  [unwired: 4 out]
                    n1743 = Multiply(x=w2701, y=w2696) -> (x*y=w2689:dbl)
                    n1744 = Multiply(x=w2679, y=w2695) -> (x*y=w2688:dbl)
                    n1745 = Multiply(x=w2700, y=w2694) -> (x*y=w2687:dbl)
                    n1746 = Multiply(x=w2699, y=w2693) -> (x*y=w2683:dbl)
                    n1747 = Multiply(x=w2698, y=w2692) -> (x*y=w2682:dbl)
                    n1748 = Multiply(x=w2697, y=w2691) -> (x*y=w2681:dbl)
                    n1749 = local read "SIG LAB05-1"() -> (w2690:T2)
                    n1750 = local read "SIG LAB05-2"() -> (w2685:T2)
                    n1751 = Bundle By Name(cluster=w2690, "AMPS"=w2689, "VOLTS"=w2688, "PF"=w2687) -> (w2686:T2)
                    n1752 = Bundle By Name(cluster=w2685, "AMPS"=w2683, "VOLTS"=w2682, "PF"=w2681) -> (w2684:T2)
                    n1753 = local write "SIG LAB05-2"(w2684) -> ()
                    n1754 = local write "SIG LAB05-1"(w2686) -> ()
                  }
                }
              }
            }
          }
          frame #12 {
            # "save test data to file"
            n1755 = local read "on loops"() -> (w2719:dbl)
            n1756 = local read "jig cycle"() -> (w2716:dbl)
            n1757 = Add(x=w2719, y=2) -> (x+y=w2717:dbl)
            n1758 = Equal?(x=w2716, y=1) -> (x = y?=w2714:bool)
            n1759 = Equal?(x=w2716, y=w2717) -> (x = y?=w2715:bool)
            n1760 = Or(x=w2714, y=w2715) -> (x .or. y?=w2713:bool)
            n1761 = case shown="True" w2713 {
              tunnel: w2712 -> [_ w2730]
              tunnel: w2711 -> [_ w2729]
              tunnel: w2710 -> [_ w2728]
              tunnel: w2709 -> [_ w2727]
              tunnel: w2708 -> [_ w2726]
              tunnel: w2707 -> [_ w2725]
              tunnel: w2706 -> [_ w2724]
              tunnel: w2705 -> [_ w2723]
              tunnel: w2704 -> [_ w2722]
              tunnel: w2703 -> [_ w2721]
              frame False {
              }
              frame True {
                n1762 = stacked-sequence {
                  tunnel: w2730 -> [w2731 _ _ _ _ _ _ _ _ _]
                  tunnel: w2729 -> [_ w2776 _ _ _ _ _ _ _ _]
                  tunnel: w2728 -> [_ _ w2821 _ _ _ _ _ _ _]
                  tunnel: w2727 -> [_ _ _ w2866 _ _ _ _ _ _]
                  tunnel: w2726 -> [_ _ _ _ w2911 _ _ _ _ _]
                  tunnel: w2725 -> [_ _ _ _ _ w2956 _ _ _ _]
                  tunnel: w2724 -> [_ _ _ _ _ _ w3001 _ _ _]
                  tunnel: w2723 -> [_ _ _ _ _ _ _ w3046 _ _]
                  tunnel: w2722 -> [_ _ _ _ _ _ _ _ w3091 _]
                  tunnel: w2721 -> [_ _ _ _ _ _ _ _ _ w3136]
                  frame #0 {
                    # "LAB01-1"
                    n1763 = case shown="True" w2731 {
                      frame False {
                      }
                      frame True {
                        n1764 = local read "DISP LAB01-1"() -> (w2732:T4)
                        n1765 = local read "SIG LAB01-1"() -> (w2733:T2)
                        n1766 = local read "TDMS LAB01-1"() -> (w2775:refnum<k34>)
                        n1767 = Build Array("TEMP Neut") -> (w2741:string[])
                        n1768 = Build Array("CYCLE") -> (w2736:string[])
                        n1769 = Build Array("TEMP Live") -> (w2746:string[])
                        n1770 = Build Array("PF") -> (w2751:string[])
                        n1771 = Build Array("AMPS") -> (w2772:string[])
                        n1772 = Build Array("VOLTS") -> (w2763:string[])
                        n1773 = Unbundle(w2733) -> ("AMPS"=w2771:dbl, "VOLTS"=w2760:dbl, "PF"=w2759:dbl, "Tmp Live"=w2758:dbl, "Tmp Neut"=w2761:dbl)
                        n1774 = Unbundle(w2732) -> ("CYCLE"=w2756:dbl)  [unwired: 2 out]
                        n1775 = Build Array(w2760) -> (w2757:dbl[])
                        n1776 = Build Array(w2759) -> (w2750:dbl[])
                        n1777 = Build Array(w2758) -> (w2745:dbl[])
                        n1778 = Build Array(w2761) -> (w2740:dbl[])
                        n1779 = Build Array(w2771) -> (w2770:dbl[])
                        n1780 = Build Array(w2756) -> (w2735:dbl[])
                        n1781 = TDMS Write(0:w2775, 5:"LAB01-1 TEST VALUES", 7:w2772, 9:w2770) -> (4:w2765:refnum<k34>, 6:w2764:string, 15:w2752:errorcluster)  [unwired: 2 in, 1 out]
                        n1782 = TDMS Write(0:w2765, 5:w2764, 7:w2763, 9:w2757, 11:w2752) -> (4:w2755:refnum<k34>, 6:w2754:string, 15:w2753:errorcluster)  [unwired: 1 in, 1 out]
                        n1783 = TDMS Write(0:w2755, 5:w2754, 7:w2751, 9:w2750, 11:w2753) -> (4:w2749:refnum<k34>, 6:w2748:string, 15:w2747:errorcluster)  [unwired: 1 in, 1 out]
                        n1784 = TDMS Write(0:w2749, 5:w2748, 7:w2746, 9:w2745, 11:w2747) -> (4:w2744:refnum<k34>, 6:w2743:string, 15:w2742:errorcluster)  [unwired: 1 in, 1 out]
                        n1785 = TDMS Write(0:w2744, 5:w2743, 7:w2741, 9:w2740, 11:w2742) -> (4:w2739:refnum<k34>, 6:w2738:string, 15:w2737:errorcluster)  [unwired: 1 in, 1 out]
                        n1786 = TDMS Write(0:w2739, 5:w2738, 7:w2736, 9:w2735, 11:w2737) -> (15:w2734:errorcluster)  [unwired: 1 in, 3 out]
                        n1787 = local write "data file error"(w2734) -> ()
                      }
                    }
                  }
                  frame #1 {
                    # "LAB01-2"
                    n1788 = case shown="True" w2776 {
                      frame False {
                      }
                      frame True {
                        n1789 = local read "DISP LAB01-2"() -> (w2818:T4)
                        n1790 = local read "SIG LAB01-2"() -> (w2819:T2)
                        n1791 = local read "TDMS LAB01-2"() -> (w2820:refnum<k34>)
                        n1792 = Build Array("TEMP Neut") -> (w2784:string[])
                        n1793 = Build Array("CYCLE") -> (w2779:string[])
                        n1794 = Build Array("TEMP Live") -> (w2789:string[])
                        n1795 = Build Array("PF") -> (w2794:string[])
                        n1796 = Build Array("AMPS") -> (w2815:string[])
                        n1797 = Build Array("VOLTS") -> (w2806:string[])
                        n1798 = Unbundle(w2819) -> ("AMPS"=w2814:dbl, "VOLTS"=w2803:dbl, "PF"=w2802:dbl, "Tmp Live"=w2801:dbl, "Tmp Neut"=w2804:dbl)
                        n1799 = Unbundle(w2818) -> ("CYCLE"=w2799:dbl)  [unwired: 2 out]
                        n1800 = Build Array(w2803) -> (w2800:dbl[])
                        n1801 = Build Array(w2802) -> (w2793:dbl[])
                        n1802 = Build Array(w2801) -> (w2788:dbl[])
                        n1803 = Build Array(w2804) -> (w2783:dbl[])
                        n1804 = Build Array(w2814) -> (w2813:dbl[])
                        n1805 = Build Array(w2799) -> (w2778:dbl[])
                        n1806 = TDMS Write(0:w2820, 5:"LAB01-2 TEST VALUES", 7:w2815, 9:w2813) -> (4:w2808:refnum<k34>, 6:w2807:string, 15:w2795:errorcluster)  [unwired: 2 in, 1 out]
                        n1807 = TDMS Write(0:w2808, 5:w2807, 7:w2806, 9:w2800, 11:w2795) -> (4:w2798:refnum<k34>, 6:w2797:string, 15:w2796:errorcluster)  [unwired: 1 in, 1 out]
                        n1808 = TDMS Write(0:w2798, 5:w2797, 7:w2794, 9:w2793, 11:w2796) -> (4:w2792:refnum<k34>, 6:w2791:string, 15:w2790:errorcluster)  [unwired: 1 in, 1 out]
                        n1809 = TDMS Write(0:w2792, 5:w2791, 7:w2789, 9:w2788, 11:w2790) -> (4:w2787:refnum<k34>, 6:w2786:string, 15:w2785:errorcluster)  [unwired: 1 in, 1 out]
                        n1810 = TDMS Write(0:w2787, 5:w2786, 7:w2784, 9:w2783, 11:w2785) -> (4:w2782:refnum<k34>, 6:w2781:string, 15:w2780:errorcluster)  [unwired: 1 in, 1 out]
                        n1811 = TDMS Write(0:w2782, 5:w2781, 7:w2779, 9:w2778, 11:w2780) -> (15:w2777:errorcluster)  [unwired: 1 in, 3 out]
                        n1812 = local write "data file error"(w2777) -> ()
                      }
                    }
                  }
                  frame #2 {
                    # "LAB02-1"
                    n1813 = case shown="True" w2821 {
                      frame False {
                      }
                      frame True {
                        n1814 = local read "DISP LAB02-1"() -> (w2863:T4)
                        n1815 = local read "SIG LAB02-1"() -> (w2864:T2)
                        n1816 = local read "TDMS LAB02-1"() -> (w2865:refnum<k34>)
                        n1817 = Build Array("TEMP Neut") -> (w2829:string[])
                        n1818 = Build Array("CYCLE") -> (w2824:string[])
                        n1819 = Build Array("TEMP Live") -> (w2834:string[])
                        n1820 = Build Array("PF") -> (w2839:string[])
                        n1821 = Build Array("AMPS") -> (w2860:string[])
                        n1822 = Build Array("VOLTS") -> (w2851:string[])
                        n1823 = Unbundle(w2864) -> ("AMPS"=w2859:dbl, "VOLTS"=w2848:dbl, "PF"=w2847:dbl, "Tmp Live"=w2846:dbl, "Tmp Neut"=w2849:dbl)
                        n1824 = Unbundle(w2863) -> ("CYCLE"=w2844:dbl)  [unwired: 2 out]
                        n1825 = Build Array(w2848) -> (w2845:dbl[])
                        n1826 = Build Array(w2847) -> (w2838:dbl[])
                        n1827 = Build Array(w2846) -> (w2833:dbl[])
                        n1828 = Build Array(w2849) -> (w2828:dbl[])
                        n1829 = Build Array(w2859) -> (w2858:dbl[])
                        n1830 = Build Array(w2844) -> (w2823:dbl[])
                        n1831 = TDMS Write(0:w2865, 5:"LAB02-1 TEST VALUES", 7:w2860, 9:w2858) -> (4:w2853:refnum<k34>, 6:w2852:string, 15:w2840:errorcluster)  [unwired: 2 in, 1 out]
                        n1832 = TDMS Write(0:w2853, 5:w2852, 7:w2851, 9:w2845, 11:w2840) -> (4:w2843:refnum<k34>, 6:w2842:string, 15:w2841:errorcluster)  [unwired: 1 in, 1 out]
                        n1833 = TDMS Write(0:w2843, 5:w2842, 7:w2839, 9:w2838, 11:w2841) -> (4:w2837:refnum<k34>, 6:w2836:string, 15:w2835:errorcluster)  [unwired: 1 in, 1 out]
                        n1834 = TDMS Write(0:w2837, 5:w2836, 7:w2834, 9:w2833, 11:w2835) -> (4:w2832:refnum<k34>, 6:w2831:string, 15:w2830:errorcluster)  [unwired: 1 in, 1 out]
                        n1835 = TDMS Write(0:w2832, 5:w2831, 7:w2829, 9:w2828, 11:w2830) -> (4:w2827:refnum<k34>, 6:w2826:string, 15:w2825:errorcluster)  [unwired: 1 in, 1 out]
                        n1836 = TDMS Write(0:w2827, 5:w2826, 7:w2824, 9:w2823, 11:w2825) -> (15:w2822:errorcluster)  [unwired: 1 in, 3 out]
                        n1837 = local write "data file error"(w2822) -> ()
                      }
                    }
                  }
                  frame #3 {
                    # "LAB02-2"
                    n1838 = case shown="True" w2866 {
                      frame False {
                      }
                      frame True {
                        n1839 = local read "DISP LAB02-2"() -> (w2908:T4)
                        n1840 = local read "SIG LAB02-2"() -> (w2909:T2)
                        n1841 = local read "TDMS LAB02-2"() -> (w2910:refnum<k34>)
                        n1842 = Build Array("TEMP Neut") -> (w2874:string[])
                        n1843 = Build Array("CYCLE") -> (w2869:string[])
                        n1844 = Build Array("TEMP Live") -> (w2879:string[])
                        n1845 = Build Array("PF") -> (w2884:string[])
                        n1846 = Build Array("AMPS") -> (w2905:string[])
                        n1847 = Build Array("VOLTS") -> (w2896:string[])
                        n1848 = Unbundle(w2909) -> ("AMPS"=w2904:dbl, "VOLTS"=w2893:dbl, "PF"=w2892:dbl, "Tmp Live"=w2891:dbl, "Tmp Neut"=w2894:dbl)
                        n1849 = Unbundle(w2908) -> ("CYCLE"=w2889:dbl)  [unwired: 2 out]
                        n1850 = Build Array(w2893) -> (w2890:dbl[])
                        n1851 = Build Array(w2892) -> (w2883:dbl[])
                        n1852 = Build Array(w2891) -> (w2878:dbl[])
                        n1853 = Build Array(w2894) -> (w2873:dbl[])
                        n1854 = Build Array(w2904) -> (w2903:dbl[])
                        n1855 = Build Array(w2889) -> (w2868:dbl[])
                        n1856 = TDMS Write(0:w2910, 5:"LAB02-2 TEST VALUES", 7:w2905, 9:w2903) -> (4:w2898:refnum<k34>, 6:w2897:string, 15:w2885:errorcluster)  [unwired: 2 in, 1 out]
                        n1857 = TDMS Write(0:w2898, 5:w2897, 7:w2896, 9:w2890, 11:w2885) -> (4:w2888:refnum<k34>, 6:w2887:string, 15:w2886:errorcluster)  [unwired: 1 in, 1 out]
                        n1858 = TDMS Write(0:w2888, 5:w2887, 7:w2884, 9:w2883, 11:w2886) -> (4:w2882:refnum<k34>, 6:w2881:string, 15:w2880:errorcluster)  [unwired: 1 in, 1 out]
                        n1859 = TDMS Write(0:w2882, 5:w2881, 7:w2879, 9:w2878, 11:w2880) -> (4:w2877:refnum<k34>, 6:w2876:string, 15:w2875:errorcluster)  [unwired: 1 in, 1 out]
                        n1860 = TDMS Write(0:w2877, 5:w2876, 7:w2874, 9:w2873, 11:w2875) -> (4:w2872:refnum<k34>, 6:w2871:string, 15:w2870:errorcluster)  [unwired: 1 in, 1 out]
                        n1861 = TDMS Write(0:w2872, 5:w2871, 7:w2869, 9:w2868, 11:w2870) -> (15:w2867:errorcluster)  [unwired: 1 in, 3 out]
                        n1862 = local write "data file error"(w2867) -> ()
                      }
                    }
                  }
                  frame #4 {
                    # "LAB03-1"
                    n1863 = case shown="True" w2911 {
                      frame False {
                      }
                      frame True {
                        n1864 = local read "DISP LAB03-1"() -> (w2953:T4)
                        n1865 = local read "SIG LAB03-1"() -> (w2954:T2)
                        n1866 = local read "TDMS LAB03-1"() -> (w2955:refnum<k34>)
                        n1867 = Build Array("TEMP Neut") -> (w2919:string[])
                        n1868 = Build Array("CYCLE") -> (w2914:string[])
                        n1869 = Build Array("TEMP Live") -> (w2924:string[])
                        n1870 = Build Array("PF") -> (w2929:string[])
                        n1871 = Build Array("AMPS") -> (w2950:string[])
                        n1872 = Build Array("VOLTS") -> (w2941:string[])
                        n1873 = Unbundle(w2954) -> ("AMPS"=w2949:dbl, "VOLTS"=w2938:dbl, "PF"=w2937:dbl, "Tmp Live"=w2936:dbl, "Tmp Neut"=w2939:dbl)
                        n1874 = Unbundle(w2953) -> ("CYCLE"=w2934:dbl)  [unwired: 2 out]
                        n1875 = Build Array(w2938) -> (w2935:dbl[])
                        n1876 = Build Array(w2937) -> (w2928:dbl[])
                        n1877 = Build Array(w2936) -> (w2923:dbl[])
                        n1878 = Build Array(w2939) -> (w2918:dbl[])
                        n1879 = Build Array(w2949) -> (w2948:dbl[])
                        n1880 = Build Array(w2934) -> (w2913:dbl[])
                        n1881 = TDMS Write(0:w2955, 5:"LAB03-1 TEST VALUES", 7:w2950, 9:w2948) -> (4:w2943:refnum<k34>, 6:w2942:string, 15:w2930:errorcluster)  [unwired: 2 in, 1 out]
                        n1882 = TDMS Write(0:w2943, 5:w2942, 7:w2941, 9:w2935, 11:w2930) -> (4:w2933:refnum<k34>, 6:w2932:string, 15:w2931:errorcluster)  [unwired: 1 in, 1 out]
                        n1883 = TDMS Write(0:w2933, 5:w2932, 7:w2929, 9:w2928, 11:w2931) -> (4:w2927:refnum<k34>, 6:w2926:string, 15:w2925:errorcluster)  [unwired: 1 in, 1 out]
                        n1884 = TDMS Write(0:w2927, 5:w2926, 7:w2924, 9:w2923, 11:w2925) -> (4:w2922:refnum<k34>, 6:w2921:string, 15:w2920:errorcluster)  [unwired: 1 in, 1 out]
                        n1885 = TDMS Write(0:w2922, 5:w2921, 7:w2919, 9:w2918, 11:w2920) -> (4:w2917:refnum<k34>, 6:w2916:string, 15:w2915:errorcluster)  [unwired: 1 in, 1 out]
                        n1886 = TDMS Write(0:w2917, 5:w2916, 7:w2914, 9:w2913, 11:w2915) -> (15:w2912:errorcluster)  [unwired: 1 in, 3 out]
                        n1887 = local write "data file error"(w2912) -> ()
                      }
                    }
                  }
                  frame #5 {
                    # "LAB03-2"
                    n1888 = case shown="True" w2956 {
                      frame False {
                      }
                      frame True {
                        n1889 = local read "DISP LAB03-2"() -> (w2998:T4)
                        n1890 = local read "SIG LAB03-2"() -> (w2999:T2)
                        n1891 = local read "TDMS LAB03-2"() -> (w3000:refnum<k34>)
                        n1892 = Build Array("TEMP Neut") -> (w2964:string[])
                        n1893 = Build Array("CYCLE") -> (w2959:string[])
                        n1894 = Build Array("TEMP Live") -> (w2969:string[])
                        n1895 = Build Array("PF") -> (w2974:string[])
                        n1896 = Build Array("AMPS") -> (w2995:string[])
                        n1897 = Build Array("VOLTS") -> (w2986:string[])
                        n1898 = Unbundle(w2999) -> ("AMPS"=w2994:dbl, "VOLTS"=w2983:dbl, "PF"=w2982:dbl, "Tmp Live"=w2981:dbl, "Tmp Neut"=w2984:dbl)
                        n1899 = Unbundle(w2998) -> ("CYCLE"=w2979:dbl)  [unwired: 2 out]
                        n1900 = Build Array(w2983) -> (w2980:dbl[])
                        n1901 = Build Array(w2982) -> (w2973:dbl[])
                        n1902 = Build Array(w2981) -> (w2968:dbl[])
                        n1903 = Build Array(w2984) -> (w2963:dbl[])
                        n1904 = Build Array(w2994) -> (w2993:dbl[])
                        n1905 = Build Array(w2979) -> (w2958:dbl[])
                        n1906 = TDMS Write(0:w3000, 5:"LAB03-2 TEST VALUES", 7:w2995, 9:w2993) -> (4:w2988:refnum<k34>, 6:w2987:string, 15:w2975:errorcluster)  [unwired: 2 in, 1 out]
                        n1907 = TDMS Write(0:w2988, 5:w2987, 7:w2986, 9:w2980, 11:w2975) -> (4:w2978:refnum<k34>, 6:w2977:string, 15:w2976:errorcluster)  [unwired: 1 in, 1 out]
                        n1908 = TDMS Write(0:w2978, 5:w2977, 7:w2974, 9:w2973, 11:w2976) -> (4:w2972:refnum<k34>, 6:w2971:string, 15:w2970:errorcluster)  [unwired: 1 in, 1 out]
                        n1909 = TDMS Write(0:w2972, 5:w2971, 7:w2969, 9:w2968, 11:w2970) -> (4:w2967:refnum<k34>, 6:w2966:string, 15:w2965:errorcluster)  [unwired: 1 in, 1 out]
                        n1910 = TDMS Write(0:w2967, 5:w2966, 7:w2964, 9:w2963, 11:w2965) -> (4:w2962:refnum<k34>, 6:w2961:string, 15:w2960:errorcluster)  [unwired: 1 in, 1 out]
                        n1911 = TDMS Write(0:w2962, 5:w2961, 7:w2959, 9:w2958, 11:w2960) -> (15:w2957:errorcluster)  [unwired: 1 in, 3 out]
                        n1912 = local write "data file error"(w2957) -> ()
                      }
                    }
                  }
                  frame #6 {
                    # "LAB04-1"
                    n1913 = case shown="True" w3001 {
                      frame False {
                      }
                      frame True {
                        n1914 = local read "DISP LAB04-1"() -> (w3043:T4)
                        n1915 = local read "SIG LAB04-1"() -> (w3044:T2)
                        n1916 = local read "TDMS LAB04-1"() -> (w3045:refnum<k34>)
                        n1917 = Build Array("TEMP Neut") -> (w3009:string[])
                        n1918 = Build Array("CYCLE") -> (w3004:string[])
                        n1919 = Build Array("TEMP Live") -> (w3014:string[])
                        n1920 = Build Array("PF") -> (w3019:string[])
                        n1921 = Build Array("AMPS") -> (w3040:string[])
                        n1922 = Build Array("VOLTS") -> (w3031:string[])
                        n1923 = Unbundle(w3044) -> ("AMPS"=w3039:dbl, "VOLTS"=w3028:dbl, "PF"=w3027:dbl, "Tmp Live"=w3026:dbl, "Tmp Neut"=w3029:dbl)
                        n1924 = Unbundle(w3043) -> ("CYCLE"=w3024:dbl)  [unwired: 2 out]
                        n1925 = Build Array(w3028) -> (w3025:dbl[])
                        n1926 = Build Array(w3027) -> (w3018:dbl[])
                        n1927 = Build Array(w3026) -> (w3013:dbl[])
                        n1928 = Build Array(w3029) -> (w3008:dbl[])
                        n1929 = Build Array(w3039) -> (w3038:dbl[])
                        n1930 = Build Array(w3024) -> (w3003:dbl[])
                        n1931 = TDMS Write(0:w3045, 5:"LAB04-1 TEST VALUES", 7:w3040, 9:w3038) -> (4:w3033:refnum<k34>, 6:w3032:string, 15:w3020:errorcluster)  [unwired: 2 in, 1 out]
                        n1932 = TDMS Write(0:w3033, 5:w3032, 7:w3031, 9:w3025, 11:w3020) -> (4:w3023:refnum<k34>, 6:w3022:string, 15:w3021:errorcluster)  [unwired: 1 in, 1 out]
                        n1933 = TDMS Write(0:w3023, 5:w3022, 7:w3019, 9:w3018, 11:w3021) -> (4:w3017:refnum<k34>, 6:w3016:string, 15:w3015:errorcluster)  [unwired: 1 in, 1 out]
                        n1934 = TDMS Write(0:w3017, 5:w3016, 7:w3014, 9:w3013, 11:w3015) -> (4:w3012:refnum<k34>, 6:w3011:string, 15:w3010:errorcluster)  [unwired: 1 in, 1 out]
                        n1935 = TDMS Write(0:w3012, 5:w3011, 7:w3009, 9:w3008, 11:w3010) -> (4:w3007:refnum<k34>, 6:w3006:string, 15:w3005:errorcluster)  [unwired: 1 in, 1 out]
                        n1936 = TDMS Write(0:w3007, 5:w3006, 7:w3004, 9:w3003, 11:w3005) -> (15:w3002:errorcluster)  [unwired: 1 in, 3 out]
                        n1937 = local write "data file error"(w3002) -> ()
                      }
                    }
                  }
                  frame #7 {
                    # "LAB04-2"
                    n1938 = case shown="True" w3046 {
                      frame False {
                      }
                      frame True {
                        n1939 = local read "DISP LAB04-2"() -> (w3088:T4)
                        n1940 = local read "SIG LAB04-2"() -> (w3089:T2)
                        n1941 = local read "TDMS LAB04-2"() -> (w3090:refnum<k34>)
                        n1942 = Build Array("TEMP Neut") -> (w3054:string[])
                        n1943 = Build Array("CYCLE") -> (w3049:string[])
                        n1944 = Build Array("TEMP Live") -> (w3059:string[])
                        n1945 = Build Array("PF") -> (w3064:string[])
                        n1946 = Build Array("AMPS") -> (w3085:string[])
                        n1947 = Build Array("VOLTS") -> (w3076:string[])
                        n1948 = Unbundle(w3089) -> ("AMPS"=w3084:dbl, "VOLTS"=w3073:dbl, "PF"=w3072:dbl, "Tmp Live"=w3071:dbl, "Tmp Neut"=w3074:dbl)
                        n1949 = Unbundle(w3088) -> ("CYCLE"=w3069:dbl)  [unwired: 2 out]
                        n1950 = Build Array(w3073) -> (w3070:dbl[])
                        n1951 = Build Array(w3072) -> (w3063:dbl[])
                        n1952 = Build Array(w3071) -> (w3058:dbl[])
                        n1953 = Build Array(w3074) -> (w3053:dbl[])
                        n1954 = Build Array(w3084) -> (w3083:dbl[])
                        n1955 = Build Array(w3069) -> (w3048:dbl[])
                        n1956 = TDMS Write(0:w3090, 5:"LAB04-2 TEST VALUES", 7:w3085, 9:w3083) -> (4:w3078:refnum<k34>, 6:w3077:string, 15:w3065:errorcluster)  [unwired: 2 in, 1 out]
                        n1957 = TDMS Write(0:w3078, 5:w3077, 7:w3076, 9:w3070, 11:w3065) -> (4:w3068:refnum<k34>, 6:w3067:string, 15:w3066:errorcluster)  [unwired: 1 in, 1 out]
                        n1958 = TDMS Write(0:w3068, 5:w3067, 7:w3064, 9:w3063, 11:w3066) -> (4:w3062:refnum<k34>, 6:w3061:string, 15:w3060:errorcluster)  [unwired: 1 in, 1 out]
                        n1959 = TDMS Write(0:w3062, 5:w3061, 7:w3059, 9:w3058, 11:w3060) -> (4:w3057:refnum<k34>, 6:w3056:string, 15:w3055:errorcluster)  [unwired: 1 in, 1 out]
                        n1960 = TDMS Write(0:w3057, 5:w3056, 7:w3054, 9:w3053, 11:w3055) -> (4:w3052:refnum<k34>, 6:w3051:string, 15:w3050:errorcluster)  [unwired: 1 in, 1 out]
                        n1961 = TDMS Write(0:w3052, 5:w3051, 7:w3049, 9:w3048, 11:w3050) -> (15:w3047:errorcluster)  [unwired: 1 in, 3 out]
                        n1962 = local write "data file error"(w3047) -> ()
                      }
                    }
                  }
                  frame #8 {
                    # "LAB05-1"
                    n1963 = case shown="True" w3091 {
                      frame False {
                      }
                      frame True {
                        n1964 = local read "DISP LAB05-1"() -> (w3133:T4)
                        n1965 = local read "SIG LAB05-1"() -> (w3134:T2)
                        n1966 = local read "TDMS LAB05-1"() -> (w3135:refnum<k34>)
                        n1967 = Build Array("TEMP Neut") -> (w3099:string[])
                        n1968 = Build Array("CYCLE") -> (w3094:string[])
                        n1969 = Build Array("TEMP Live") -> (w3104:string[])
                        n1970 = Build Array("PF") -> (w3109:string[])
                        n1971 = Build Array("AMPS") -> (w3130:string[])
                        n1972 = Build Array("VOLTS") -> (w3121:string[])
                        n1973 = Unbundle(w3134) -> ("AMPS"=w3129:dbl, "VOLTS"=w3118:dbl, "PF"=w3117:dbl, "Tmp Live"=w3116:dbl, "Tmp Neut"=w3119:dbl)
                        n1974 = Unbundle(w3133) -> ("CYCLE"=w3114:dbl)  [unwired: 2 out]
                        n1975 = Build Array(w3118) -> (w3115:dbl[])
                        n1976 = Build Array(w3117) -> (w3108:dbl[])
                        n1977 = Build Array(w3116) -> (w3103:dbl[])
                        n1978 = Build Array(w3119) -> (w3098:dbl[])
                        n1979 = Build Array(w3129) -> (w3128:dbl[])
                        n1980 = Build Array(w3114) -> (w3093:dbl[])
                        n1981 = TDMS Write(0:w3135, 5:"LAB05-1 TEST VALUES", 7:w3130, 9:w3128) -> (4:w3123:refnum<k34>, 6:w3122:string, 15:w3110:errorcluster)  [unwired: 2 in, 1 out]
                        n1982 = TDMS Write(0:w3123, 5:w3122, 7:w3121, 9:w3115, 11:w3110) -> (4:w3113:refnum<k34>, 6:w3112:string, 15:w3111:errorcluster)  [unwired: 1 in, 1 out]
                        n1983 = TDMS Write(0:w3113, 5:w3112, 7:w3109, 9:w3108, 11:w3111) -> (4:w3107:refnum<k34>, 6:w3106:string, 15:w3105:errorcluster)  [unwired: 1 in, 1 out]
                        n1984 = TDMS Write(0:w3107, 5:w3106, 7:w3104, 9:w3103, 11:w3105) -> (4:w3102:refnum<k34>, 6:w3101:string, 15:w3100:errorcluster)  [unwired: 1 in, 1 out]
                        n1985 = TDMS Write(0:w3102, 5:w3101, 7:w3099, 9:w3098, 11:w3100) -> (4:w3097:refnum<k34>, 6:w3096:string, 15:w3095:errorcluster)  [unwired: 1 in, 1 out]
                        n1986 = TDMS Write(0:w3097, 5:w3096, 7:w3094, 9:w3093, 11:w3095) -> (15:w3092:errorcluster)  [unwired: 1 in, 3 out]
                        n1987 = local write "data file error"(w3092) -> ()
                      }
                    }
                  }
                  frame #9 {
                    # "LAB05-2"
                    n1988 = case shown="True" w3136 {
                      frame False {
                      }
                      frame True {
                        n1989 = local read "DISP LAB05-2"() -> (w3178:T4)
                        n1990 = local read "SIG LAB05-2"() -> (w3179:T2)
                        n1991 = local read "TDMS LAB05-2"() -> (w3180:refnum<k34>)
                        n1992 = Build Array("TEMP Neut") -> (w3144:string[])
                        n1993 = Build Array("CYCLE") -> (w3139:string[])
                        n1994 = Build Array("TEMP Live") -> (w3149:string[])
                        n1995 = Build Array("PF") -> (w3154:string[])
                        n1996 = Build Array("AMPS") -> (w3175:string[])
                        n1997 = Build Array("VOLTS") -> (w3166:string[])
                        n1998 = Unbundle(w3179) -> ("AMPS"=w3174:dbl, "VOLTS"=w3163:dbl, "PF"=w3162:dbl, "Tmp Live"=w3161:dbl, "Tmp Neut"=w3164:dbl)
                        n1999 = Unbundle(w3178) -> ("CYCLE"=w3159:dbl)  [unwired: 2 out]
                        n2000 = Build Array(w3163) -> (w3160:dbl[])
                        n2001 = Build Array(w3162) -> (w3153:dbl[])
                        n2002 = Build Array(w3161) -> (w3148:dbl[])
                        n2003 = Build Array(w3164) -> (w3143:dbl[])
                        n2004 = Build Array(w3174) -> (w3173:dbl[])
                        n2005 = Build Array(w3159) -> (w3138:dbl[])
                        n2006 = TDMS Write(0:w3180, 5:"LAB05-2 TEST VALUES", 7:w3175, 9:w3173) -> (4:w3168:refnum<k34>, 6:w3167:string, 15:w3155:errorcluster)  [unwired: 2 in, 1 out]
                        n2007 = TDMS Write(0:w3168, 5:w3167, 7:w3166, 9:w3160, 11:w3155) -> (4:w3158:refnum<k34>, 6:w3157:string, 15:w3156:errorcluster)  [unwired: 1 in, 1 out]
                        n2008 = TDMS Write(0:w3158, 5:w3157, 7:w3154, 9:w3153, 11:w3156) -> (4:w3152:refnum<k34>, 6:w3151:string, 15:w3150:errorcluster)  [unwired: 1 in, 1 out]
                        n2009 = TDMS Write(0:w3152, 5:w3151, 7:w3149, 9:w3148, 11:w3150) -> (4:w3147:refnum<k34>, 6:w3146:string, 15:w3145:errorcluster)  [unwired: 1 in, 1 out]
                        n2010 = TDMS Write(0:w3147, 5:w3146, 7:w3144, 9:w3143, 11:w3145) -> (4:w3142:refnum<k34>, 6:w3141:string, 15:w3140:errorcluster)  [unwired: 1 in, 1 out]
                        n2011 = TDMS Write(0:w3142, 5:w3141, 7:w3139, 9:w3138, 11:w3140) -> (15:w3137:errorcluster)  [unwired: 1 in, 3 out]
                        n2012 = local write "data file error"(w3137) -> ()
                      }
                    }
                  }
                }
              }
            }
          }
          frame #13 {
            # "check for amps fail"
            # "check for cycle test & temperature rise fail conditions"
            n2013 = local read "on loops"() -> (w3206:dbl)
            n2014 = local read "jig cycle"() -> (w3203:dbl)
            n2015 = local read "jig cycle"() -> (w3208:dbl)
            n2016 = Add(x=w3206, y=3.0) -> (x+y=w3204:dbl)
            n2017 = Equal?(x=w3203, y=w3204) -> (x = y?=w3199:bool)
            n2018 = Equal?(x=w3208, y=1.0) -> (x = y?=w3201:bool)
            n2019 = stacked-sequence {
              tunnel: w3202 -> [w3211 _ _ _ _ _ _ _ _ _]
              tunnel: w3201 -> [w3212 w3232 w3252 w3272 w3292 w3312 w3332 w3352 w3372 w3392]
              tunnel: w3200 -> [w3209 _ _ _ _ _ _ _ _ _]
              tunnel: w3199 -> [w3210 w3231 w3251 w3271 w3291 w3311 w3331 w3351 w3371 w3391]
              tunnel: w3198 -> [_ w3230 _ _ _ _ _ _ _ _]
              tunnel: w3197 -> [_ w3229 _ _ _ _ _ _ _ _]
              tunnel: w3196 -> [_ _ w3250 _ _ _ _ _ _ _]
              tunnel: w3195 -> [_ _ w3249 _ _ _ _ _ _ _]
              tunnel: w3194 -> [_ _ _ w3270 _ _ _ _ _ _]
              tunnel: w3193 -> [_ _ _ w3269 _ _ _ _ _ _]
              tunnel: w3192 -> [_ _ _ _ w3290 _ _ _ _ _]
              tunnel: w3191 -> [_ _ _ _ w3289 _ _ _ _ _]
              tunnel: w3190 -> [_ _ _ _ _ w3310 _ _ _ _]
              tunnel: w3189 -> [_ _ _ _ _ w3309 _ _ _ _]
              tunnel: w3188 -> [_ _ _ _ _ _ w3330 _ _ _]
              tunnel: w3187 -> [_ _ _ _ _ _ w3329 _ _ _]
              tunnel: w3186 -> [_ _ _ _ _ _ _ w3350 _ _]
              tunnel: w3185 -> [_ _ _ _ _ _ _ w3349 _ _]
              tunnel: w3184 -> [_ _ _ _ _ _ _ _ w3370 _]
              tunnel: w3183 -> [_ _ _ _ _ _ _ _ w3369 _]
              tunnel: w3182 -> [_ _ _ _ _ _ _ _ _ w3390]
              tunnel: w3181 -> [_ _ _ _ _ _ _ _ _ w3389]
              frame #0 {
                # "LAB01-1"
                n2020 = case shown="True" w3209 {
                  tunnel: w3212 -> [_ w3225]
                  tunnel: w3211 -> [_ w3222]
                  tunnel: w3210 -> [_ w3221]
                  frame False {
                  }
                  frame True {
                    n2021 = local read "TEMP START LAB01-1"() -> (w3227:cluster{"TL":dbl, "TN":dbl})
                    n2022 = local read "RESULT LAB01-1"() -> (w3215:bool)
                    n2023 = local read "FAIL LAB01-1"() -> (w3218:cluster{"LO":dbl, "HI":dbl})
                    n2024 = local read "TDMS LAB01-1"() -> (w3226:refnum<k34>)
                    n2025 = local read "SET LAB01-1"() -> (w3223:T5)
                    n2026 = local read "DISP LAB01-1"() -> (w3224:T4)
                    n2027 = local read "SIG LAB01-1"() -> (w3228:T2)
                    n2028 = Bundle("FAIL LAB01-1"=w3218, "SIG LAB01-1"=w3228, "TEMP START LAB01-1"=w3227, "DISP LAB01-1"=w3224, "SET LAB01-1"=w3223, "TDMS LAB01-1"=w3226) -> (w3213:T25)  [unwired: 1 in]
                    n2029 = call "sub vi - cycle&temp fail v6.vi"("Amps Lo?"=w3225, "Input Cluster"=w3213, "SELECT"=w3222, "Amps Hi?"=w3221, "Result In"=w3215) -> ("(FAIL) out"=w3217:cluster{"FAIL LO":dbl, "FAIL HI":dbl}, "(DISP) out"=w3220:T4, "T-RISE"=w3214:cluster{"T-RISE (L)":dbl, "T-RISE (N)":dbl}, "Result Out"=w3216:bool, "file error"=w3219:errorcluster)  [unwired: 10 in]
                    n2030 = local write "TEMP RISE LAB01-1"(w3214) -> ()
                    n2031 = local write "FAIL LAB01-1"(w3217) -> ()
                    n2032 = local write "DISP LAB01-1"(w3220) -> ()
                    n2033 = local write "RESULT LAB01-1"(w3216) -> ()
                    n2034 = local write "data file error"(w3219) -> ()
                  }
                }
              }
              frame #1 {
                # "LAB01-2"
                n2035 = case shown="True" w3230 {
                  tunnel: w3232 -> [_ w3245]
                  tunnel: w3229 -> [_ w3242]
                  tunnel: w3231 -> [_ w3241]
                  frame False {
                  }
                  frame True {
                    n2036 = local read "TEMP START LAB01-2"() -> (w3247:cluster{"TL":dbl, "TN":dbl})
                    n2037 = local read "FAIL LAB01-2"() -> (w3238:cluster{"LO":dbl, "HI":dbl})
                    n2038 = local read "TDMS LAB01-2"() -> (w3246:refnum<k34>)
                    n2039 = local read "SET LAB01-2"() -> (w3243:T5)
                    n2040 = local read "DISP LAB01-2"() -> (w3244:T4)
                    n2041 = local read "RESULT LAB01-2"() -> (w3235:bool)
                    n2042 = local read "SIG LAB01-2"() -> (w3248:T2)
                    n2043 = Bundle("FAIL LAB01-2"=w3238, "SIG LAB01-2"=w3248, "TEMP START LAB01-2"=w3247, "DISP LAB01-2"=w3244, "SET LAB01-2"=w3243, "TDMS LAB01-2"=w3246) -> (w3233:T26)  [unwired: 1 in]
                    n2044 = call "sub vi - cycle&temp fail v6.vi"("Amps Lo?"=w3245, "Input Cluster"=w3233, "SELECT"=w3242, "Amps Hi?"=w3241, "Result In"=w3235) -> ("(FAIL) out"=w3237:cluster{"FAIL LO":dbl, "FAIL HI":dbl}, "(DISP) out"=w3240:T4, "T-RISE"=w3234:cluster{"T-RISE (L)":dbl, "T-RISE (N)":dbl}, "Result Out"=w3236:bool, "file error"=w3239:errorcluster)  [unwired: 10 in]
                    n2045 = local write "TEMP RISE LAB01-2"(w3234) -> ()
                    n2046 = local write "FAIL LAB01-2"(w3237) -> ()
                    n2047 = local write "DISP LAB01-2"(w3240) -> ()
                    n2048 = local write "RESULT LAB01-2"(w3236) -> ()
                    n2049 = local write "data file error"(w3239) -> ()
                  }
                }
              }
              frame #2 {
                # "LAB02-1"
                n2050 = case shown="True" w3250 {
                  tunnel: w3252 -> [_ w3265]
                  tunnel: w3249 -> [_ w3262]
                  tunnel: w3251 -> [_ w3261]
                  frame False {
                  }
                  frame True {
                    n2051 = local read "TEMP START LAB02-1"() -> (w3267:cluster{"TL":dbl, "TN":dbl})
                    n2052 = local read "FAIL LAB02-1"() -> (w3258:cluster{"LO":dbl, "HI":dbl})
                    n2053 = local read "TDMS LAB02-1"() -> (w3266:refnum<k34>)
                    n2054 = local read "SET LAB02-1"() -> (w3263:T5)
                    n2055 = local read "DISP LAB02-1"() -> (w3264:T4)
                    n2056 = local read "SIG LAB02-1"() -> (w3268:T2)
                    n2057 = local read "RESULT LAB02-1"() -> (w3255:bool)
                    n2058 = Bundle("FAIL LAB02-1"=w3258, "SIG LAB02-1"=w3268, "TEMP START LAB02-1"=w3267, "DISP LAB02-1"=w3264, "SET LAB02-1"=w3263, "TDMS LAB02-1"=w3266) -> (w3253:T27)  [unwired: 1 in]
                    n2059 = call "sub vi - cycle&temp fail v6.vi"("Amps Lo?"=w3265, "Input Cluster"=w3253, "SELECT"=w3262, "Amps Hi?"=w3261, "Result In"=w3255) -> ("(FAIL) out"=w3257:cluster{"FAIL LO":dbl, "FAIL HI":dbl}, "(DISP) out"=w3260:T4, "T-RISE"=w3254:cluster{"T-RISE (L)":dbl, "T-RISE (N)":dbl}, "Result Out"=w3256:bool, "file error"=w3259:errorcluster)  [unwired: 10 in]
                    n2060 = local write "TEMP RISE LAB02-1"(w3254) -> ()
                    n2061 = local write "FAIL LAB02-1"(w3257) -> ()
                    n2062 = local write "DISP LAB02-1"(w3260) -> ()
                    n2063 = local write "RESULT LAB02-1"(w3256) -> ()
                    n2064 = local write "data file error"(w3259) -> ()
                  }
                }
              }
              frame #3 {
                # "LAB02-2"
                n2065 = case shown="True" w3270 {
                  tunnel: w3272 -> [_ w3285]
                  tunnel: w3269 -> [_ w3282]
                  tunnel: w3271 -> [_ w3281]
                  frame False {
                  }
                  frame True {
                    n2066 = local read "TEMP START LAB02-2"() -> (w3287:cluster{"TL":dbl, "TN":dbl})
                    n2067 = local read "FAIL LAB02-2"() -> (w3278:cluster{"LO":dbl, "HI":dbl})
                    n2068 = local read "TDMS LAB02-2"() -> (w3286:refnum<k34>)
                    n2069 = local read "SET LAB02-2"() -> (w3283:T5)
                    n2070 = local read "DISP LAB02-2"() -> (w3284:T4)
                    n2071 = local read "SIG LAB02-2"() -> (w3288:T2)
                    n2072 = local read "RESULT LAB02-2"() -> (w3275:bool)
                    n2073 = Bundle("FAIL LAB02-2"=w3278, "SIG LAB02-2"=w3288, "TEMP START LAB02-2"=w3287, "DISP LAB02-2"=w3284, "SET LAB02-2"=w3283, "TDMS LAB02-2"=w3286) -> (w3273:T28)  [unwired: 1 in]
                    n2074 = call "sub vi - cycle&temp fail v6.vi"("Amps Lo?"=w3285, "Input Cluster"=w3273, "SELECT"=w3282, "Amps Hi?"=w3281, "Result In"=w3275) -> ("(FAIL) out"=w3277:cluster{"FAIL LO":dbl, "FAIL HI":dbl}, "(DISP) out"=w3280:T4, "T-RISE"=w3274:cluster{"T-RISE (L)":dbl, "T-RISE (N)":dbl}, "Result Out"=w3276:bool, "file error"=w3279:errorcluster)  [unwired: 10 in]
                    n2075 = local write "TEMP RISE LAB02-2"(w3274) -> ()
                    n2076 = local write "FAIL LAB02-2"(w3277) -> ()
                    n2077 = local write "DISP LAB02-2"(w3280) -> ()
                    n2078 = local write "RESULT LAB02-2"(w3276) -> ()
                    n2079 = local write "data file error"(w3279) -> ()
                  }
                }
              }
              frame #4 {
                # "LAB03-1"
                n2080 = case shown="True" w3290 {
                  tunnel: w3292 -> [_ w3305]
                  tunnel: w3289 -> [_ w3302]
                  tunnel: w3291 -> [_ w3301]
                  frame False {
                  }
                  frame True {
                    n2081 = local read "TEMP START LAB03-1"() -> (w3307:cluster{"TL":dbl, "TN":dbl})
                    n2082 = local read "FAIL LAB03-1"() -> (w3298:cluster{"LO":dbl, "HI":dbl})
                    n2083 = local read "TDMS LAB03-1"() -> (w3306:refnum<k34>)
                    n2084 = local read "SET LAB03-1"() -> (w3303:T5)
                    n2085 = local read "DISP LAB03-1"() -> (w3304:T4)
                    n2086 = local read "SIG LAB03-1"() -> (w3308:T2)
                    n2087 = local read "RESULT LAB03-1"() -> (w3295:bool)
                    n2088 = Bundle("FAIL LAB03-1"=w3298, "SIG LAB03-1"=w3308, "TEMP START LAB03-1"=w3307, "DISP LAB03-1"=w3304, "SET LAB03-1"=w3303, "TDMS LAB03-1"=w3306) -> (w3293:T29)  [unwired: 1 in]
                    n2089 = call "sub vi - cycle&temp fail v6.vi"("Amps Lo?"=w3305, "Input Cluster"=w3293, "SELECT"=w3302, "Amps Hi?"=w3301, "Result In"=w3295) -> ("(FAIL) out"=w3297:cluster{"FAIL LO":dbl, "FAIL HI":dbl}, "(DISP) out"=w3300:T4, "T-RISE"=w3294:cluster{"T-RISE (L)":dbl, "T-RISE (N)":dbl}, "Result Out"=w3296:bool, "file error"=w3299:errorcluster)  [unwired: 10 in]
                    n2090 = local write "TEMP RISE LAB03-1"(w3294) -> ()
                    n2091 = local write "FAIL LAB03-1"(w3297) -> ()
                    n2092 = local write "DISP LAB03-1"(w3300) -> ()
                    n2093 = local write "RESULT LAB03-1"(w3296) -> ()
                    n2094 = local write "data file error"(w3299) -> ()
                  }
                }
              }
              frame #5 {
                # "LAB03-2"
                n2095 = case shown="True" w3310 {
                  tunnel: w3312 -> [_ w3325]
                  tunnel: w3309 -> [_ w3322]
                  tunnel: w3311 -> [_ w3321]
                  frame False {
                  }
                  frame True {
                    n2096 = local read "TEMP START LAB03-2"() -> (w3327:cluster{"TL":dbl, "TN":dbl})
                    n2097 = local read "FAIL LAB03-2"() -> (w3318:cluster{"LO":dbl, "HI":dbl})
                    n2098 = local read "TDMS LAB03-2"() -> (w3326:refnum<k34>)
                    n2099 = local read "SET LAB03-2"() -> (w3323:T5)
                    n2100 = local read "DISP LAB03-2"() -> (w3324:T4)
                    n2101 = local read "RESULT LAB03-2"() -> (w3315:bool)
                    n2102 = local read "SIG LAB03-2"() -> (w3328:T2)
                    n2103 = Bundle("FAIL LAB03-2"=w3318, "SIG LAB03-2"=w3328, "TEMP START LAB03-2"=w3327, "DISP LAB03-2"=w3324, "SET LAB03-2"=w3323, "TDMS LAB03-2"=w3326) -> (w3313:T30)  [unwired: 1 in]
                    n2104 = call "sub vi - cycle&temp fail v6.vi"("Amps Lo?"=w3325, "Input Cluster"=w3313, "SELECT"=w3322, "Amps Hi?"=w3321, "Result In"=w3315) -> ("(FAIL) out"=w3317:cluster{"FAIL LO":dbl, "FAIL HI":dbl}, "(DISP) out"=w3320:T4, "T-RISE"=w3314:cluster{"T-RISE (L)":dbl, "T-RISE (N)":dbl}, "Result Out"=w3316:bool, "file error"=w3319:errorcluster)  [unwired: 10 in]
                    n2105 = local write "FAIL LAB03-2"(w3317) -> ()
                    n2106 = local write "TEMP RISE LAB03-2"(w3314) -> ()
                    n2107 = local write "DISP LAB03-2"(w3320) -> ()
                    n2108 = local write "RESULT LAB03-2"(w3316) -> ()
                    n2109 = local write "data file error"(w3319) -> ()
                  }
                }
              }
              frame #6 {
                # "LAB04-1"
                n2110 = case shown="True" w3330 {
                  tunnel: w3332 -> [_ w3345]
                  tunnel: w3329 -> [_ w3342]
                  tunnel: w3331 -> [_ w3341]
                  frame False {
                  }
                  frame True {
                    n2111 = local read "TEMP START LAB04-1"() -> (w3347:cluster{"TL":dbl, "TN":dbl})
                    n2112 = local read "FAIL LAB04-1"() -> (w3338:cluster{"LO":dbl, "HI":dbl})
                    n2113 = local read "TDMS LAB04-1"() -> (w3346:refnum<k34>)
                    n2114 = local read "SET LAB04-1"() -> (w3343:T5)
                    n2115 = local read "DISP LAB04-1"() -> (w3344:T4)
                    n2116 = local read "SIG LAB04-1"() -> (w3348:T2)
                    n2117 = local read "RESULT LAB04-1"() -> (w3335:bool)
                    n2118 = Bundle("FAIL LAB04-1"=w3338, "SIG LAB04-1"=w3348, "TEMP START LAB04-1"=w3347, "DISP LAB04-1"=w3344, "SET LAB04-1"=w3343, "TDMS LAB04-1"=w3346) -> (w3333:T31)  [unwired: 1 in]
                    n2119 = call "sub vi - cycle&temp fail v6.vi"("Amps Lo?"=w3345, "Input Cluster"=w3333, "SELECT"=w3342, "Amps Hi?"=w3341, "Result In"=w3335) -> ("(FAIL) out"=w3337:cluster{"FAIL LO":dbl, "FAIL HI":dbl}, "(DISP) out"=w3340:T4, "T-RISE"=w3334:cluster{"T-RISE (L)":dbl, "T-RISE (N)":dbl}, "Result Out"=w3336:bool, "file error"=w3339:errorcluster)  [unwired: 10 in]
                    n2120 = local write "TEMP RISE LAB04-1"(w3334) -> ()
                    n2121 = local write "FAIL LAB04-1"(w3337) -> ()
                    n2122 = local write "DISP LAB04-1"(w3340) -> ()
                    n2123 = local write "RESULT LAB04-1"(w3336) -> ()
                    n2124 = local write "data file error"(w3339) -> ()
                  }
                }
              }
              frame #7 {
                # "LAB04-2"
                n2125 = case shown="True" w3350 {
                  tunnel: w3352 -> [_ w3365]
                  tunnel: w3349 -> [_ w3362]
                  tunnel: w3351 -> [_ w3361]
                  frame False {
                  }
                  frame True {
                    n2126 = local read "TEMP START LAB04-2"() -> (w3367:cluster{"TL":dbl, "TN":dbl})
                    n2127 = local read "FAIL LAB04-2"() -> (w3358:cluster{"LO":dbl, "HI":dbl})
                    n2128 = local read "TDMS LAB04-2"() -> (w3366:refnum<k34>)
                    n2129 = local read "SET LAB04-2"() -> (w3363:T5)
                    n2130 = local read "DISP LAB04-2"() -> (w3364:T4)
                    n2131 = local read "SIG LAB04-2"() -> (w3368:T2)
                    n2132 = local read "RESULT LAB04-2"() -> (w3355:bool)
                    n2133 = Bundle("FAIL LAB04-2"=w3358, "SIG LAB04-2"=w3368, "TEMP START LAB04-2"=w3367, "DISP LAB04-2"=w3364, "SET LAB04-2"=w3363, "TDMS LAB04-2"=w3366) -> (w3353:T32)  [unwired: 1 in]
                    n2134 = call "sub vi - cycle&temp fail v6.vi"("Amps Lo?"=w3365, "Input Cluster"=w3353, "SELECT"=w3362, "Amps Hi?"=w3361, "Result In"=w3355) -> ("(FAIL) out"=w3357:cluster{"FAIL LO":dbl, "FAIL HI":dbl}, "(DISP) out"=w3360:T4, "T-RISE"=w3354:cluster{"T-RISE (L)":dbl, "T-RISE (N)":dbl}, "Result Out"=w3356:bool, "file error"=w3359:errorcluster)  [unwired: 10 in]
                    n2135 = local write "TEMP RISE LAB04-2"(w3354) -> ()
                    n2136 = local write "FAIL LAB04-2"(w3357) -> ()
                    n2137 = local write "DISP LAB04-2"(w3360) -> ()
                    n2138 = local write "RESULT LAB04-2"(w3356) -> ()
                    n2139 = local write "data file error"(w3359) -> ()
                  }
                }
              }
              frame #8 {
                # "LAB05-1"
                n2140 = case shown="True" w3370 {
                  tunnel: w3372 -> [_ w3385]
                  tunnel: w3369 -> [_ w3382]
                  tunnel: w3371 -> [_ w3381]
                  frame False {
                  }
                  frame True {
                    n2141 = local read "TEMP START LAB05-1"() -> (w3387:cluster{"TL":dbl, "TN":dbl})
                    n2142 = local read "FAIL LAB05-1"() -> (w3378:cluster{"LO":dbl, "HI":dbl})
                    n2143 = local read "TDMS LAB05-1"() -> (w3386:refnum<k34>)
                    n2144 = local read "SET LAB05-1"() -> (w3383:T5)
                    n2145 = local read "DISP LAB05-1"() -> (w3384:T4)
                    n2146 = local read "SIG LAB05-1"() -> (w3388:T2)
                    n2147 = local read "RESULT LAB05-1"() -> (w3375:bool)
                    n2148 = Bundle("FAIL LAB05-1"=w3378, "SIG LAB05-1"=w3388, "TEMP START LAB05-1"=w3387, "DISP LAB05-1"=w3384, "SET LAB05-1"=w3383, "TDMS LAB05-1"=w3386) -> (w3373:T33)  [unwired: 1 in]
                    n2149 = call "sub vi - cycle&temp fail v6.vi"("Amps Lo?"=w3385, "Input Cluster"=w3373, "SELECT"=w3382, "Amps Hi?"=w3381, "Result In"=w3375) -> ("(FAIL) out"=w3377:cluster{"FAIL LO":dbl, "FAIL HI":dbl}, "(DISP) out"=w3380:T4, "T-RISE"=w3374:cluster{"T-RISE (L)":dbl, "T-RISE (N)":dbl}, "Result Out"=w3376:bool, "file error"=w3379:errorcluster)  [unwired: 10 in]
                    n2150 = local write "TEMP RISE LAB05-1"(w3374) -> ()
                    n2151 = local write "FAIL LAB05-1"(w3377) -> ()
                    n2152 = local write "DISP LAB05-1"(w3380) -> ()
                    n2153 = local write "RESULT LAB05-1"(w3376) -> ()
                    n2154 = local write "data file error"(w3379) -> ()
                  }
                }
              }
              frame #9 {
                # "LAB05-2"
                n2155 = case shown="True" w3390 {
                  tunnel: w3392 -> [_ w3405]
                  tunnel: w3389 -> [_ w3402]
                  tunnel: w3391 -> [_ w3401]
                  frame False {
                  }
                  frame True {
                    n2156 = local read "TEMP START LAB05-2"() -> (w3407:cluster{"TL":dbl, "TN":dbl})
                    n2157 = local read "FAIL LAB05-2"() -> (w3398:cluster{"LO":dbl, "HI":dbl})
                    n2158 = local read "TDMS LAB05-2"() -> (w3406:refnum<k34>)
                    n2159 = local read "SET LAB05-2"() -> (w3403:T5)
                    n2160 = local read "DISP LAB05-2"() -> (w3404:T4)
                    n2161 = local read "SIG LAB05-2"() -> (w3408:T2)
                    n2162 = local read "RESULT LAB05-2"() -> (w3395:bool)
                    n2163 = Bundle("FAIL LAB05-2"=w3398, "SIG LAB05-2"=w3408, "TEMP START LAB05-2"=w3407, "DISP LAB05-2"=w3404, "SET LAB05-2"=w3403, "TDMS LAB05-2"=w3406) -> (w3393:T34)  [unwired: 1 in]
                    n2164 = call "sub vi - cycle&temp fail v6.vi"("Amps Lo?"=w3405, "Input Cluster"=w3393, "SELECT"=w3402, "Amps Hi?"=w3401, "Result In"=w3395) -> ("(FAIL) out"=w3397:cluster{"FAIL LO":dbl, "FAIL HI":dbl}, "(DISP) out"=w3400:T4, "T-RISE"=w3394:cluster{"T-RISE (L)":dbl, "T-RISE (N)":dbl}, "Result Out"=w3396:bool, "file error"=w3399:errorcluster)  [unwired: 10 in]
                    n2165 = local write "TEMP RISE LAB05-2"(w3394) -> ()
                    n2166 = local write "FAIL LAB05-2"(w3397) -> ()
                    n2167 = local write "DISP LAB05-2"(w3400) -> ()
                    n2168 = local write "RESULT LAB05-2"(w3396) -> ()
                    n2169 = local write "data file error"(w3399) -> ()
                  }
                }
              }
            }
          }
          frame #14 {
            # "run calibration routine"
            n2170 = local read "CALIBRATE"() -> (w3409:bool)
            n2171 = case shown="True" w3409 {
              frame False {
              }
              frame True {
                n2172 = stacked-sequence {
                  seq-local: [w3410 _ _] -> [_ w3412 _]
                  frame #0 {
                    n2173 = call "CALIBRATION PASSWORD"() -> ("PASSWORD"=w3410:string)  [unwired: 17 in, 2 out]
                  }
                  frame #1 {
                    n2174 = Equal?(x=w3412, y="7777") -> (x = y?=w3411:bool)
                    n2175 = case shown="True" w3411 {
                      frame False {
                      }
                      frame True {
                        n2176 = stacked-sequence {
                          frame #0 {
                            n2177 = call "sub vi - calibration v1.vi"() -> ()  [unwired: 12 in]
                          }
                          frame #1 {
                            n2178 = call "sub vi - get calibration values v1.vi"() -> ("LAB01 (CAL)"=w3418:T7, "LAB02 (CAL)"=w3417:T8, "LAB03 (CAL)"=w3416:T7, "LAB04 (CAL)"=w3415:T7, "calibration file error out"=w3419:errorcluster, "LAB05 (CAL)"=w3414:T7)  [unwired: 10 in]
                            n2179 = local write "calibration file error out"(w3419) -> ()
                            n2180 = local write "CAL LAB04"(w3415) -> ()
                            n2181 = local write "CAL LAB05"(w3414) -> ()
                            n2182 = local write "CAL LAB01"(w3418) -> ()
                            n2183 = local write "CAL LAB02"(w3417) -> ()
                            n2184 = local write "CAL LAB03"(w3416) -> ()
                          }
                        }
                      }
                    }
                  }
                  frame #2 {
                    n2185 = local write "CALIBRATE"(FALSE) -> ()
                  }
                }
              }
            }
          }
          frame #15 {
            # "save certain settings to file"
            n2186 = String To Path(string="c:\\crabtree\\Set Up\\") -> (path=w3422:path)
            n2187 = Build Path(base path=w3422, name or relative path="settings.bin") -> (appended path=w3424:path)
            n2188 = Build Path(base path=w3422, name or relative path="mail.bin") -> (appended path=w3421:path)
            n2189 = Create Folder(path (use dialog)=w3422) -> (error out=w3427:errorcluster)  [unwired: 2 in, 2 out]
            n2190 = call <vilib>:"Clear Errors.vi"("error in (no error)"=w3427) -> ()  [unwired: 6 in, 1 out]
            n2191 = stacked-sequence {
              seq-local: [w3429 _] -> [_ w3442]
              tunnel: w3424 -> [_ w3443]
              tunnel: w3421 -> [_ w3441]
              frame #0 {
                n2192 = local read "C drive data root dir"() -> (w3428:path)
                n2193 = local read "Network Directory"() -> (w3434:path)
                n2194 = local read "SET LAB05-2"() -> (w3433:T5)
                n2195 = local read "SET LAB05-1"() -> (w3432:T5)
                n2196 = local read "SET LAB04-2"() -> (w3431:T5)
                n2197 = local read "SET LAB03-2"() -> (w3435:T5)
                n2198 = local read "SET LAB04-1"() -> (w3430:T5)
                n2199 = local read "SET LAB03-1"() -> (w3436:T5)
                n2200 = local read "SET LAB02-2"() -> (w3437:T5)
                n2201 = local read "SET LAB02-1"() -> (w3438:T5)
                n2202 = local read "SET LAB01-2"() -> (w3439:T5)
                n2203 = local read "SET LAB01-1"() -> (w3440:T5)
                n2204 = Bundle("SET LAB01-1"=w3440, "SET LAB01-2"=w3439, "SET LAB02-1"=w3438, "SET LAB02-2"=w3437, "SET LAB03-1"=w3436, "SET LAB03-2"=w3435, "SET LAB04-1"=w3430, "SET LAB04-2"=w3431, "SET LAB05-1"=w3432, "SET LAB05-2"=w3433, "Network Directory"=w3434, "C drive data root dir"=w3428) -> (w3429:T17)  [unwired: 1 in]
              }
              frame #1 {
                n2205 = event shown="[1] \"SET LAB01-1\", \"SET LAB01-2\", \"SET LAB02-1\", \"SET LAB02-2\", \"SET LAB03-1\", \"SET LAB03-2\", \"SET LAB04-1\", \"SET LAB04-2\", \"SET LAB05-1\", \"SET LAB05-2\", \"Network Directory\", \"C drive data root dir\": Value Change" {
                  selector: _ -> [_ _ _]
                  dyn-events: _ -> [_ _ _]
                  timeout: 10.0 -> [_ _ _]
                  tunnel: w3443 -> [_ w3445 _]
                  tunnel: w3442 -> [_ w3446 _]
                  tunnel: w3441 -> [_ _ w3457]
                  event Timeout {
                    n2206 = event-data() -> ()  [unwired: 1 in, 3 out]
                  }
                  event "SET LAB01-1", "SET LAB01-2", "SET LAB02-1", "SET LAB02-2", "SET LAB03-1", "SET LAB03-2", "SET LAB04-1", "SET LAB04-2", "SET LAB05-1", "SET LAB05-2", "Network Directory", "C drive data root dir": Value Change {
                    n2207 = event-data() -> ()  [unwired: 1 in, 6 out]
                    n2208 = Open/Create/Replace File(file path (use dialog)=w3445, operation (0:open)=T16."replace or create") -> (refnum out=w3451:refnum<file>, error out=w3450:errorcluster)  [unwired: 4 in, 1 out]
                    n2209 = Write to Binary File(file (use dialog)=w3451, data=w3446, error in=w3450) -> (refnum out=w3449:refnum<file>, error out=w3448:errorcluster)  [unwired: 3 in, 1 out]
                    n2210 = Close File(refnum=w3449, error in=w3448) -> (error out=w3447:errorcluster)  [unwired: 1 out]
                    n2211 = local write "data file error"(w3447) -> ()
                  }
                  event "MAIL SETTINGS.OUT SERVER ADDRESS", "MAIL SETTINGS.FROM ACCOUNT", "MAIL SETTINGS.USER NAME", "MAIL SETTINGS.PASSWORD", "Auto Mail Send", "TO (string):": Value Change {
                    n2212 = event-data() -> ()  [unwired: 1 in, 6 out]
                    n2213 = local read "MAIL SETTINGS"() -> (w3456:T6)
                    n2214 = local read "Auto Mail Send"() -> (w3454:bool)
                    n2215 = local read "TO (string):"() -> (w3453:string)
                    n2216 = Open/Create/Replace File(file path (use dialog)=w3457, operation (0:open)=T16."replace or create") -> (refnum out=w3462:refnum<file>, error out=w3461:errorcluster)  [unwired: 4 in, 1 out]
                    n2217 = Bundle("MAIL SETTINGS"=w3456, "Auto Mail Send"=w3454, "TO (string):"=w3453) -> (w3455:T35)  [unwired: 1 in]
                    n2218 = Write to Binary File(file (use dialog)=w3462, data=w3455, error in=w3461) -> (refnum out=w3460:refnum<file>, error out=w3459:errorcluster)  [unwired: 3 in, 1 out]
                    n2219 = Close File(refnum=w3460, error in=w3459) -> (error out=w3458:errorcluster)  [unwired: 1 out]
                    n2220 = local write "data file error"(w3458) -> ()
                  }
                }
              }
            }
          }
          frame #16 {
            # "mail control"
            n2221 = local read "MAIL SETTINGS"() -> (w3479:T6)
            n2222 = local read "Auto Mail Send"() -> (w3465:bool)
            n2223 = Unbundle(w3479) -> ("OUT SERVER ADDRESS"=w3478:string, "FROM ACCOUNT"=w3477:string, "TEST MAIL"=w3476:bool)  [unwired: 4 out]
            n2224 = stacked-sequence {
              tunnel: "TO (string):" -> [_ w3518]
              tunnel: w3479 -> [w3484 w3517]
              tunnel: w3478 -> [w3483 w3516]
              tunnel: w3477 -> [w3482 w3515]
              tunnel: w3476 -> [w3481 _]
              tunnel: w3465 -> [_ w3514]
              tunnel: w3475 -> [_ w3513]
              tunnel: w3474 -> [_ w3512]
              tunnel: w3473 -> [_ w3511]
              tunnel: w3472 -> [_ w3510]
              tunnel: w3471 -> [_ w3509]
              tunnel: w3470 -> [_ w3508]
              tunnel: w3469 -> [_ w3507]
              tunnel: w3468 -> [_ w3506]
              tunnel: w3467 -> [_ w3505]
              tunnel: w3466 -> [_ w3504]
              tunnel: "TO (string):" -> [w3480 _]
              frame #0 {
                # "mail test"
                n2225 = case shown="True" w3481 {
                  tunnel: w3484 -> [_ w3488]
                  tunnel: w3480 -> [_ w3487]
                  tunnel: w3483 -> [_ w3486]
                  tunnel: w3482 -> [_ w3485]
                  frame False {
                  }
                  frame True {
                    n2226 = stacked-sequence {
                      seq-local: [_ _ w3498 _] -> [_ _ _ w3499]
                      tunnel: w3488 -> [w3491 _ _ w3503]
                      tunnel: w3487 -> [_ _ w3496 _]
                      tunnel: w3486 -> [_ _ w3494 _]
                      tunnel: w3485 -> [_ _ w3495 _]
                      frame #0 {
                        n2227 = Bundle(cluster=w3491, "TEST MAIL STATUS"="TEST START") -> (w3489:T6)  [unwired: 6 in]
                        n2228 = local write "MAIL SETTINGS"(w3489) -> ()
                      }
                      frame #1 {
                        n2229 = Wait (ms)(milliseconds to wait=500) -> ()  [unwired: 1 out]
                      }
                      frame #2 {
                        n2230 = call "sub vi - send mail with attach v5.vi"("TO:"=w3496, "subject"="MAIL TEST FROM LAB PANEL", "from"=w3495, "out going server"=w3494, "message"="TEST MESSAGE") -> ("error out"=w3498:errorcluster)  [unwired: 10 in]
                      }
                      frame #3 {
                        n2231 = Bundle(cluster=w3503, "TEST MAIL"=FALSE, "TEST MAIL STATUS"="TEST END", "mail error"=w3499) -> (w3501:T6)  [unwired: 4 in]
                        n2232 = local write "MAIL SETTINGS"(w3501) -> ()
                      }
                    }
                  }
                }
              }
              frame #1 {
                # "mail report"
                n2233 = stacked-sequence {
                  seq-local: [_ w3583 _ _] -> [_ _ _ w3751]
                  seq-local: [_ _ w3664 _] -> [_ _ _ w3741]
                  seq-local: [w3528 _ _ _] -> [_ w3577 _ _]
                  seq-local: [w3527 _ _ _] -> [_ w3576 _ _]
                  seq-local: [w3525 _ _ _] -> [_ w3574 _ _]
                  seq-local: [w3526 _ _ _] -> [_ w3575 _ _]
                  seq-local: [w3524 _ _ _] -> [_ w3573 _ _]
                  seq-local: [w3523 _ _ _] -> [_ w3568 _ _]
                  seq-local: [w3522 _ _ _] -> [_ w3569 _ _]
                  seq-local: [w3521 _ _ _] -> [_ w3570 _ _]
                  seq-local: [w3520 _ _ _] -> [_ w3571 _ _]
                  seq-local: [w3519 _ _ _] -> [_ w3572 _ _]
                  tunnel: w3518 -> [_ _ _ w3752]
                  tunnel: w3517 -> [_ _ _ w3735]
                  tunnel: w3516 -> [_ _ _ w3749]
                  tunnel: w3515 -> [_ _ _ w3748]
                  tunnel: w3514 -> [w3559 _ _ w3743]
                  tunnel: w3513 -> [_ _ w3694 _]
                  tunnel: w3512 -> [_ _ w3691 _]
                  tunnel: w3511 -> [_ _ w3690 _]
                  tunnel: w3510 -> [_ _ w3689 _]
                  tunnel: w3509 -> [_ _ w3688 _]
                  tunnel: w3508 -> [_ _ w3687 _]
                  tunnel: w3507 -> [_ _ w3686 _]
                  tunnel: w3506 -> [_ _ w3685 _]
                  tunnel: w3505 -> [_ _ w3684 _]
                  tunnel: w3504 -> [_ _ w3683 _]
                  frame #0 {
                    n2234 = case shown="False" w3559 {
                      frame False {
                        n2235 = local write "mail control"("") -> ()
                      }
                      frame True {
                      }
                    }
                    n2236 = local read "SET LAB01-1"() -> (w3558:T5)
                    n2237 = local read "SET LAB01-2"() -> (w3557:T5)
                    n2238 = local read "SET LAB02-1"() -> (w3556:T5)
                    n2239 = local read "SET LAB02-2"() -> (w3555:T5)
                    n2240 = local read "SET LAB03-1"() -> (w3554:T5)
                    n2241 = local read "SET LAB04-1"() -> (w3552:T5)
                    n2242 = local read "SET LAB05-1"() -> (w3550:T5)
                    n2243 = local read "SET LAB03-2"() -> (w3553:T5)
                    n2244 = local read "SET LAB04-2"() -> (w3551:T5)
                    n2245 = local read "SET LAB05-2"() -> (w3549:T5)
                    n2246 = Unbundle(w3554) -> ("DESCRIPTION"=w3534:string)  [unwired: 4 out]
                    n2247 = Unbundle(w3553) -> ("DESCRIPTION"=w3533:string)  [unwired: 4 out]
                    n2248 = Unbundle(w3552) -> ("DESCRIPTION"=w3532:string)  [unwired: 4 out]
                    n2249 = Unbundle(w3549) -> ("DESCRIPTION"=w3529:string)  [unwired: 4 out]
                    n2250 = Unbundle(w3555) -> ("DESCRIPTION"=w3535:string)  [unwired: 4 out]
                    n2251 = Unbundle(w3551) -> ("DESCRIPTION"=w3531:string)  [unwired: 4 out]
                    n2252 = Unbundle(w3558) -> ("DESCRIPTION"=w3547:string)  [unwired: 4 out]
                    n2253 = Unbundle(w3556) -> ("DESCRIPTION"=w3536:string)  [unwired: 4 out]
                    n2254 = Unbundle(w3550) -> ("DESCRIPTION"=w3530:string)  [unwired: 4 out]
                    n2255 = Unbundle(w3557) -> ("DESCRIPTION"=w3537:string)  [unwired: 4 out]
                    n2256 = Concatenate Strings("[LAB05-1/", w3529) -> (w3519:string)
                    n2257 = Concatenate Strings("[LAB05-2/", w3530) -> (w3520:string)
                    n2258 = Concatenate Strings("[LAB04-2/", w3531) -> (w3521:string)
                    n2259 = Concatenate Strings("[LAB03-2/", w3533) -> (w3523:string)
                    n2260 = Concatenate Strings("[LAB04-1/", w3532) -> (w3522:string)
                    n2261 = Concatenate Strings("[LAB03-1/", w3534) -> (w3524:string)
                    n2262 = Concatenate Strings("[LAB01-2/", w3537) -> (w3527:string)
                    n2263 = Concatenate Strings("[LAB02-2/", w3535) -> (w3525:string)
                    n2264 = Concatenate Strings("[LAB01-1/", w3547) -> (w3528:string)
                    n2265 = Concatenate Strings("[LAB02-1/", w3536) -> (w3526:string)
                  }
                  frame #1 {
                    w3581 = "/"
                    w3582 = 2.0
                    n2266 = local read "DISP LAB01-2"() -> (w3662:T4)
                    n2267 = local read "DISP LAB01-1"() -> (w3663:T4)
                    n2268 = local read "DISP LAB02-1"() -> (w3661:T4)
                    n2269 = local read "DISP LAB03-2"() -> (w3658:T4)
                    n2270 = local read "DISP LAB02-2"() -> (w3660:T4)
                    n2271 = local read "DISP LAB03-1"() -> (w3659:T4)
                    n2272 = local read "DISP LAB04-2"() -> (w3656:T4)
                    n2273 = local read "DISP LAB04-1"() -> (w3657:T4)
                    n2274 = local read "DISP LAB05-1"() -> (w3655:T4)
                    n2275 = local read "DISP LAB05-2"() -> (w3654:T4)
                    n2276 = Unbundle(w3662) -> ("CYCLE"=w3646:dbl, "MINS"=w3645:dbl, "STATUS"=w3642:string)
                    n2277 = Unbundle(w3663) -> ("CYCLE"=w3651:dbl, "MINS"=w3650:dbl, "STATUS"=w3647:string)
                    n2278 = Unbundle(w3661) -> ("CYCLE"=w3639:dbl, "MINS"=w3638:dbl, "STATUS"=w3637:string)
                    n2279 = Unbundle(w3658) -> ("CYCLE"=w3626:dbl, "MINS"=w3625:dbl, "STATUS"=w3622:string)
                    n2280 = Unbundle(w3659) -> ("CYCLE"=w3631:dbl, "MINS"=w3630:dbl, "STATUS"=w3627:string)
                    n2281 = Unbundle(w3660) -> ("CYCLE"=w3636:dbl, "MINS"=w3635:dbl, "STATUS"=w3632:string)
                    n2282 = Unbundle(w3657) -> ("CYCLE"=w3621:dbl, "MINS"=w3620:dbl, "STATUS"=w3617:string)
                    n2283 = Unbundle(w3656) -> ("CYCLE"=w3616:dbl, "MINS"=w3615:dbl, "STATUS"=w3612:string)
                    n2284 = Unbundle(w3655) -> ("CYCLE"=w3611:dbl, "MINS"=w3610:dbl, "STATUS"=w3607:string)
                    n2285 = Unbundle(w3654) -> ("CYCLE"=w3653:dbl, "MINS"=w3652:dbl, "STATUS"=w3604:string)
                    n2286 = Number To Decimal String(number=w3639) -> (decimal integer string=w3641:string)  [unwired: 1 in]
                    n2287 = Number To Decimal String(number=w3636) -> (decimal integer string=w3634:string)  [unwired: 1 in]
                    n2288 = Number To Decimal String(number=w3631) -> (decimal integer string=w3629:string)  [unwired: 1 in]
                    n2289 = Number To Decimal String(number=w3646) -> (decimal integer string=w3644:string)  [unwired: 1 in]
                    n2290 = Number To Decimal String(number=w3626) -> (decimal integer string=w3624:string)  [unwired: 1 in]
                    n2291 = Number To Decimal String(number=w3651) -> (decimal integer string=w3649:string)  [unwired: 1 in]
                    n2292 = Number To Decimal String(number=w3653) -> (decimal integer string=w3606:string)  [unwired: 1 in]
                    n2293 = Number To Decimal String(number=w3621) -> (decimal integer string=w3619:string)  [unwired: 1 in]
                    n2294 = Number To Decimal String(number=w3616) -> (decimal integer string=w3614:string)  [unwired: 1 in]
                    n2295 = Number To Decimal String(number=w3611) -> (decimal integer string=w3609:string)  [unwired: 1 in]
                    n2296 = Number To Fractional String(number=w3638, precision (6)=w3582) -> (F-format string=w3640:string)  [unwired: 2 in]
                    n2297 = Number To Fractional String(number=w3625, precision (6)=w3582) -> (F-format string=w3623:string)  [unwired: 2 in]
                    n2298 = Number To Fractional String(number=w3635, precision (6)=w3582) -> (F-format string=w3633:string)  [unwired: 2 in]
                    n2299 = Number To Fractional String(number=w3630, precision (6)=w3582) -> (F-format string=w3628:string)  [unwired: 2 in]
                    n2300 = Number To Fractional String(number=w3615, precision (6)=w3582) -> (F-format string=w3613:string)  [unwired: 2 in]
                    n2301 = Number To Fractional String(number=w3620, precision (6)=w3582) -> (F-format string=w3618:string)  [unwired: 2 in]
                    n2302 = Number To Fractional String(number=w3645, precision (6)=w3582) -> (F-format string=w3643:string)  [unwired: 2 in]
                    n2303 = Number To Fractional String(number=w3610, precision (6)=w3582) -> (F-format string=w3608:string)  [unwired: 2 in]
                    n2304 = Number To Fractional String(number=w3650, precision (6)=w3582) -> (F-format string=w3648:string)  [unwired: 2 in]
                    n2305 = Number To Fractional String(number=w3652, precision (6)=w3582) -> (F-format string=w3605:string)  [unwired: 2 in]
                    n2306 = Concatenate Strings(w3581, w3624, w3581, w3623, w3581, w3622) -> (w3598:string)
                    n2307 = Concatenate Strings(w3581, w3619, w3581, w3618, w3581, w3617) -> (w3597:string)
                    n2308 = Concatenate Strings(w3581, w3614, w3581, w3613, w3581, w3612) -> (w3596:string)
                    n2309 = Concatenate Strings(w3581, w3609, w3581, w3608, w3581, w3607) -> (w3595:string)
                    n2310 = Concatenate Strings(w3581, w3606, w3581, w3605, w3581, w3604) -> (w3594:string)
                    n2311 = Concatenate Strings(w3581, w3649, w3581, w3648, w3581, w3647) -> (w3603:string)
                    n2312 = Concatenate Strings(w3581, w3629, w3581, w3628, w3581, w3627) -> (w3599:string)
                    n2313 = Concatenate Strings(w3581, w3644, w3581, w3643, w3581, w3642) -> (w3602:string)
                    n2314 = Concatenate Strings(w3581, w3641, w3581, w3640, w3581, w3637) -> (w3601:string)
                    n2315 = Concatenate Strings(w3581, w3634, w3581, w3633, w3581, w3632) -> (w3600:string)
                    n2316 = Concatenate Strings("]", "\r") -> (w3578:string)
                    n2317 = Concatenate Strings(w3573, w3599, w3578) -> (w3589:string)
                    n2318 = Concatenate Strings(w3575, w3601, w3578) -> (w3591:string)
                    n2319 = Concatenate Strings(w3574, w3600, w3578) -> (w3590:string)
                    n2320 = Concatenate Strings(w3570, w3596, w3578) -> (w3586:string)
                    n2321 = Concatenate Strings(w3571, w3595, w3578) -> (w3587:string)
                    n2322 = Concatenate Strings(w3569, w3597, w3578) -> (w3585:string)
                    n2323 = Concatenate Strings(w3568, w3598, w3578) -> (w3584:string)
                    n2324 = Concatenate Strings(w3572, w3594, w3578) -> (w3588:string)
                    n2325 = Concatenate Strings(w3576, w3602, w3578) -> (w3592:string)
                    n2326 = Concatenate Strings(w3577, w3603, w3578) -> (w3593:string)
                    n2327 = Concatenate Strings(w3593, w3592, w3591, w3590, w3589, w3584, w3585, w3586, w3587, w3588) -> (w3561:string)
                    n2328 = Concatenate Strings("[PANEL/", "DESC/", "CYCLES/", "MINS/", "STATUS]", "\r", w3561) -> (w3583:string)
                    "MAIL REPORT" <- w3583
                  }
                  frame #2 {
                    w3692 = "END"
                    n2329 = local read "mail control"() -> (w3693:string)
                    n2330 = case shown="False" w3688 {
                      tunnel: w3693 -> [w3717 _]
                      tunnel: w3692 -> [w3716 _]
                      tunnel: [w3715 FALSE] -> w3678
                      frame False {
                        n2331 = Equal?(x=w3717, y=w3716) -> (x = y?=w3715:bool)
                      }
                      frame True {
                      }
                    }
                    n2332 = case shown="False" w3694 {
                      tunnel: w3693 -> [w3733 _]
                      tunnel: w3692 -> [w3732 _]
                      tunnel: [w3731 FALSE] -> w3682
                      frame False {
                        n2333 = Equal?(x=w3733, y=w3732) -> (x = y?=w3731:bool)
                      }
                      frame True {
                      }
                    }
                    n2334 = case shown="False" w3691 {
                      tunnel: w3693 -> [w3729 _]
                      tunnel: w3692 -> [w3728 _]
                      tunnel: [w3727 FALSE] -> w3681
                      frame False {
                        n2335 = Equal?(x=w3729, y=w3728) -> (x = y?=w3727:bool)
                      }
                      frame True {
                      }
                    }
                    n2336 = case shown="False" w3689 {
                      tunnel: w3693 -> [w3721 _]
                      tunnel: w3692 -> [w3720 _]
                      tunnel: [w3719 FALSE] -> w3679
                      frame False {
                        n2337 = Equal?(x=w3721, y=w3720) -> (x = y?=w3719:bool)
                      }
                      frame True {
                      }
                    }
                    n2338 = case shown="False" w3690 {
                      tunnel: w3693 -> [w3725 _]
                      tunnel: w3692 -> [w3724 _]
                      tunnel: [w3723 FALSE] -> w3680
                      frame False {
                        n2339 = Equal?(x=w3725, y=w3724) -> (x = y?=w3723:bool)
                      }
                      frame True {
                      }
                    }
                    n2340 = Or(x=w3680, y=w3679) -> (x .or. y?=w3671:bool)
                    n2341 = Or(x=w3682, y=w3681) -> (x .or. y?=w3672:bool)
                    n2342 = Or(x=w3672, y=w3671) -> (x .or. y?=w3667:bool)
                    n2343 = case shown="False" w3684 {
                      tunnel: w3693 -> [w3701 _]
                      tunnel: w3692 -> [w3700 _]
                      tunnel: [w3699 FALSE] -> w3673
                      frame False {
                        n2344 = Equal?(x=w3701, y=w3700) -> (x = y?=w3699:bool)
                      }
                      frame True {
                      }
                    }
                    n2345 = case shown="False" w3683 {
                      tunnel: w3693 -> [w3697 _]
                      tunnel: w3692 -> [w3696 _]
                      tunnel: [w3695 FALSE] -> w3677
                      frame False {
                        n2346 = Equal?(x=w3697, y=w3696) -> (x = y?=w3695:bool)
                      }
                      frame True {
                      }
                    }
                    n2347 = case shown="False" w3685 {
                      tunnel: w3693 -> [w3705 _]
                      tunnel: w3692 -> [w3704 _]
                      tunnel: [w3703 FALSE] -> w3674
                      frame False {
                        n2348 = Equal?(x=w3705, y=w3704) -> (x = y?=w3703:bool)
                      }
                      frame True {
                      }
                    }
                    n2349 = case shown="False" w3687 {
                      tunnel: w3693 -> [w3713 _]
                      tunnel: w3692 -> [w3712 _]
                      tunnel: [w3711 FALSE] -> w3676
                      frame False {
                        n2350 = Equal?(x=w3713, y=w3712) -> (x = y?=w3711:bool)
                      }
                      frame True {
                      }
                    }
                    n2351 = case shown="False" w3686 {
                      tunnel: w3693 -> [w3709 _]
                      tunnel: w3692 -> [w3708 _]
                      tunnel: [w3707 FALSE] -> w3675
                      frame False {
                        n2352 = Equal?(x=w3709, y=w3708) -> (x = y?=w3707:bool)
                      }
                      frame True {
                      }
                    }
                    n2353 = Or(x=w3676, y=w3675) -> (x .or. y?=w3670:bool)
                    n2354 = Or(x=w3674, y=w3673) -> (x .or. y?=w3669:bool)
                    n2355 = Or(x=w3677, y=w3678) -> (x .or. y?=w3665:bool)
                    n2356 = Or(x=w3670, y=w3669) -> (x .or. y?=w3668:bool)
                    n2357 = Or(x=w3667, y=w3668) -> (x .or. y?=w3666:bool)
                    n2358 = Or(x=w3666, y=w3665) -> (x .or. y?=w3664:bool)
                  }
                  frame #3 {
                    n2359 = local read "on loops"() -> (w3747:dbl)
                    n2360 = local read "jig cycle"() -> (w3744:dbl)
                    n2361 = local read "Send Mail Now"() -> (w3738:bool)
                    n2362 = Add(x=w3747, y=3.0) -> (x+y=w3745:dbl)
                    n2363 = Equal?(x=w3744, y=w3745) -> (x = y?=w3739:bool)
                    n2364 = And(x=w3739, y=w3738) -> (x .and. y?=w3737:bool)
                    n2365 = And(x=w3743, y=w3739) -> (x .and. y?=w3742:bool)
                    n2366 = And(x=w3742, y=w3741) -> (x .and. y?=w3740:bool)
                    n2367 = Or(x=w3740, y=w3737) -> (x .or. y?=w3736:bool)
                    n2368 = case shown="True" w3736 {
                      tunnel: w3752 -> [_ w3758]
                      tunnel: w3751 -> [_ w3757]
                      tunnel: "Lab Panel Test Status" -> [_ w3756]
                      tunnel: w3749 -> [_ w3755]
                      tunnel: w3748 -> [_ w3754]
                      tunnel: w3735 -> [_ w3753]
                      frame False {
                      }
                      frame True {
                        n2369 = stacked-sequence {
                          tunnel: w3758 -> [w3766 _]
                          tunnel: w3757 -> [w3765 _]
                          tunnel: w3756 -> [w3764 _]
                          tunnel: w3755 -> [w3763 _]
                          tunnel: w3754 -> [w3762 _]
                          tunnel: w3753 -> [w3761 _]
                          frame #0 {
                            n2370 = call "sub vi - send mail with attach v5.vi"("TO:"=w3766, "subject"=w3764, "from"=w3762, "out going server"=w3763, "message"=w3765) -> ("error out"=w3760:errorcluster)  [unwired: 10 in]
                            n2371 = Bundle(cluster=w3761, "mail error"=w3760) -> (w3759:T6)  [unwired: 6 in]
                            n2372 = local write "MAIL SETTINGS"(w3759) -> ()
                          }
                          frame #1 {
                            n2373 = local write "mail control"("") -> ()
                            n2374 = local write "Send Mail Now"(FALSE) -> ()
                          }
                        }
                      }
                    }
                  }
                }
              }
            }
          }
        }
        n2375 = node-c288() -> ()  [unwired: 1 in, 1 out]
        "loops" <- w165
        "stop2" <- "stop"
      }
      n2376 = node-c288(w142) -> ()  [unwired: 1 out]
    }
  }
